vi "main 1.18.vi"() -> ()   [LabVIEW 2020]
uses:
  subvi/Newport ESP301/Newport ESP301.lvlib
  subvi/sp_manip.llb/sp_manip_lib.lvlib
  subvi/sp_manip.llb/tcp_gateway.lvlib
  <vilib>/Utility/file.llb/Write Delimited Spreadsheet (DBL).vi
  <vilib>/Analysis/NI_AALBase.lvlib
  <vilib>/Analysis/1siggen.llb/Ramp Pattern by Samples.vi
  <vilib>/Analysis/NI_AALPro.lvlib
  <vilib>/Analysis/_algsub.llb/Real Vector Norm.vi
  subvi/ZaberTSeries/ZaberTSeries.lvlib
  <vilib>/Utility/file.llb/Write Delimited Spreadsheet (string).vi
  <userlib>/caLab/Private/Get_PV.vi
  <userlib>/caLab/Private/Put_DBL_PV.vi
  <vilib>/Utility/file.llb/Read Delimited Spreadsheet (string).vi
  subvi/ProdigyRemoteControlLib/ProdigyRemoteControl.lvlib
  <vilib>/DAQmx/create/channels.llb/DAQmx Create Channel (DI-Digital Input).vi
panel:
  out "Pics L":i32=200
  out "Waveform Chart":dbl(graph)
  out "G2 X":cluster{dbl[], "Ramp Pattern":dbl[]}(graph)={array[344 elements], "Ramp Pattern"=[0.0, 0.0, 0.0, 0.0, 0.0, 0.0, 0.0, 0.0, 0.0, 0.0, 0.0, 0.0, 0.0, 0.0, 0.0, 0.0, 0.0, 0.0, 0.0, 0.0, 0.0, 12.377241379310345, 41.64689655172414, 18.335172413793103, 0.0, 0.0, 0.0, 0.0, 0.0, 0.0, 0.0, 0.0, 0.0, 0.0, 0.0, 0.0, 0.0, 0.0, 0.0, 0.0, 0.0, 0.0, 0.0, 0.0, 0.0, 0.0, 0.0, 0.0, 0.0, 0.0, 0.0, 0.0, 0.0, 0.0, 0.0, 0.0, 0.0, 0.0, 0.0, 0.0, 0.0, 0.0, 0.0, 0.0, 0.0, 0.0, 0.0, 0.0, 0.0, 0.0, 0.0, 0.0, 0.0, 0.0, 0.0, 0.0, 0.0, 0.0, 0.0, 0.0, 0.0, 0.0, 0.0, 0.0, 0.0, 0.0, 0.0, 0.0, 0.0, 0.0, 0.0, 0.0, 0.0, 0.0, 0.0, 0.0, 0.0, 0.0, 0.0, 0.0, 0.0, 0.0, 0.0, 0.0, 0.0, 0.0, 0.0, 0.0, 0.0, 0.0, 0.0, 0.0, 0.0, 0.0, 0.0, 17.495517241379314, 48.13413793103449, 27.429999999999996, 0.0, 0.0, 0.0, 0.0, 0.0, 0.0, 0.0, 0.0, 0.0, 0.0, 0.0, 0.0, 0.0, 0.0, 0.0, 0.0, 0.0, 0.0, 0.0, 0.0, 0.0, 0.0, 0.0, 0.0, 0.0, 0.0, 0.0, 0.0, 0.0, 0.0, 0.0, 0.0, 0.0, 0.0, 0.0, 0.0, 0.0, 0.0, 0.0, 0.0, 0.0, 0.0, 0.0, 0.0, 0.0, 0.0, 0.0, 0.0, 0.0, 0.0, 0.0, 0.0, 0.0, 0.0, 0.0, 0.0, 0.0, 0.0, 0.0, 0.0, 0.0, 0.0, 0.0, 0.0, 17.760344827586206, 28.923448275862068, 17.532068965517244, 0.0, 0.0, 0.0, 0.0, 0.0, 0.0, 0.0, 0.0, 0.0, 0.0, 0.0, 0.0, 0.0, 0.0, 0.0, 0.0, 0.0, 0.0, 0.0, 0.0, 0.0, 0.0, 0.0, 0.0, 0.0, 0.0, 0.0, 0.0, 0.0, 0.0, 0.0, 0.0, 0.0, 0.0, 0.0, 0.0, 0.0, 0.0, 0.0, 0.0, 0.0, 0.0, 0.0, 0.0, 0.0, 2.201724137931034, 1.9948275862068956, 0.0, 0.0, 0.0, 0.0, 0.0, 0.0, 0.0, 0.0, 0.0, 0.0, 0.0, 0.0, 0.0, 0.0, 0.0, 0.0, 0.0, 0.0, 0.0, 0.0, 0.0, 0.0, 0.0, 0.0, 0.0, 0.0, 0.0, 0.0, 0.0, 0.0, 0.0, 0.0, 0.0, 0.0, 0.0, 0.0, 0.0, 0.0, 0.0, 0.0, 0.0, 0.0, 0.0, 0.0, 0.0, 0.0, 0.0, 0.0, 0.0, 0.0, 0.0, 0.0, 0.0, 0.0, 0.0, 0.0, 0.0, 0.0, 0.0, 0.0, 0.0, 0.0, 0.0, 0.0, 0.0, 0.0, 0.0, 0.0, 0.0, 0.0, 0.0, 0.0, 0.0, 0.0, 0.0, 0.0, 0.0, 0.0, 0.0, 0.0, 0.0, 0.0, 0.0, 0.0, 0.0, 0.0, 0.0, 0.0, 0.0, 0.0, 0.0, 0.0, 0.0, 0.0, 0.0, 0.0, 0.0, 0.0, 0.0, 0.0, 0.0, 0.0, 0.0, 0.0, 0.0, 0.0, 0.0, 0.0, 0.0, 0.0, 0.0, 0.0]}
  in  "reset every n pics":bool=TRUE
  in  "pics2avg":i32=50
  in  "abort acq.":bool
  out "G2 Y":cluster{dbl[], "Ramp Pattern":dbl[]}(graph)={[0.0, 0.0, 0.0, 0.0, 0.0, 0.0, 0.0, 0.0, 0.0, 0.0, 0.0, 0.0, 0.0, 0.0, 0.0, 0.0, 0.0, 0.0, 0.0, 0.0, 0.0, 0.0, 0.0, 0.0, 0.0, 0.0, 0.0, 0.0, 0.0, 0.0, 0.0, 0.0, 0.0, 0.0, 0.0, 0.0, 0.0, 0.0, 0.0, 0.0, 0.0, 0.0, 0.0, 0.0, 0.0, 0.0, 0.0, 0.0, 0.0, 0.0, 0.0, 0.0, 0.0, 0.0, 0.0, 0.0, 0.0, 0.0, 0.0, 0.0, 0.0, 0.0, 0.0, 0.0, 0.0, 0.0, 0.0, 0.0, 0.0, 0.0, 0.0, 0.0, 0.0, 0.0, 0.0, 0.0, 0.0, 0.0, 0.0, 0.0, 0.0, 0.0, 0.0, 0.0, 0.0, 0.0, 0.0, 0.0, 0.0, 0.0, 0.0, 0.0, 0.0, 0.0, 0.0, 0.0, 0.0, 0.0, 0.0, 0.0, 0.0, 0.0, 0.0, 0.0, 0.0, 0.0, 0.0, 0.0, 0.0, 0.0, 0.0, 0.0, 0.0, 0.0, 0.0, 0.0, 0.0, 0.0, 0.0, 0.0, 0.0, 0.0, 0.0, 0.0, 0.0, 0.0, 0.0, 0.0, 0.0, 0.0, 0.0, 0.0, 0.0, 0.0, 0.0, 0.0, 0.0, 0.0, 0.0, 0.0, 0.0, 0.0, 0.0, 0.0, 0.0, 0.0, 0.0, 0.0, 0.0, 0.0, 0.0, 0.0, 0.0, 0.0, 0.0, 0.0, 0.0, 0.0, 0.0, 0.0, 0.0, 0.0, 0.0, 0.0, 0.0, 0.0, 0.0, 0.0, 0.0, 0.0, 0.0, 0.0, 0.0, 0.0, 0.0, 0.0, 0.0, 0.0, 0.0, 0.0, 0.0, 0.0, 0.0, 0.0, 0.0, 0.0, 0.0, 0.0, 0.0, 0.0, 0.0, 0.0, 0.0, 0.0, 0.0, 0.0, 0.0, 0.0, 0.0, 0.0, 0.0, 0.0, 0.0, 0.0, 0.0, 0.0, 0.0, 0.0, 0.0, 0.0, 0.0, 0.0, 0.0, 0.0, 0.0, 0.0, 0.0, 0.0, 0.0, 0.0, 0.0, 0.0, 0.0, 0.0, 0.0, 0.0, 0.0, 0.0, 0.0, 0.0, 0.0, 0.0, 0.0, 0.0, 0.0, 0.0, 0.0, 0.0, 0.0, 0.0, 0.0, 0.0, 0.0, 0.0, 0.0, 0.0, 0.0, 0.0, 0.0, 0.0, 0.0, 0.0, 0.0, 0.0, 0.0, 0.0], "Ramp Pattern"=[0.0, 1.003921568627451, 2.007843137254902, 3.011764705882353, 4.015686274509804, 5.019607843137255, 6.023529411764706, 7.027450980392157, 8.031372549019608, 9.035294117647059, 10.03921568627451, 11.04313725490196, 12.047058823529412, 13.050980392156863, 14.054901960784314, 15.058823529411764, 16.062745098039215, 17.066666666666666, 18.070588235294117, 19.07450980392157, 20.07843137254902, 21.08235294117647, 22.08627450980392, 23.090196078431372, 24.094117647058823, 25.098039215686274, 26.101960784313725, 27.105882352941176, 28.109803921568627, 29.113725490196078, 30.11764705882353, 31.12156862745098, 32.12549019607843, 33.129411764705885, 34.13333333333333, 35.13725490196079, 36.141176470588235, 37.14509803921569, 38.14901960784314, 39.15294117647059, 40.15686274509804, 41.16078431372549, 42.16470588235294, 43.168627450980395, 44.17254901960784, 45.1764705882353, 46.180392156862744, 47.1843137254902, 48.188235294117646, 49.1921568627451, 50.19607843137255, 51.2, 52.20392156862745, 53.207843137254905, 54.21176470588235, 55.21568627450981, 56.219607843137254, 57.22352941176471, 58.227450980392156, 59.23137254901961, 60.23529411764706, 61.23921568627451, 62.24313725490196, 63.247058823529414, 64.25098039215686, 65.25490196078431, 66.25882352941177, 67.26274509803922, 68.26666666666667, 69.27058823529411, 70.27450980392157, 71.27843137254902, 72.28235294117647, 73.28627450980392, 74.29019607843138, 75.29411764705883, 76.29803921568627, 77.30196078431372, 78.30588235294118, 79.30980392156863, 80.31372549019608, 81.31764705882352, 82.32156862745099, 83.32549019607843, 84.32941176470588, 85.33333333333333, 86.33725490196079, 87.34117647058824, 88.34509803921569, 89.34901960784313, 90.3529411764706, 91.35686274509804, 92.36078431372549, 93.36470588235294, 94.3686274509804, 95.37254901960785, 96.37647058823529, 97.38039215686274, 98.3843137254902, 99.38823529411765, 100.3921568627451, 101.39607843137254, 102.4, 103.40392156862745, 104.4078431372549, 105.41176470588235, 106.41568627450981, 107.41960784313726, 108.4235294117647, 109.42745098039215, 110.43137254901961, 111.43529411764706, 112.43921568627451, 113.44313725490196, 114.44705882352942, 115.45098039215686, 116.45490196078431, 117.45882352941176, 118.46274509803922, 119.46666666666667, 120.47058823529412, 121.47450980392156, 122.47843137254903, 123.48235294117647, 124.48627450980392, 125.49019607843137, 126.49411764705883, 127.49803921568628, 128.50196078431372, 129.50588235294117, 130.50980392156862, 131.51372549019607, 132.51764705882354, 133.521568627451, 134.52549019607844, 135.52941176470588, 136.53333333333333, 137.53725490196078, 138.54117647058823, 139.54509803921567, 140.54901960784315, 141.5529411764706, 142.55686274509804, 143.5607843137255, 144.56470588235294, 145.5686274509804, 146.57254901960783, 147.57647058823528, 148.58039215686276, 149.5843137254902, 150.58823529411765, 151.5921568627451, 152.59607843137255, 153.6, 154.60392156862744, 155.6078431372549, 156.61176470588236, 157.6156862745098, 158.61960784313726, 159.6235294117647, 160.62745098039215, 161.6313725490196, 162.63529411764705, 163.6392156862745, 164.64313725490197, 165.64705882352942, 166.65098039215687, 167.65490196078431, 168.65882352941176, 169.6627450980392, 170.66666666666666, 171.6705882352941, 172.67450980392158, 173.67843137254903, 174.68235294117648, 175.68627450980392, 176.69019607843137, 177.69411764705882, 178.69803921568626, 179.7019607843137, 180.7058823529412, 181.70980392156864, 182.71372549019608, 183.71764705882353, 184.72156862745098, 185.72549019607843, 186.72941176470587, 187.73333333333332, 188.7372549019608, 189.74117647058824, 190.7450980392157, 191.74901960784314, 192.75294117647059, 193.75686274509803, 194.76078431372548, 195.76470588235293, 196.7686274509804, 197.77254901960785, 198.7764705882353, 199.78039215686275, 200.7843137254902, 201.78823529411764, 202.7921568627451, 203.79607843137254, 204.8, 205.80392156862746, 206.8078431372549, 207.81176470588235, 208.8156862745098, 209.81960784313725, 210.8235294117647, 211.82745098039214, 212.83137254901962, 213.83529411764707, 214.8392156862745, 215.84313725490196, 216.8470588235294, 217.85098039215686, 218.8549019607843, 219.85882352941175, 220.86274509803923, 221.86666666666667, 222.87058823529412, 223.87450980392157, 224.87843137254902, 225.88235294117646, 226.8862745098039, 227.89019607843136, 228.89411764705883, 229.89803921568628, 230.90196078431373, 231.90588235294118, 232.90980392156862, 233.91372549019607, 234.91764705882352, 235.92156862745097, 236.92549019607844, 237.9294117647059, 238.93333333333334, 239.93725490196078, 240.94117647058823, 241.94509803921568, 242.94901960784313, 243.95294117647057, 244.95686274509805, 245.9607843137255, 246.96470588235294, 247.9686274509804, 248.97254901960784, 249.9764705882353, 250.98039215686273, 251.98431372549018, 252.98823529411766, 253.9921568627451, 254.99607843137255, 256.0]}
  out "ETA":timestamp=timestamp(3655133644.4615793 s since 1904-01-01) format="%<%H:%M:%S>T"
  out "acq. imgs":i32=200
  out "snap_prog":dbl(slide)=1.0 scale=0.0..1.0
  in  "BasePath":path=path "T:/trARPES/PESData"
  in  "cam_liveavg":bool=TRUE caption="live average"
  out "cam_fps":dbl=19.690658487387566 caption="FPS" format="%.1g"
  out "sideimg":dbl[][](graph)
  out "RunNumber":u16=3091
  out "sum":dbl format="%#.2g"
  out "max":dbl=22.774482758620692
  out "mainimg":dbl[][](graph)
  out "ESP_con?":bool=TRUE caption="ESP301"
  out "phoib_con?":bool caption="PHOIBOS"
  out "manip_con?":bool=TRUE caption="manipulator"
  out "cam_con?":bool caption="camera"
  in  "main_close":bool=TRUE
  in  "Tab Control":enum32{"live", "scan", "devices"}(tab)=enum."devices"
  in  "wattpilot_set":bool
  out "Readback_wattpilot":dbl=304.89
  in  "Set Powet (%)":dbl
  out "Readback":dbl=340.0
  out "In Range":bool
  in  "setpoint_set":bool
  in  "Setpoint":dbl=302.0
  out "TB":dbl=304.91
  out "TA":dbl=304.49
  in  "phoib_I_10s":dbl
  out "phoib_I_10":dbl caption="Mesh Back"
  in  "mirr_go":bool
  in  "ESP_opent0file":bool
  in  "mirr_rel":i32=1 caption="relative [steps]"
  in  "mirr_Y-":bool
  in  "mirr_Y+":bool
  in  "mirr_X+":bool
  in  "mirr_X-":bool
  in  "manip_deltas":dbl[](array[numeric])=[0.0, 0.0, 5.0, 0.0, 0.0, 0.0] caption="delta" format="%#.5g"
  in  "aq.mode":enum32{"Radio Selection 1", "Radio Selection 2"}(radio)=enum."Radio Selection 2"
  in  "dark avg":i32=100
  in  "cam_avgs":i32=20 caption="N"
  in  "ESP_delta":dbl caption="relative [mm]"
  in  "ESP_-":bool
  in  "ESP_+":bool
  in  "ESP_go":bool
  in  "ESP_dest_t":dbl=728236.1319443199 caption="[fs]"
  in  "ESP_dest":dbl=-35.84015 caption="[mm]"
  in  "ESP_set_t0":bool
  in  "phoib_I_6s":dbl=3200.0
  in  "phoib_I_5s":dbl=1700.0
  in  "phoib_I_4s":dbl=4.558
  in  "phoib_I_3s":dbl=-10.0
  in  "phoib_I_2s":dbl=35.0
  in  "phoib_I_1s":dbl=21.0
  in  "phoib_standby":bool
  in  "phoib_set":bool
  out "phoib_I_6":dbl=3200.0 caption="Screen Voltage"
  out "phoib_I_5":dbl=1500.0 caption="Detctor Voltage"
  out "phoib_I_4":dbl=4.558 caption="Work Function"
  out "phoib_I_3":dbl=-10.0 caption="Coil Current"
  out "phoib_I_2":dbl=35.0 caption="Pass Energy"
  out "phoib_I_1":dbl=21.0 caption="Kinetic Energy"
  out "Saved Positions":string[][](table)=[["ertwertwert", "-2.299945", "-2.030214", "38.900024", "50.000762", "0.000887", "-97.998082"], ["uztgugt", "-14.999451", "-13.638894", "442.380066", "13.998380", "-1.893758", "-76.305838"], ["asdf", "-14.999451", "-13.638894", "442.380066", "13.998380", "-1.893758", "-76.305838"], ["test3", "-14.999451", "-13.638894", "441.380066", "13.998380", "-1.893758", "-76.305838"]]
  in  "Save Pos":bool
  in  "Load":bool
  in  "Delete":bool
  in  "ManipRel +":bool
  in  "ManipRel -":bool
  in  "Move Abs":bool
  in  "stop manip":bool
  in  "dest":dbl[](array[numeric])=[1.794011231344732, -4.007411134769244, 35.099853515625, 337.9843004481455, 2.0, 140.61656469713384] caption="destination" format="%#.5g"
  out "axis":string[](array[string])=["x", "y", "z", "polar", "tilt", "azimut"]
  out "pos":dbl[](array[numeric])=[1.794011231344732, -4.007411134769244, 35.099853515625, 337.9843004481455, 1.998632949125299, 140.61656469713384] caption="position" format="%.5f"
  out "ESP_pos":dbl=-35.84015 caption="Position"
  out "ESP_delay":dbl=-0.3335640952092252 caption="Delay"
  out "ESP_t0":dbl=-35.8401 caption="Time Zero @"
  out "phoib_I_7":dbl=-30.0 caption="Conversion Voltage"
  in  "phoib_I_7s":dbl=-30.0
  in  "phoib_I_8s":dbl=0.0039
  in  "phoib_I_9s":dbl
  out "phoib_I_8":dbl=0.0039 caption="FD1"
  out "phoib_I_9":dbl caption="Mesh Front"
  in  "gain":bool
  in  "cam_exp":u32=50 caption="exposure [ms]"
  in  "binning":u16(ring)=2 items=["X 1", "X 2", "X 4", "X 8"]
  in  "cam_dark?":bool=TRUE caption="subtract dark?"
  in  "cam_dark":bool
  in  "cam_saveimg":bool
  in  "e-size":u8
  in  "lower threshold":i32=20
  in  "count?":bool
  in  "ROI Left":i32=1
  in  "ROI Right":i32=43
  in  "ROI Top":i32=1
  in  "ROI Bottom":i32=33
  out "moving?":bool[](array[boolean])
  out "mirr_posX":i32=1955 caption="X"
  out "mirr_posY":i32=2950 caption="Y"
  in  "mirr_dest":i32[](array[numeric])=[60782, 121383]
  out "waveplate position":dbl format="%.6g"
  out "stage2 position":dbl format="%.6g"
  in  "lens_mode":string(combo)
  in  "scan_range":string(combo)
  out "current scan 2":i32=3
  out "scan 1":dbl(slide)=1.0 scale=0.0..1.0
  in  "Tab Control 2":enum32{"setup", "data"}(tab)=enum."data"
  in  "scan_selector 2":T1(tab)
  in  "scan_manip_start 2":dbl[](array[numeric])=[1.794011231344732, -4.007411134769244, 35.099853515625, 337.9843004481455, 2.000390761745462, 140.61656469713384] caption="start position" format="%#.5g"
  in  "scan_manip_deltas 2":dbl[](array[numeric])=[0.0, 0.0, 0.0, 0.0, 1.0, 0.0] caption="direction vector\n(gets normalized)" format="%#.5g"
  in  "scan_manip_setstart 2":bool
  in  "scan_mirr_start 2":i32[](array[numeric])=[60782, 121383] caption="scan_mirr_start"
  in  "scan_mirr_deltas 2":i32[](array[numeric])=[1, 0] caption="direction vector\n(gets normalized)"
  in  "scan_mirr_setstart 2":bool
  in  "wait addional  2":dbl caption="s"
  in  "Wait for T 2":bool=TRUE
  in  "scan_volt_parameter 2":string(combo)="Kinetic Energy"
  in  "waypointsD2":string[][](table)
  in  "waypointsD1":string[][](table)=[["302", "1"], ["304", ""], ["", ""]]
  in  "load waypoints 1":bool
  in  "meas_iter":i32=1 caption="Iterations"
  in  "scan_selector":T1(tab)=enum."delay"
  in  "scan_manip_setstart":bool
  in  "scan_manip_start":dbl[](array[numeric])=[1.794011231344732, -4.007411134769244, 35.099853515625, 337.9843004481455, 2.000390761745462, 140.61656469713384] caption="start position" format="%#.5g"
  in  "scan_manip_deltas":dbl[](array[numeric])=[0.0, 0.0, 0.0, 0.0, 1.0, 0.0] caption="direction vector\n(gets normalized)" format="%#.5g"
  in  "scan_mirr_start":i32[](array[numeric])=[60782, 121383]
  in  "scan_mirr_deltas":i32[](array[numeric])=[1, 0] caption="direction vector\n(gets normalized)"
  in  "scan_mirr_setstart":bool
  in  "wait addional":dbl caption="s"
  in  "Wait for T":bool=TRUE
  in  "scan_volt_parameter":string(combo)="Kinetic Energy"
  in  "clear waypoints 1":bool
  in  "load waypoints 2":bool
  in  "clear waypoints 2":bool
  out "intensitygraph":cluster{"Array":dbl[], "Intensity Chart":dbl[]}(graph)={"Array"=[302.0, 303.0, 304.0], "Intensity Chart"=[1937.88, 12704.590000000002, 4640.840000000001]}
  out "energygraph":dbl[][](graph)=[[0.0, 0.0, 0.0, 64.28999999999999, 120.06, 0.0, 0.0, 0.0, 0.0, 0.0, 0.0, 0.0, 0.0, 0.0, 0.0, 0.0, 0.0, 0.0, 0.0, 0.0, 0.0, 0.0, 0.0, 0.0, 0.0, 0.0, 0.0, 0.0, 0.0, 0.0, 0.0, 0.0, 0.0, 0.0, 0.0, 0.0, 0.0, 0.0, 0.0, 0.0, 0.0, 0.0, 0.0, 0.0, 0.0, 0.0, 0.0, 0.0, 0.0, 384.53999999999996, 1103.3799999999999, 448.21000000000004, 0.0, 0.0, 0.0, 0.0, 0.0, 0.0, 0.0, 0.0, 0.0, 0.0, 0.0, 0.0, 0.0, 0.0, 0.0, 0.0, 0.0, 120.82, 0.0, 261.04, 195.1, 253.87, 199.70999999999998, 127.75, 87.50999999999999, 0.0, 52.54, 0.0, 0.0, 51.78, 55.73, 0.0, 0.0, 0.0, 0.0, 0.0, 0.0, 0.0, 0.0, 0.0, 0.0, 0.0, 0.0, 0.0, 0.0, 0.0, 0.0, 0.0, 0.0, 0.0, 0.0, 0.0, 0.0, 0.0, 0.0, 0.0, 0.0, 0.0, 0.0, 0.0, 0.0, 332.90999999999997, 1106.25, 934.74, 0.0, 156.76, 62.65, 0.0, 0.0, 0.0, 0.0, 0.0, 0.0, 54.62, 0.0, 0.0, 0.0, 0.0, 0.0, 0.0, 0.0, 0.0, 0.0, 0.0, 0.0, 0.0, 0.0, 0.0, 0.0, 0.0, 0.0, 0.0, 65.85, 165.75, 0.0, 0.0, 0.0, 0.0, 0.0, 0.0, 0.0, 0.0, 0.0, 0.0, 0.0, 0.0, 0.0, 0.0, 0.0, 0.0, 0.0, 266.63, 591.5, 261.64, 0.0, 391.9, 527.29, 82.87, 123.75, 286.74, 151.72, 0.0, 0.0, 0.0, 0.0, 0.0, 0.0, 0.0, 0.0, 0.0, 0.0, 0.0, 0.0, 0.0, 0.0, 0.0, 0.0, 0.0, 0.0, 0.0, 396.37, 721.0900000000001, 353.5, 83.97999999999999, 104.77000000000001, 0.0, 57.83, 60.98, 182.28, 128.78, 0.0, 0.0, 0.0, 465.25, 624.3399999999999, 348.62, 0.0, 0.0, 0.0, 0.0, 0.0, 0.0, 0.0, 0.0, 0.0, 0.0, 0.0, 0.0, 119.7, 217.91, 120.56, 0.0, 0.0, 0.0, 0.0, 0.0, 0.0, 0.0, 58.89, 0.0, 0.0, 0.0, 202.23999999999998, 149.79000000000002, 0.0, 117.82, 212.51999999999998, 534.74, 421.98, 50.97, 0.0, 0.0, 0.0, 0.0, 362.15999999999997, 656.04, 265.02, 0.0, 0.0, 0.0, 0.0, 0.0, 0.0, 0.0, 0.0, 0.0, 0.0, 0.0, 0.0, 0.0, 0.0, 0.0, 0.0, 0.0, 0.0, 0.0, 0.0, 0.0, 0.0, 0.0, 0.0, 0.0, 0.0, 0.0, 0.0, 0.0, 0.0, 0.0, 0.0, 0.0, 0.0, 0.0, 0.0, 0.0, 0.0, 0.0, 0.0, 0.0, 0.0, 0.0, 0.0, 0.0, 0.0, 0.0, 0.0, 0.0, 0.0, 0.0, 0.0, 0.0, 0.0, 0.0, 0.0, 0.0, 0.0, 0.0, 0.0, 0.0, 0.0, 0.0, 0.0, 237.67999999999998, 286.08, 130.9, 0.0, 0.0, 0.0, 0.0, 0.0, 0.0, 0.0, 0.0, 0.0, 0.0, 0.0, 0.0, 0.0, 0.0, 0.0, 0.0, 0.0, 0.0, 0.0, 0.0, 0.0, 0.0, 0.0, 0.0, 0.0, 0.0, 0.0, 0.0], [0.0, 0.0, 0.0, 0.0, 0.0, 0.0, 0.0, 0.0, 0.0, 0.0, 0.0, 0.0, 0.0, 0.0, 0.0, 0.0, 0.0, 485.13, 1279.2, 234.71, 0.0, 0.0, 0.0, 0.0, 0.0, 0.0, 0.0, 0.0, 0.0, 0.0, 0.0, 0.0, 50.5, 654.4200000000001, 511.98, 0.0, 0.0, 0.0, 0.0, 0.0, 0.0, 0.0, 0.0, 0.0, 0.0, 0.0, 0.0, 0.0, 0.0, 0.0, 0.0, 0.0, 0.0, 0.0, 0.0, 0.0, 0.0, 0.0, 63.72, 693.84, 574.54, 0.0, 0.0, 0.0, 68.68, 1054.28, 1010.9499999999999, 0.0, 0.0, 0.0, 0.0, 0.0, 0.0, 0.0, 0.0, 0.0, 0.0, 0.0, 56.57, 971.76, 1333.73, 330.0, 0.0, 0.0, 0.0, 0.0, 0.0, 349.33000000000004, 292.7, 0.0, 0.0, 0.0, 0.0, 0.0, 0.0, 82.77000000000001, 1059.23, 1069.87, 156.47, 0.0, 0.0, 0.0, 0.0, 293.91, 333.47, 551.4, 493.64, 73.72999999999999, 0.0, 0.0, 0.0, 0.0, 0.0, 0.0, 0.0, 0.0, 0.0, 0.0, 0.0, 0.0, 0.0, 0.0, 286.01, 543.0699999999999, 251.94, 0.0, 0.0, 0.0, 0.0, 0.0, 233.63, 968.4799999999999, 771.53, 109.94, 0.0, 123.07, 499.72999999999996, 431.4, 0.0, 0.0, 60.85, 69.5, 0.0, 0.0, 0.0, 0.0, 0.0, 0.0, 0.0, 0.0, 0.0, 0.0, 0.0, 0.0, 0.0, 0.0, 52.01, 0.0, 0.0, 0.0, 0.0, 0.0, 0.0, 0.0, 0.0, 0.0, 0.0, 0.0, 0.0, 0.0, 0.0, 0.0, 0.0, 0.0, 0.0, 0.0, 0.0, 0.0, 0.0, 0.0, 0.0, 0.0, 0.0, 0.0, 0.0, 0.0, 0.0, 0.0, 0.0, 0.0, 52.95, 478.8, 870.47, 572.83, 61.67, 268.19, 1143.4, 1804.2599999999998, 1145.6100000000001, 739.22, 904.59, 1109.3000000000002, 1233.6599999999999, 212.92, 0.0, 0.0, 105.95, 448.76000000000005, 1306.3500000000001, 1005.5900000000001, 68.8, 0.0, 57.94, 0.0, 0.0, 0.0, 0.0, 0.0, 0.0, 0.0, 0.0, 0.0, 0.0, 0.0, 0.0, 0.0, 0.0, 0.0, 0.0, 0.0, 0.0, 0.0, 0.0, 0.0, 0.0, 0.0, 0.0, 159.01, 520.94, 925.5600000000001, 1641.53, 2261.26, 1259.83, 0.0, 0.0, 0.0, 0.0, 0.0, 0.0, 136.69, 398.81, 382.02, 0.0, 0.0, 0.0, 0.0, 0.0, 0.0, 421.01, 1376.5800000000002, 1425.75, 268.07, 0.0, 345.84000000000003, 396.77, 0.0, 0.0, 0.0, 0.0, 0.0, 216.93, 727.65, 830.9, 774.2299999999999, 839.3900000000001, 309.97, 0.0, 0.0, 0.0, 0.0, 0.0, 0.0, 0.0, 100.57, 459.66, 305.86, 0.0, 0.0, 0.0, 0.0, 0.0, 0.0, 0.0, 0.0, 0.0, 0.0, 0.0, 0.0, 0.0, 0.0, 0.0, 0.0, 0.0, 0.0, 0.0, 0.0, 0.0, 0.0, 0.0, 0.0, 0.0, 64.97999999999999, 379.62, 337.15999999999997, 83.6, 463.66, 399.03999999999996, 0.0, 0.0, 0.0, 0.0, 0.0, 0.0, 0.0, 0.0, 0.0, 0.0, 0.0, 0.0, 0.0, 0.0, 0.0, 0.0, 0.0, 0.0, 0.0, 0.0, 0.0, 0.0, 0.0, 0.0, 0.0, 0.0, 0.0], [0.0, 0.0, 0.0, 0.0, 0.0, 0.0, 0.0, 0.0, 0.0, 0.0, 0.0, 0.0, 0.0, 0.0, 0.0, 165.83, 124.99, 78.27000000000001, 0.0, 0.0, 0.0, 765.77, 1457.88, 293.67, 0.0, 0.0, 0.0, 0.0, 0.0, 0.0, 0.0, 0.0, 0.0, 0.0, 0.0, 0.0, 0.0, 0.0, 0.0, 0.0, 0.0, 0.0, 0.0, 0.0, 0.0, 0.0, 0.0, 0.0, 0.0, 85.5, 116.32, 0.0, 0.0, 0.0, 0.0, 0.0, 0.0, 0.0, 0.0, 0.0, 0.0, 0.0, 0.0, 0.0, 0.0, 0.0, 0.0, 0.0, 179.01, 123.78999999999999, 64.69, 0.0, 433.57000000000005, 1457.15, 661.49, 0.0, 0.0, 0.0, 0.0, 0.0, 0.0, 171.38, 497.28999999999996, 835.47, 1797.0300000000002, 1202.25, 169.95, 0.0, 0.0, 0.0, 0.0, 383.74, 496.08, 196.89999999999998, 0.0, 0.0, 0.0, 0.0, 719.08, 1717.5100000000002, 1360.8, 163.65, 118.56, 798.75, 610.32, 0.0, 0.0, 0.0, 0.0, 73.12, 51.75, 0.0, 0.0, 0.0, 0.0, 0.0, 0.0, 0.0, 0.0, 0.0, 0.0, 0.0, 233.35000000000002, 1128.3, 1138.8400000000001, 207.43, 0.0, 0.0, 50.52, 0.0, 0.0, 0.0, 0.0, 0.0, 0.0, 0.0, 0.0, 0.0, 0.0, 0.0, 0.0, 0.0, 0.0, 0.0, 0.0, 0.0, 0.0, 0.0, 0.0, 0.0, 0.0, 122.82, 66.93, 184.87, 606.35, 1065.2, 616.33, 82.97, 0.0, 0.0, 0.0, 0.0, 0.0, 0.0, 0.0, 0.0, 0.0, 0.0, 0.0, 210.77, 369.49, 0.0, 0.0, 0.0, 0.0, 0.0, 0.0, 0.0, 0.0, 0.0, 0.0, 0.0, 0.0, 0.0, 0.0, 0.0, 0.0, 0.0, 0.0, 61.71, 492.70000000000005, 501.67999999999995, 50.9, 0.0, 0.0, 0.0, 0.0, 0.0, 0.0, 0.0, 0.0, 0.0, 0.0, 0.0, 0.0, 0.0, 0.0, 0.0, 0.0, 0.0, 0.0, 0.0, 0.0, 0.0, 0.0, 0.0, 0.0, 0.0, 0.0, 0.0, 0.0, 0.0, 0.0, 0.0, 0.0, 0.0, 0.0, 0.0, 0.0, 0.0, 0.0, 0.0, 0.0, 0.0, 0.0, 0.0, 0.0, 0.0, 0.0, 0.0, 0.0, 0.0, 0.0, 0.0, 0.0, 0.0, 0.0, 0.0, 0.0, 0.0, 0.0, 0.0, 0.0, 0.0, 0.0, 0.0, 0.0, 0.0, 0.0, 0.0, 0.0, 0.0, 0.0, 0.0, 0.0, 0.0, 0.0, 0.0, 0.0, 0.0, 191.69, 347.02, 262.31, 325.89, 168.79, 0.0, 0.0, 52.9, 53.13, 0.0, 0.0, 0.0, 0.0, 0.0, 0.0, 0.0, 0.0, 0.0, 0.0, 0.0, 0.0, 0.0, 0.0, 0.0, 0.0, 0.0, 0.0, 0.0, 0.0, 0.0, 0.0, 0.0, 0.0, 0.0, 0.0, 327.12, 491.83000000000004, 242.02999999999997, 0.0, 0.0, 0.0, 0.0, 0.0, 0.0, 0.0, 676.6, 975.77, 229.86, 0.0, 144.15, 151.75, 0.0, 0.0, 0.0, 0.0, 0.0, 0.0, 0.0, 0.0, 0.0, 0.0, 0.0, 0.0, 0.0, 0.0, 0.0, 0.0, 0.0, 0.0, 0.0, 0.0, 0.0, 0.0, 0.0]]
  out "anglegraph":dbl[][](graph)=[[0.0, 0.0, 0.0, 0.0, 0.0, 0.0, 0.0, 0.0, 0.0, 0.0, 0.0, 0.0, 0.0, 0.0, 0.0, 0.0, 0.0, 0.0, 0.0, 0.0, 0.0, 0.0, 0.0, 0.0, 0.0, 0.0, 0.0, 307.98, 204.45, 0.0, 0.0, 0.0, 0.0, 0.0, 0.0, 0.0, 0.0, 0.0, 0.0, 0.0, 0.0, 0.0, 0.0, 0.0, 0.0, 0.0, 0.0, 0.0, 0.0, 0.0, 0.0, 0.0, 0.0, 0.0, 0.0, 0.0, 0.0, 0.0, 0.0, 0.0, 0.0, 0.0, 0.0, 0.0, 0.0, 0.0, 0.0, 0.0, 0.0, 0.0, 0.0, 0.0, 0.0, 0.0, 0.0, 0.0, 0.0, 0.0, 0.0, 0.0, 0.0, 0.0, 0.0, 0.0, 0.0, 0.0, 0.0, 0.0, 0.0, 0.0, 0.0, 0.0, 0.0, 0.0, 0.0, 0.0, 0.0, 0.0, 0.0, 0.0, 0.0, 0.0, 0.0, 0.0, 0.0, 0.0, 0.0, 0.0, 0.0, 0.0, 0.0, 0.0, 0.0, 0.0, 0.0, 0.0, 0.0, 0.0, 0.0, 0.0, 0.0, 0.0, 0.0, 0.0, 0.0, 0.0, 0.0, 0.0, 0.0, 0.0, 0.0, 0.0, 0.0, 0.0, 0.0, 0.0, 0.0, 0.0, 0.0, 0.0, 0.0, 0.0, 0.0, 0.0, 0.0, 0.0, 0.0, 0.0, 0.0, 0.0, 0.0, 0.0, 0.0, 0.0, 0.0, 0.0, 640.8800000000001, 550.45, 91.89, 0.0, 0.0, 0.0, 0.0, 0.0, 0.0, 0.0, 0.0, 0.0, 0.0, 0.0, 0.0, 0.0, 0.0, 0.0, 0.0, 69.94, 60.96, 0.0, 0.0, 0.0, 0.0, 0.0, 0.0, 0.0, 0.0, 0.0, 0.0, 0.0, 0.0, 0.0, 0.0, 0.0, 0.0, 0.0, 0.0, 0.0, 115.87, 235.84, 172.04999999999998, 0.0, 0.0, 0.0, 0.0, 0.0, 0.0, 0.0, 0.0, 0.0, 0.0, 0.0, 0.0, 0.0, 0.0, 0.0, 0.0, 0.0, 0.0, 0.0, 0.0, 0.0, 0.0, 0.0, 0.0, 0.0, 0.0, 0.0, 0.0, 0.0, 0.0, 0.0, 0.0, 0.0, 0.0, 0.0, 0.0, 0.0, 0.0, 0.0, 0.0, 0.0, 0.0, 0.0, 0.0, 0.0, 0.0, 0.0, 0.0, 0.0, 0.0, 0.0, 0.0, 0.0, 0.0, 0.0, 0.0, 0.0], [0.0, 0.0, 0.0, 0.0, 0.0, 0.0, 0.0, 0.0, 0.0, 0.0, 0.0, 0.0, 0.0, 0.0, 0.0, 0.0, 54.97, 1426.6399999999999, 1312.94, 180.81, 0.0, 0.0, 0.0, 0.0, 0.0, 0.0, 0.0, 465.48, 989.61, 293.56, 0.0, 0.0, 0.0, 0.0, 0.0, 0.0, 0.0, 0.0, 0.0, 0.0, 0.0, 0.0, 0.0, 0.0, 0.0, 0.0, 0.0, 0.0, 0.0, 0.0, 0.0, 0.0, 0.0, 0.0, 0.0, 0.0, 0.0, 0.0, 0.0, 331.78, 944.91, 463.28, 0.0, 0.0, 0.0, 0.0, 143.70999999999998, 402.81, 196.09, 0.0, 0.0, 0.0, 483.82, 433.7, 0.0, 0.0, 0.0, 0.0, 0.0, 0.0, 89.85, 513.2, 263.03999999999996, 0.0, 0.0, 0.0, 0.0, 0.0, 0.0, 0.0, 0.0, 104.84, 0.0, 226.86, 214.93, 235.13, 0.0, 0.0, 0.0, 0.0, 0.0, 0.0, 0.0, 0.0, 0.0, 0.0, 0.0, 0.0, 0.0, 0.0, 0.0, 0.0, 0.0, 0.0, 0.0, 0.0, 0.0, 0.0, 0.0, 0.0, 0.0, 0.0, 0.0, 0.0, 0.0, 0.0, 0.0, 0.0, 0.0, 0.0, 0.0, 0.0, 0.0, 0.0, 0.0, 0.0, 0.0, 0.0, 0.0, 380.83, 649.96, 229.04, 0.0, 0.0, 0.0, 276.21000000000004, 441.79999999999995, 228.29, 0.0, 0.0, 0.0, 0.0, 0.0, 0.0, 0.0, 0.0, 0.0, 0.0, 0.0, 0.0, 0.0, 0.0, 0.0, 0.0, 0.0, 0.0, 0.0, 0.0, 123.92000000000002, 1311.81, 1454.81, 600.87, 0.0, 0.0, 0.0, 0.0, 0.0, 0.0, 0.0, 0.0, 0.0, 0.0, 0.0, 0.0, 0.0, 0.0, 0.0, 0.0, 0.0, 0.0, 0.0, 0.0, 0.0, 0.0, 0.0, 0.0, 0.0, 0.0, 0.0, 0.0, 0.0, 0.0, 654.53, 894.22, 410.35, 0.0, 0.0, 0.0, 0.0, 0.0, 0.0, 0.0, 0.0, 0.0, 0.0, 0.0, 0.0, 0.0, 0.0, 0.0, 0.0, 0.0, 0.0, 0.0, 0.0, 0.0, 0.0, 0.0, 0.0, 0.0, 0.0, 0.0, 0.0, 0.0, 0.0, 0.0, 0.0, 0.0, 0.0, 0.0, 0.0, 0.0, 0.0, 0.0, 0.0, 0.0, 0.0, 0.0, 0.0, 0.0, 0.0, 0.0, 0.0, 0.0, 0.0, 0.0], [0.0, 0.0, 0.0, 0.0, 0.0, 0.0, 0.0, 0.0, 0.0, 0.0, 0.0, 0.0, 0.0, 0.0, 0.0, 0.0, 0.0, 0.0, 0.0, 0.0, 0.0, 0.0, 0.0, 0.0, 0.0, 0.0, 0.0, 0.0, 0.0, 125.9, 1017.51, 504.48, 0.0, 0.0, 0.0, 0.0, 0.0, 0.0, 0.0, 0.0, 0.0, 0.0, 0.0, 0.0, 0.0, 0.0, 0.0, 0.0, 0.0, 0.0, 0.0, 0.0, 0.0, 0.0, 0.0, 0.0, 0.0, 0.0, 0.0, 0.0, 0.0, 0.0, 0.0, 0.0, 0.0, 0.0, 0.0, 0.0, 0.0, 0.0, 0.0, 0.0, 109.81, 66.88, 0.0, 0.0, 733.48, 806.32, 342.43, 0.0, 0.0, 0.0, 0.0, 0.0, 0.0, 0.0, 0.0, 0.0, 0.0, 0.0, 0.0, 0.0, 0.0, 0.0, 0.0, 0.0, 0.0, 0.0, 0.0, 0.0, 0.0, 0.0, 0.0, 0.0, 0.0, 174.07999999999998, 275.74, 429.21, 301.15999999999997, 0.0, 0.0, 0.0, 0.0, 0.0, 0.0, 0.0, 0.0, 0.0, 0.0, 0.0, 0.0, 0.0, 0.0, 0.0, 0.0, 0.0, 0.0, 0.0, 0.0, 0.0, 0.0, 0.0, 0.0, 0.0, 0.0, 0.0, 0.0, 0.0, 0.0, 0.0, 0.0, 0.0, 0.0, 0.0, 0.0, 0.0, 0.0, 0.0, 0.0, 0.0, 0.0, 0.0, 0.0, 0.0, 0.0, 0.0, 0.0, 0.0, 0.0, 0.0, 0.0, 0.0, 0.0, 0.0, 0.0, 0.0, 0.0, 0.0, 0.0, 0.0, 0.0, 0.0, 0.0, 0.0, 0.0, 252.98000000000002, 303.56, 60.91, 52.9, 53.13, 0.0, 0.0, 0.0, 0.0, 0.0, 0.0, 0.0, 0.0, 0.0, 0.0, 0.0, 0.0, 0.0, 0.0, 0.0, 0.0, 0.0, 0.0, 0.0, 0.0, 0.0, 0.0, 0.0, 0.0, 0.0, 0.0, 0.0, 0.0, 0.0, 0.0, 0.0, 0.0, 0.0, 61.05, 350.49, 266.71000000000004, 0.0, 0.0, 0.0, 0.0, 0.0, 0.0, 0.0, 0.0, 0.0, 0.0, 0.0, 0.0, 0.0, 0.0, 0.0, 0.0, 0.0, 0.0, 0.0, 0.0, 0.0, 0.0, 0.0, 0.0, 0.0, 0.0, 0.0, 0.0, 0.0, 0.0, 0.0, 0.0, 0.0, 0.0, 0.0, 0.0, 0.0, 0.0, 0.0, 0.0]]
  in  "stop after iteration":bool
  in  "time/step [s]":dbl=10.787117004394531
  out "current iteration":i32=1
  out "current scan":i32=3
  out "iteration":dbl(slide)=1.0 scale=0.0..1.0
  out "scan 2":dbl(slide)=1.0 scale=0.0..1.0
  in  "stop after step":bool
  in  "scan_go":bool
  out "measpoints":i32=3
  out "total steps":i32=3
  out "RAM [MB]":dbl=1.6590000000000003
  out "disk [MB]":dbl=1.6590000000000003
  out "duration [HH:MM:SS]":dbl=32.361351013183594 format="%<%H:%M:%S>t"
  out "ETA 2":timestamp
  in  "WattPilot EPICS chanel readback":string="trARPES:Wattpilot:PumpPercent_RBV"
  in  "WattPilot EPICS chanel set":string="trARPES:Wattpilot:PumpPercent"
  in  "ESP patch":i32[](array[numeric])=[3, 2, 1]
  in  "LS310  EPICS Heater":string="trARPES:Carving:HT-RNG"
  in  "LS310  EPICS SP":string="trARPES:Carving:TEMP"
  in  "LS310  EPICS chanel B":string="trARPES:Carving:TEMP-B"
  in  "mm/s":dbl
  in  "Set Speed to":bool
  in  "ESP Axis waveplate":i32=2 min=1 max=3
  in  "mirr_init":bool
  in  "mirr_release":bool
  in  "mirr_Y#":u8=2
  in  "manip_init":bool
  in  "manip_release":bool
  in  "phoib_init":bool
  in  "phoib_release":bool
  in  "ESP_init":bool
  in  "ESP_release":bool
  in  "ESP301 VISA":refnum<visa-resource-name>="COM8"
  in  "board number":i32
  in  "cam_init":bool
  in  "cam_release":bool
  out "cam_error":errorcluster
  out "phoib_error":errorcluster
  in  "ESP Axis delay":i32=3 min=1 max=3
  out "error out":errorcluster={"status"=FALSE, "code"=1073676418, "source"="VISA Close in Newport ESP301.lvlib:Close.vi->main 1.17a beta.vi"}
  out "error out 2":errorcluster={"status"=TRUE, "code"=1, "source"="TCP Write in sp_manip_lib.lvlib:sp_manip_disconnect.vi->main 1.17a beta.vi"}
  out "mirr_Error":errorcluster={"status"=FALSE, "code"=1073676418, "source"="VISA Close in ZaberTSeries.lvlib:Close.vi->main 1.17a beta.vi"}
  in  "mirr_VISA":refnum<visa-resource-name>="COM3"
  in  "mirr_X#":u8=1
  in  "Operating mode\nHP & QE / HS & DiCam Pro":u32=1
  in  "Frame trigger \n(High Performance and QE only)":u16
  in  "LS310  EPICS chanel A":string="trARPES:Carving:TEMP_RBV"
  in  "Status EPICS chanel":string="trARPES:Carving:TEMP-STAT"
  # "camera"
  # "analyzer"
  # "manipulator"
  # "temperature"
  # "aquisition"
  # "delay stage"
  # "Position"
  # "Destination"
  # "WattPilot"
  # "- no settings -"
  # "waypoints are absolute values"
  # "- no settings -"
  # "waypoints are absolute values"
  # "- no settings -"
  # "waypoints are absolute values"
  # "- no settings -"
  # "waypoints are absolute values"
  # "X\nY\nZ\npolar\ntilt\nazimut"
  # "waypoint \"0\" is start position"
  # "X\nY"
  # "waypoint \"0\" is start position"
  # "waypoints are absolute values"
  # "- no settings -"
  # "waypoints are absolute values"
  # "- no settings -"
  # "waypoints are absolute values"
  # "- no settings -"
  # "waypoints are absolute values"
  # "- no settings -"
  # "waypoints are absolute values"
  # "X\nY\nZ\npolar\ntilt\nazimut"
  # "waypoint \"0\" is start position"
  # "X\nY"
  # "waypoint \"0\" is start position"
  # "waypoints are absolute values"
  # "camera"
  # "phoibos"
  # "ESP301"
  # "manipulator"
  # "mirror"
  # "delay"
  # "waveplate"
  # "stage2"
  # "0 = sequential\n1 = simultaneous"
  # "0 = internal\n1 = external rising\n2 = external falling"
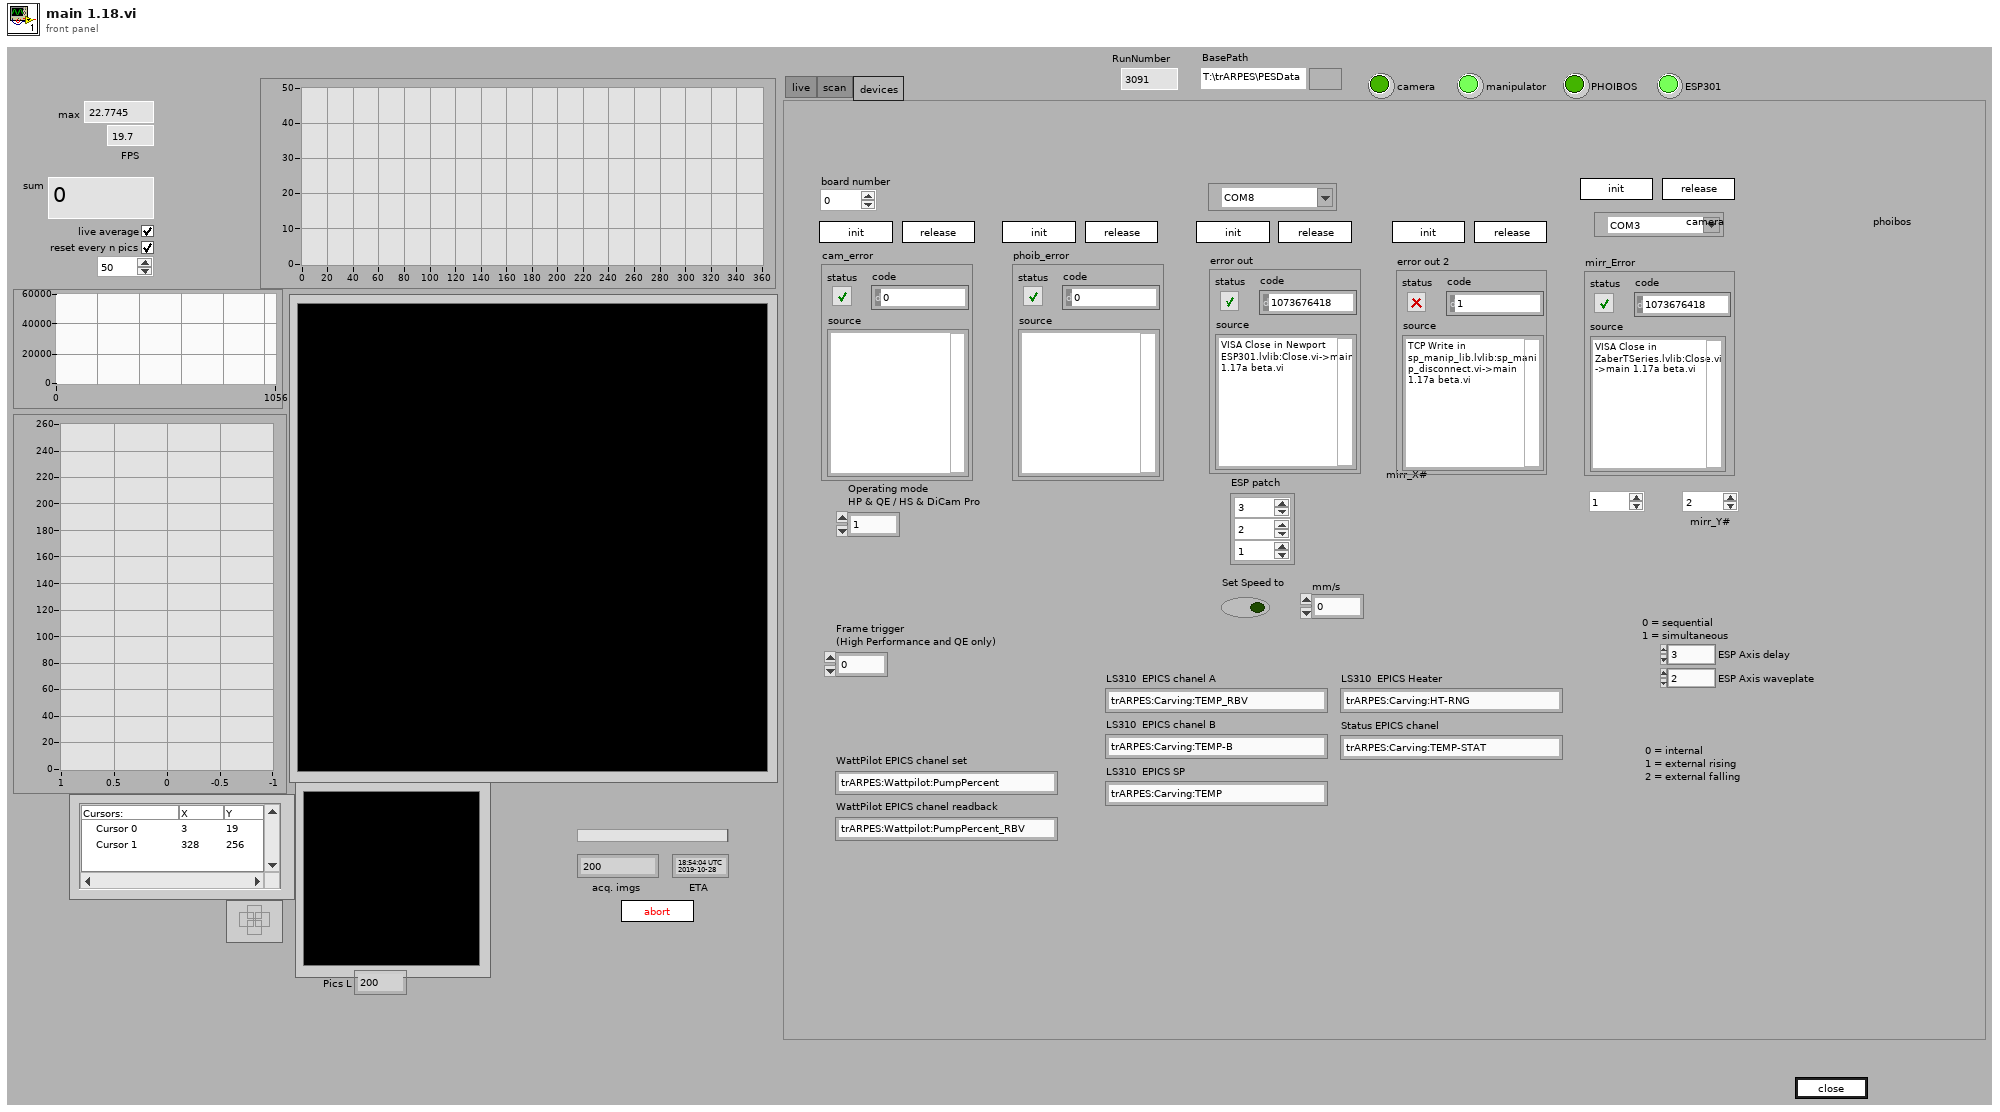
[diagram p1: front panel]
types:
  T1 = enum32{"none", "delay", "wattpilot", "waveplate", "stage2", "manipulator", "mirror", "temperature", "voltage"}
  T2 = cluster{"queue out":refnum<queue>, "queue out":refnum<queue>, "queue out":refnum<queue>, "queue out":refnum<queue>, "queue out":refnum<queue>, "queue out":refnum<queue>, "queue out":refnum<queue>}
  T3 = typedef "LVCursorListTypeDef.ctl" = cluster{"Name":string, "Color":u32, "Style":u8, "Point Style":u8, "Name Visible":bool, "Allow Drag":bool, "Cursor Mode":u32, "Plot":i32, "Index":i32, "Position":cluster{"X":dbl, "Y":dbl}, "X Scale":u32, "Y Scale":u32, "Watch Plots":i32[], "Watch All Plots":bool, "Plot Area":i32, "Label Offset":cluster{"X":dbl, "Y":dbl}}[]
  T4 = cluster{"mirr_X#":u8, "Command":u8, dbl, "Response Count":i32}
  T5 = cluster{"mirr_Y#":u8, "Command":u8, dbl, "Response Count":i32}
  T6 = cluster{i32, "Command":u8, i32, "Response Count":i32}
  T7 = cluster{"Axis_Name":string, "Axis_Type":string, "Axis_Position":dbl, "continous":bool, "moving":bool}[]
  T8 = typedef "ProdigyRemoteControl.lvlib/DEF_AnalyzerParaInfo.ctl" = cluster{"Name":string, "Type":string, "Value Type":string, "Unit":string, "Min":string, "Max":string, "Values":string}
  T9 = typedef "ProdigyRemoteControl.lvlib/DEF_SpectrumParaInfo.ctl" = cluster{"Name":string, "Value Type":string, "Unit":string, "Min":string, "Max":string, "Values":string[]}
  T10 = cluster{"Camera type":u32, "Operating mode\nHP & QE / HS & DiCam Pro ":u32, "Frame trigger \n(High Performance and QE only)":u16, "Sequence trigger":u16, "Low Light\n(QE only)":bool, "Gain":bool, "Horzontal\nbinning":u16, "Vertical\nbinning ":u16, "ROI Left":i32, "ROI Right":i32, "ROI Top":i32, "ROI Bottom":i32}
  T11 = cluster{"Name":string, "Color":u32, "Style":u8, "Point Style":u8, "Name Visible":bool, "Allow Drag":bool, "Cursor Mode":u32, "Plot":i32, "Index":i32, "Position":cluster{"X":dbl, "Y":dbl}, "X Scale":u32, "Y Scale":u32, "Watch Plots":i32[], "Watch All Plots":bool, "Plot Area":i32, "Label Offset":cluster{"X":dbl, "Y":dbl}}
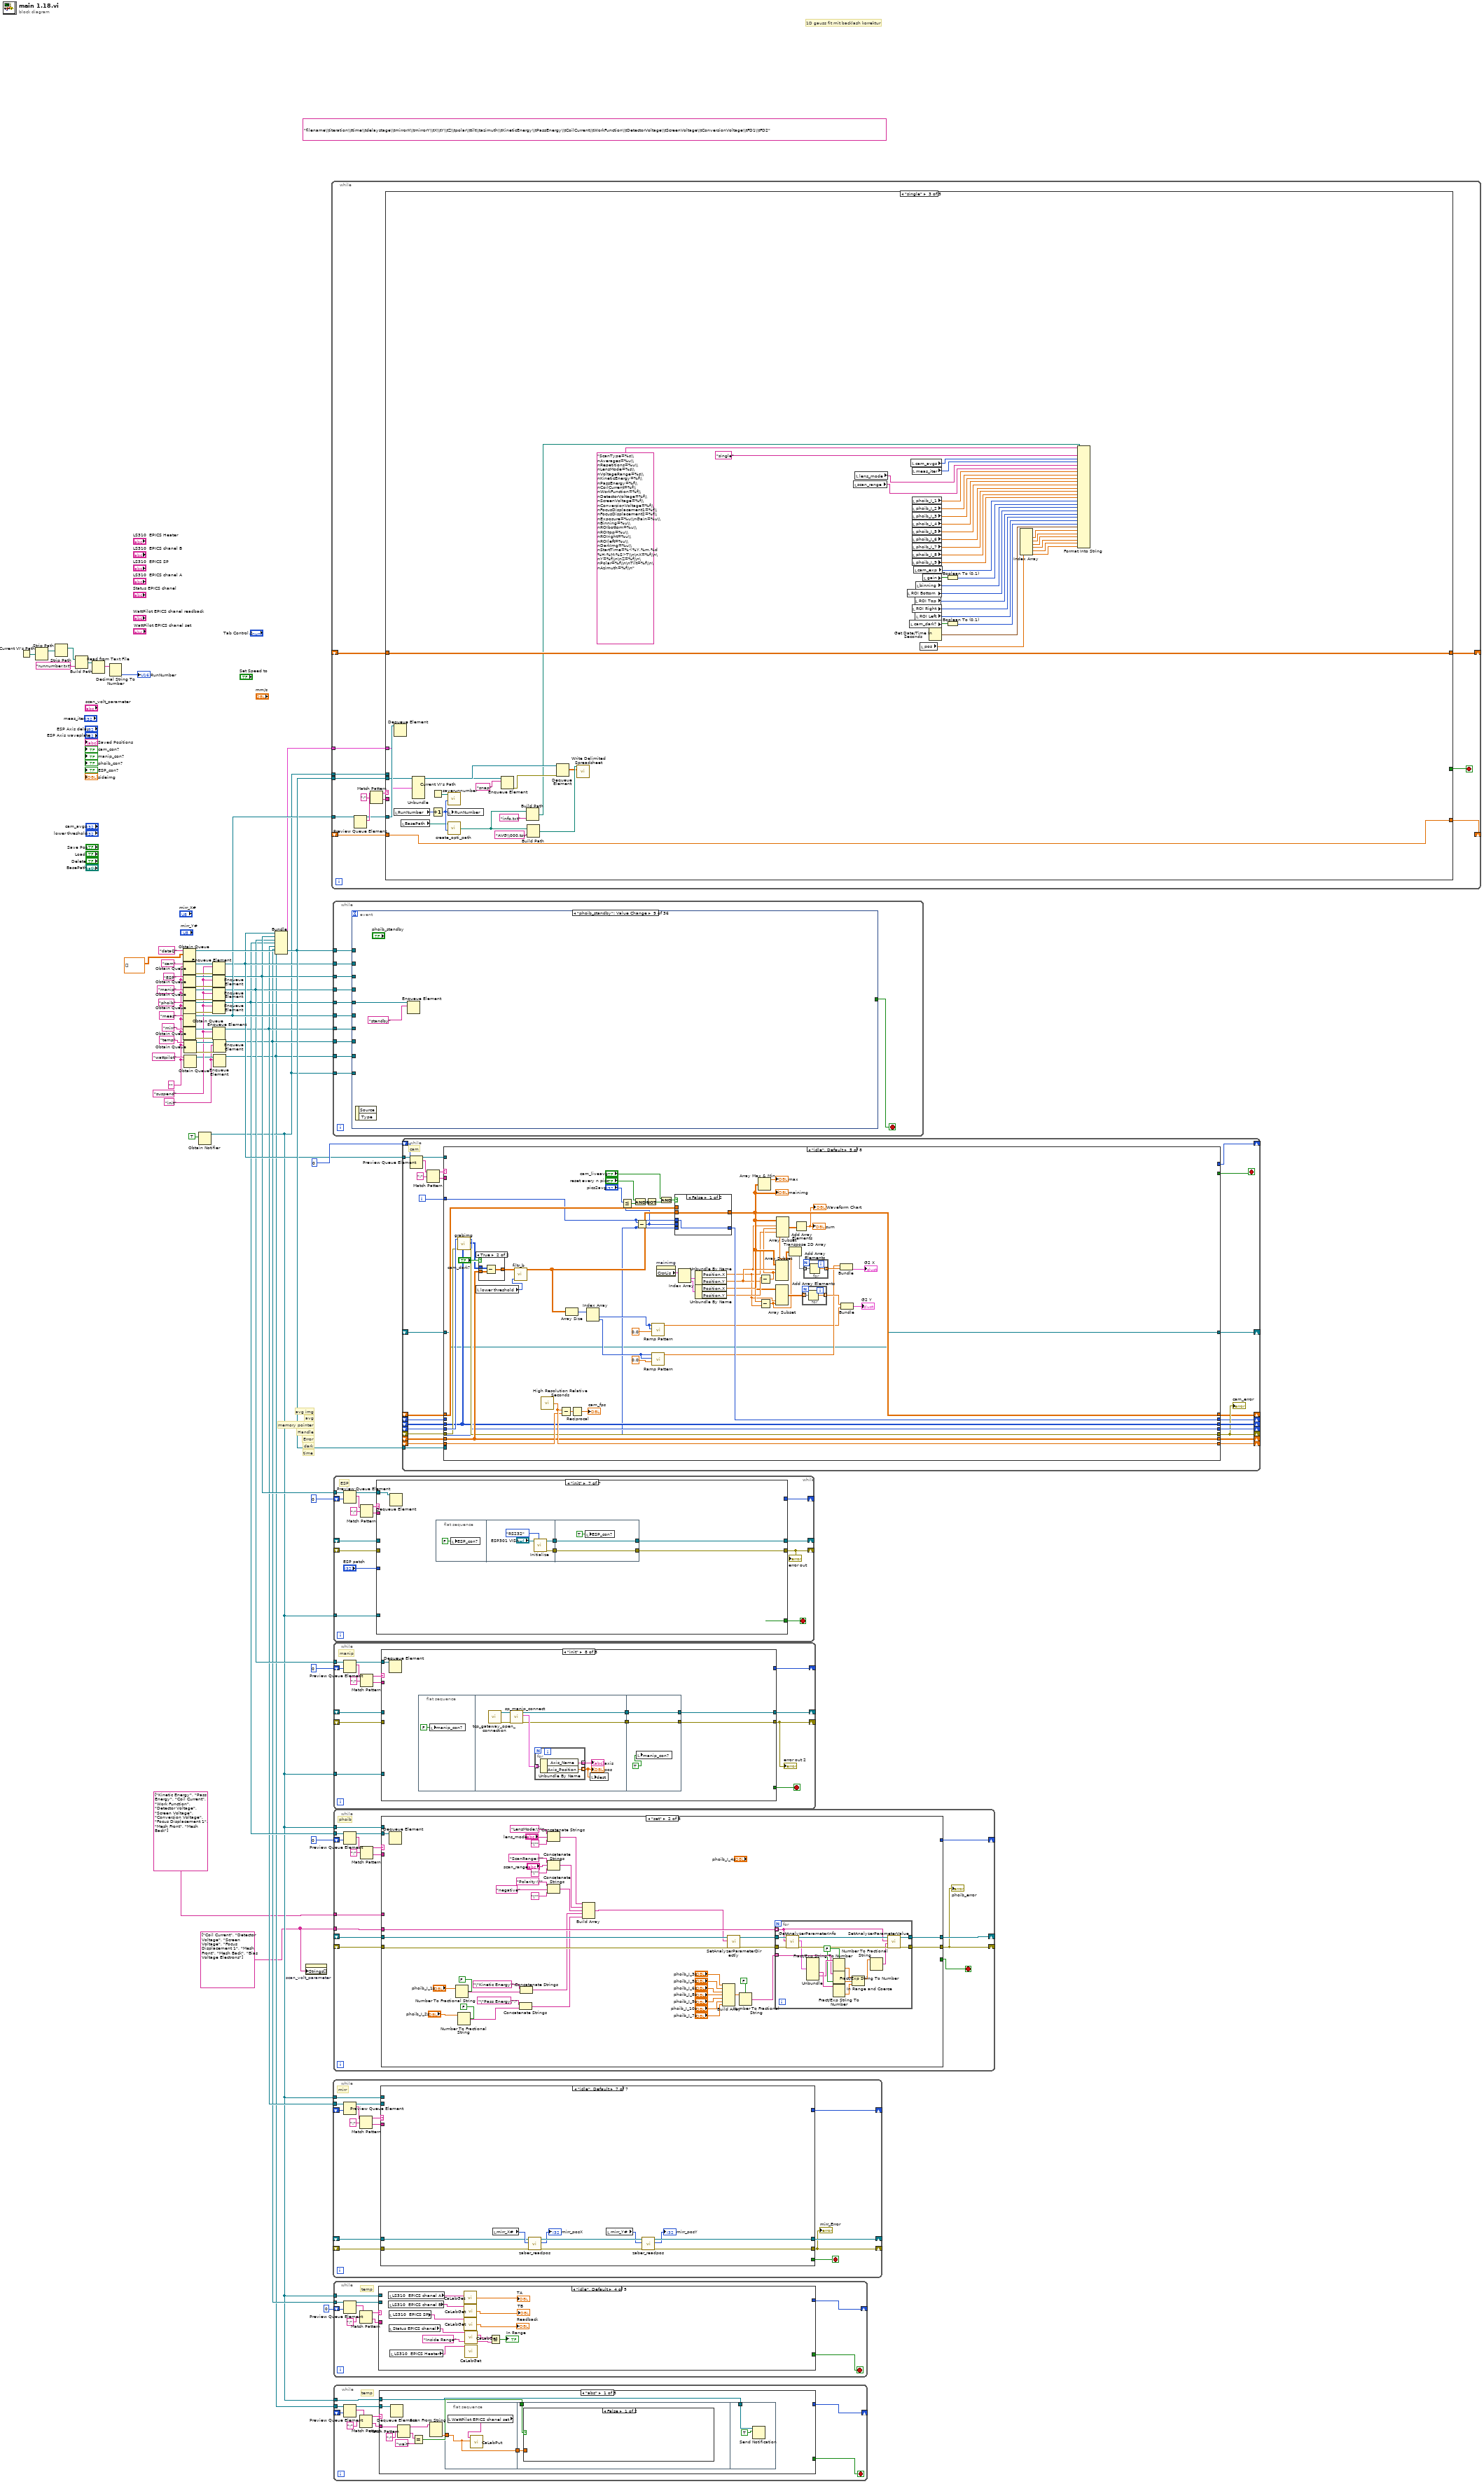
[diagram p0: block diagram]
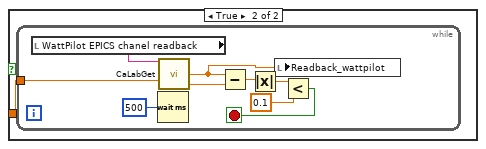
[diagram p2: hidden frame]
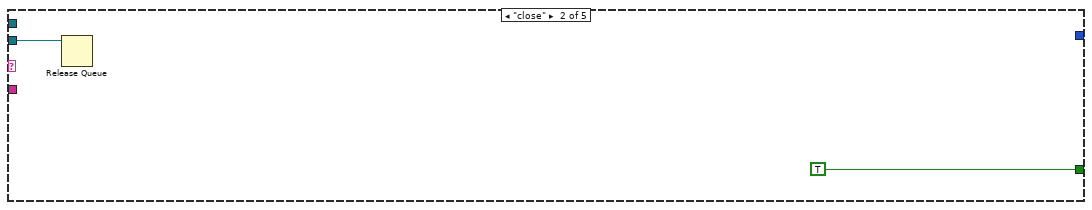
[diagram p3: hidden frame]
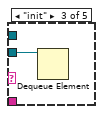
[diagram p4: hidden frame]
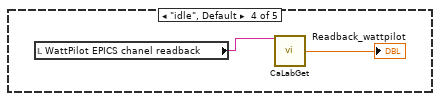
[diagram p5: hidden frame]
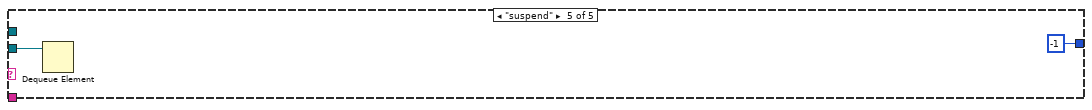
[diagram p6: hidden frame]
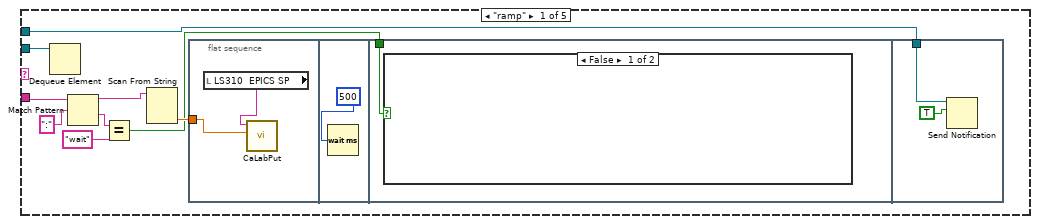
[diagram p7: hidden frame]
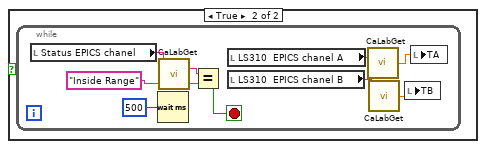
[diagram p8: hidden frame]
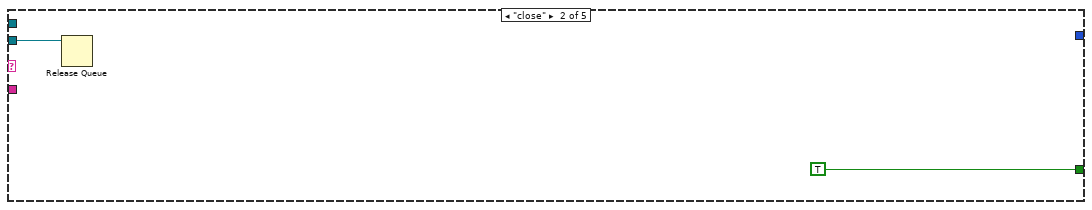
[diagram p9: hidden frame]
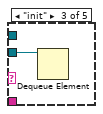
[diagram p10: hidden frame]
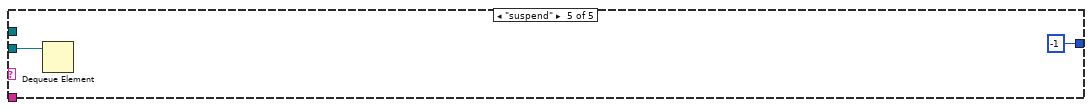
[diagram p11: hidden frame]
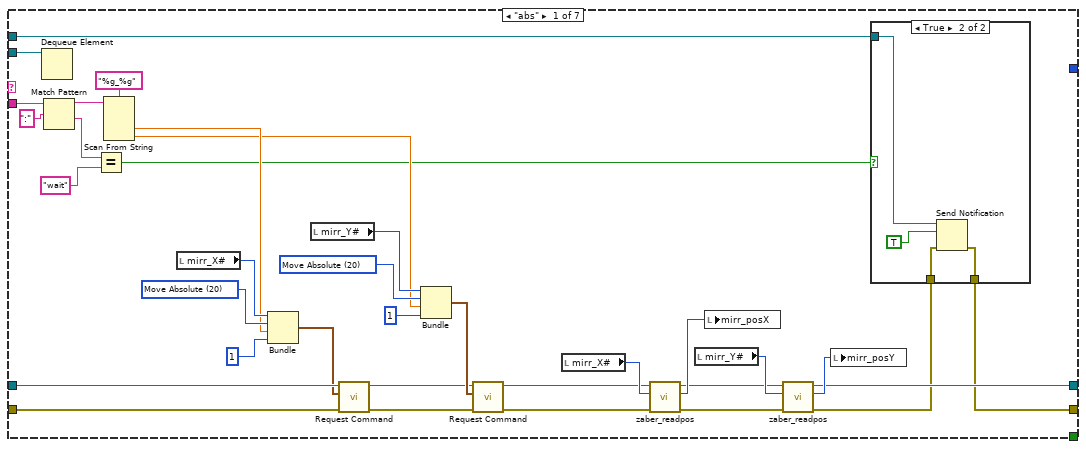
[diagram p12: hidden frame]
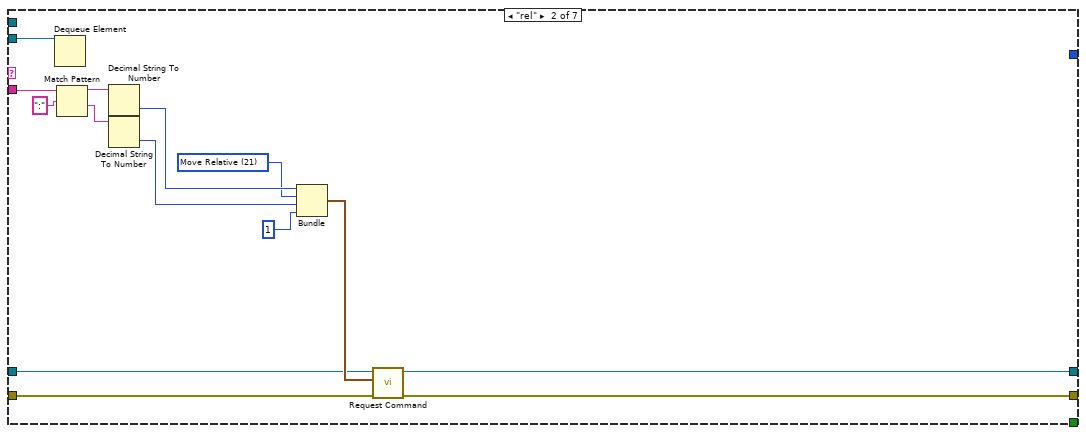
[diagram p14: hidden frame]
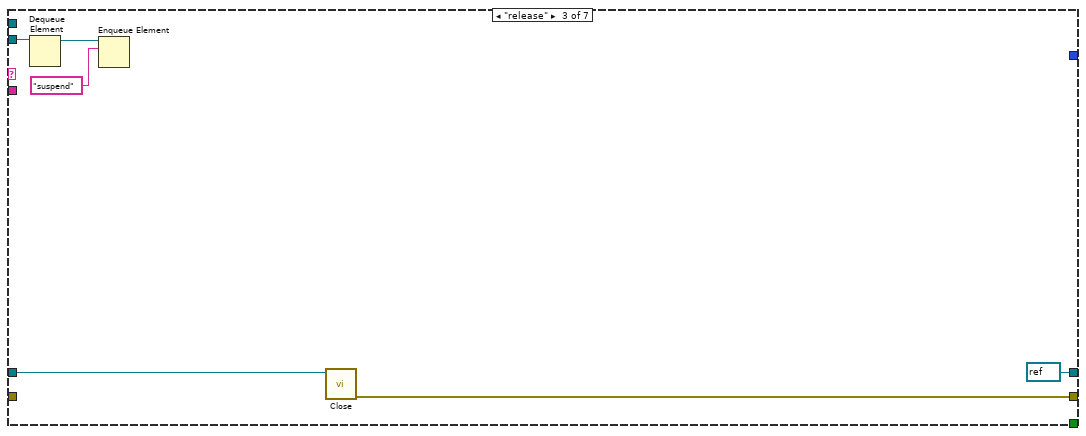
[diagram p15: hidden frame]
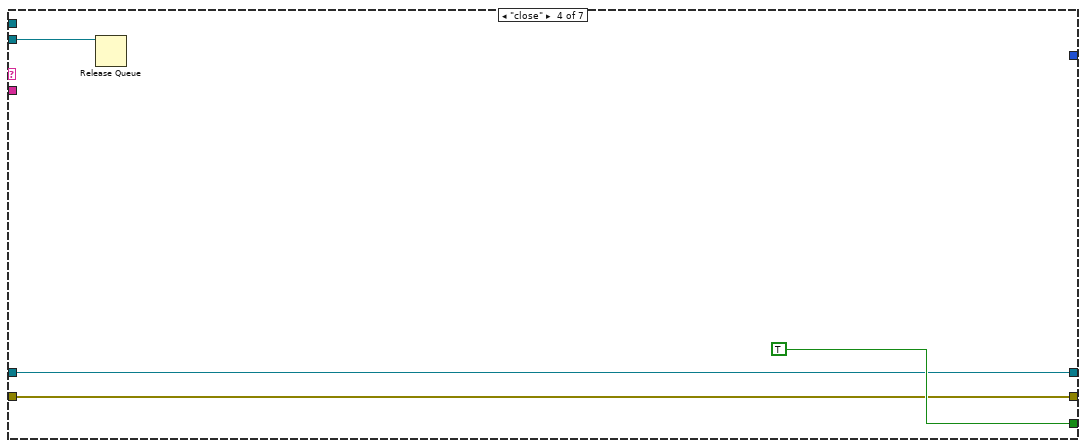
[diagram p16: hidden frame]
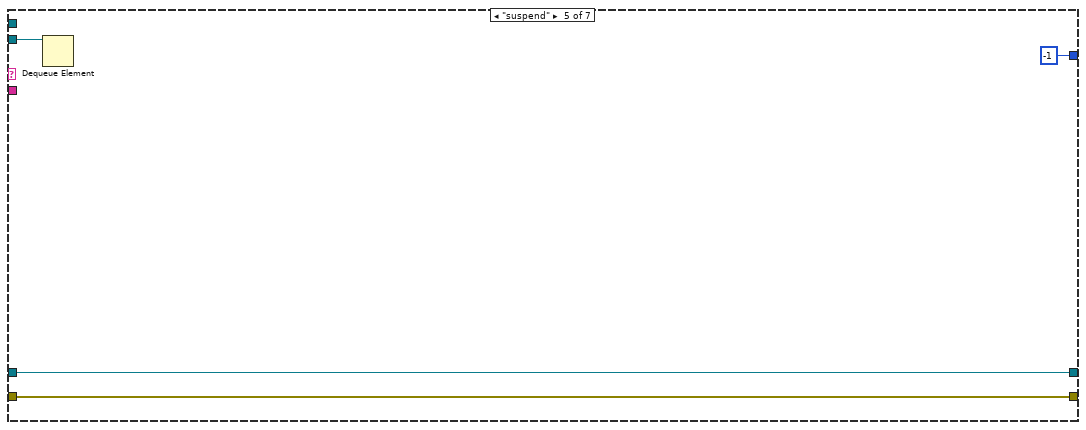
[diagram p17: hidden frame]
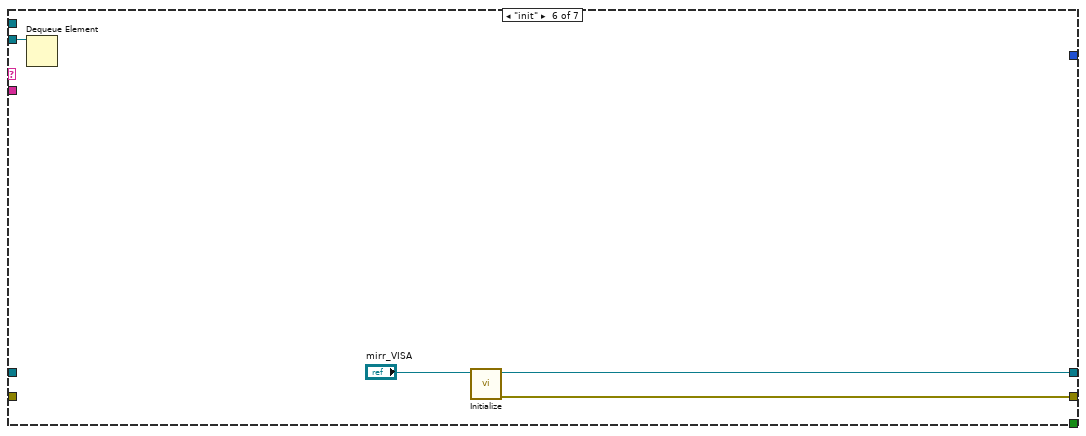
[diagram p18: hidden frame]
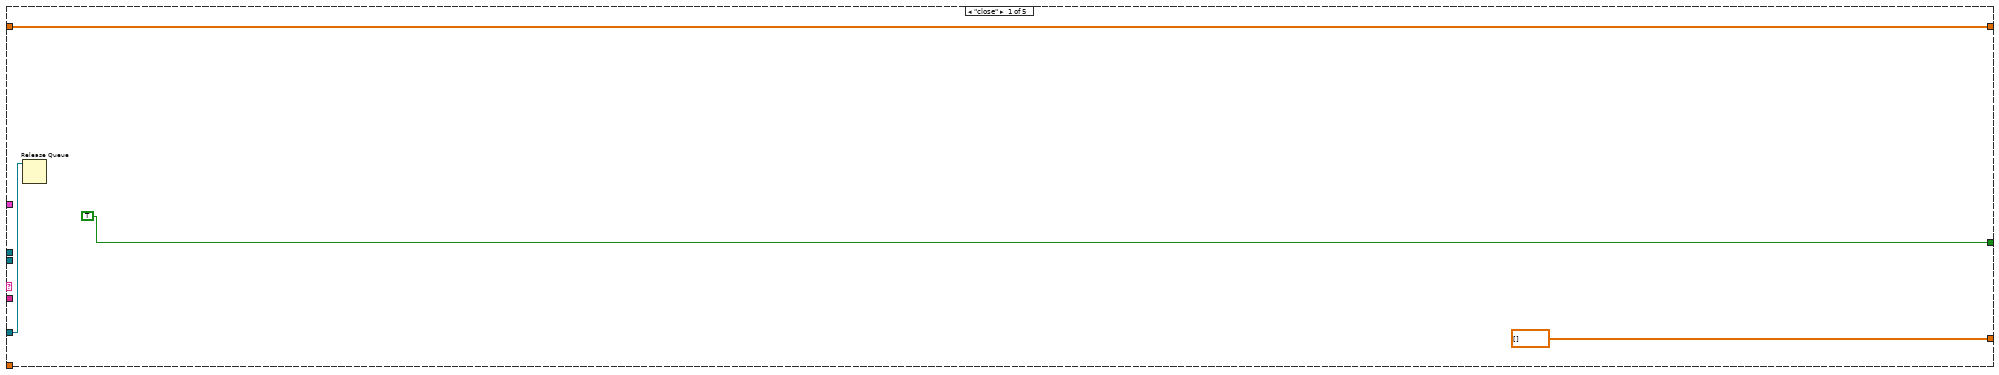
[diagram p19: hidden frame]
diagram:
  w1 = string[] ["Coil Current", "Detector Voltage", "Screen Voltage", "Focus Displacement 1", "Mesh Front", "Mesh Back", "Bias Voltage Electrons"]
  (unwired) "filename\\titeration\\ttime\\tdelaystage\\tmirrorX\\tmirrorY\\tX\\tY\\tZ\\tpolar\\ttilt\\tazimuth\\tKineticEnergy\\tPassEnergy\\tCoilCurrent\\tWorkFunction\\tDetectorVoltage\\tScreenVoltage\\tConversionVoltage\\tFD1\\tFD2"
  w4 = "init" ("name (unnamed)")
  w10 = "suspend" ("name (unnamed)")
  w5 = "" ("name (unnamed)")
  # "1D gauss fit mit backlash korrektur"
  # "avg img"
  # "avg"
  # "time"
  # "dark"
  # "Error"
  # "Handle"
  # "memory pointer"
  n1 = Current VI's Path() -> (path=w27:path)
  n2 = Strip Path(path=w27) -> (stripped path=w31:path)  [unwired: 1 out]
  n3 = Strip Path(path=w31) -> (stripped path=w32:path)  [unwired: 1 out]
  n4 = Build Path(base path=w32, name or relative path="runnumber.txt") -> (appended path=w29:path)
  n5 = Read from Text File(file (use dialog)=w29) -> (text=w30:string)  [unwired: 3 in, 3 out]
  n6 = Decimal String To Number(string=w30) -> (number=→"RunNumber":i32)  [unwired: 2 in, 1 out]
  n7 = Obtain Queue(name (unnamed)="dataQ", element data type=dbl[][] []) -> (queue out=w33:refnum<queue>)  [unwired: 3 in, 2 out]
  n8 = Obtain Queue(name (unnamed)="cam", element data type=w5) -> (queue out=w51:refnum<queue>, error out=w50:errorcluster)  [unwired: 3 in, 1 out]
  n9 = Obtain Queue(name (unnamed)="ESP", element data type=w5) -> (queue out=w48:refnum<queue>, error out=w49:errorcluster)  [unwired: 3 in, 1 out]
  n10 = Obtain Queue(name (unnamed)="manip", element data type=w5) -> (queue out=w45:refnum<queue>, error out=w44:errorcluster)  [unwired: 3 in, 1 out]
  n11 = Obtain Queue(name (unnamed)="phoib", element data type=w5) -> (queue out=w42:refnum<queue>, error out=w43:errorcluster)  [unwired: 3 in, 1 out]
  n12 = Obtain Queue(name (unnamed)="meas", element data type=w5) -> (queue out=w26:refnum<queue>)  [unwired: 3 in, 2 out]
  n13 = Obtain Queue(name (unnamed)="mirr", element data type=w5) -> (queue out=w18:refnum<queue>, error out=w17:errorcluster)  [unwired: 3 in, 1 out]
  n14 = Obtain Queue(name (unnamed)="temp", element data type=w5) -> (queue out=w13:refnum<queue>, error out=w12:errorcluster)  [unwired: 3 in, 1 out]
  n15 = Obtain Queue(name (unnamed)="wattpilot", element data type=w5) -> (queue out=w7:refnum<queue>)  [unwired: 3 in, 2 out]
  n16 = Obtain Notifier(notification data type=TRUE) -> (notifier out=w8:refnum<notifier>)  [unwired: 3 in, 2 out]
  n17 = Enqueue Element(queue=w51, element=w10, error in (no error)=w50) -> (queue out=w24:refnum<queue>)  [unwired: 1 in, 2 out]
  n18 = Enqueue Element(queue=w48, element=w10, error in (no error)=w49) -> (queue out=w23:refnum<queue>)  [unwired: 1 in, 2 out]
  n19 = Enqueue Element(queue=w45, element=w10, error in (no error)=w44) -> (queue out=w22:refnum<queue>)  [unwired: 1 in, 2 out]
  n20 = Enqueue Element(queue=w42, element=w10, error in (no error)=w43) -> (queue out=w21:refnum<queue>)  [unwired: 1 in, 2 out]
  n21 = Enqueue Element(queue=w18, element=w10, error in (no error)=w17) -> (queue out=w15:refnum<queue>)  [unwired: 1 in, 2 out]
  n22 = Enqueue Element(queue=w13, element=w4, error in (no error)=w12) -> (queue out=w9:refnum<queue>)  [unwired: 1 in, 2 out]
  n23 = Enqueue Element(queue=w7, element=w4) -> (queue out=w3:refnum<queue>)  [unwired: 2 in, 2 out]
  n24 = Bundle("queue out"=w24, "queue out"=w23, "queue out"=w22, "queue out"=w21, "queue out"=w15, "queue out"=w9, "queue out"=w3) -> (w25:T2)  [unwired: 1 in]
  n25 = property on="scan_volt_parameter" class="CmbBox"("Strings[]"=w1) -> ()  [unwired: 2 in, 2 out]
  n26 = while {
    tunnel: w33 -> [w66]
    tunnel: w26 -> [w63]
    tunnel: w25 -> [w59]
    shift-right: [w57] -> _
    shift-left: _ -> [w56]
    tunnel: w8 -> [w55]
    shift-right: [w54] -> _
    shift-left: _ -> [w53]
    stop <- w58 stop-if-true
    n27 = Preview Queue Element(queue=w63) -> (queue out=w60:refnum<queue>, element=w65:string)  [unwired: 2 in, 2 out]
    n28 = Match Pattern(string=w65, regular expression=":") -> (before substring=w62:string, after substring=w61:string)  [unwired: 1 in, 2 out]
    n29 = case shown="\"single\"" w62 {
      tunnel: w66 -> [_ _ w122 w146 _]
      tunnel: w61 -> [_ _ _ _ _]
      tunnel: w60 -> [w70 _ w123 w142 w626]
      tunnel: [TRUE _ _ _ _] -> w58
      tunnel: w59 -> [_ _ w110 w139 _]
      tunnel: [w68 w72 w108 w144 w632] -> w57
      tunnel: w56 -> [w68 w72 w108 _ w632]
      tunnel: w55 -> [_ _ _ w143 _]
      tunnel: [dbl[] [] ("Array") w71 w82 w140 w628] -> w54
      tunnel: w53 -> [_ w71 w82 _ w628]
      frame "close" {
        n30 = Release Queue(queue=w70) -> ()  [unwired: 2 in, 3 out]
      }
      frame "idle", Default {
      }
      frame "single" {
        n31 = Dequeue Element(queue=w123) -> ()  [unwired: 2 in, 4 out]
        n32 = local read "RunNumber"() -> (w117:u16)
        n33 = local read "BasePath"() -> (w118:path)
        n34 = Unbundle(w110) -> ("queue out"=w109:refnum<queue>)  [unwired: 6 out]
        n35 = Increment(x=w117) -> (x+1=w119:u16)
        n36 = Current VI's Path() -> (path=w116:path)
        n37 = call "saverunnumber.vi"("RunNumber"=w119, "VI path"=w116) -> ()  [unwired: 10 in]
        n38 = local write "RunNumber"(w119) -> ()
        n39 = call "create_opti_path.vi"("RunNumber"=w119, "base path"=w118) -> ("Path"=w112:path)  [unwired: 2 in]
        n40 = Enqueue Element(queue=w109, element="snap" ("string")) -> (error out=w120:errorcluster)  [unwired: 2 in, 2 out]
        n41 = Build Path(base path=w112, name or relative path="info.txt") -> (appended path=w83:path)
        n42 = Build Path(base path=w112, name or relative path="AVG\\000.tsv") -> (appended path=w114:path)
        n43 = Dequeue Element(queue=w122, error in (no error)=w120) -> (element=w111:dbl[][])  [unwired: 1 in, 3 out]
        n44 = call-poly <vilib>:"Write Delimited Spreadsheet.vi"("file path (dialog if empty)"=w114, "2D data"=w111) -> ()  [unwired: 12 in, 2 out]
        n45 = local read "scan_range"() -> (w73:string)
        n46 = local read "lens_mode"() -> (w74:string)
        n47 = local read "ROI Bottom"() -> (w90:i32)
        n48 = local read "cam_dark?"() -> (w86:bool)
        n49 = local read "cam_avgs"() -> (w105:i32)
        n50 = local read "meas_iter"() -> (w104:i32)
        n51 = local read "phoib_I_1"() -> (w103:dbl)
        n52 = local read "phoib_I_2"() -> (w102:dbl)
        n53 = local read "phoib_I_3"() -> (w101:dbl)
        n54 = local read "phoib_I_4"() -> (w100:dbl)
        n55 = local read "phoib_I_5"() -> (w99:dbl)
        n56 = local read "phoib_I_6"() -> (w98:dbl)
        n57 = local read "phoib_I_7"() -> (w97:dbl)
        n58 = local read "phoib_I_8"() -> (w96:dbl)
        n59 = local read "phoib_I_9"() -> (w95:dbl)
        n60 = local read "ROI Right"() -> (w88:i32)
        n61 = local read "cam_exp"() -> (w94:u32)
        n62 = local read "ROI Top"() -> (w89:i32)
        n63 = local read "ROI Left"() -> (w87:i32)
        n64 = local read "binning"() -> (w91:u16)
        n65 = local read "pos"() -> (w81:dbl[])
        n66 = local read "gain"() -> (w93:bool)
        n67 = Get Date/Time In Seconds() -> (seconds since 1Jan1904=w84:timestamp)
        n68 = Boolean To (0,1)(Boolean=w93) -> (0, 1=w92:i16)
        n69 = Boolean To (0,1)(Boolean=w86) -> (0, 1=w85:i16)
        n70 = Index Array(array=w81) -> (element #1=w80:dbl, element #2=w79:dbl, element #3=w78:dbl, element #4=w77:dbl, element #5=w76:dbl, element #6=w75:dbl)  [unwired: 6 in]
        n71 = Format Into String(format string="ScanType=%s\\nAverages=%u\\nRepetitions=%u\\nLensMode=%s\\nVoltageRange=%s\\nKineticEnergy=%f\\nPassEnergy=%f\\nCoilCurrent=%f\\nWorkFunction=%f\\nDetectorVoltage=%f\\nScreenVoltage=%f\\nConversionVoltage=%f\\nFocusDisplacement1=%f\\nFocusDisplacement2=%f\\nExposure=%u\\nGain=%u\\nBinning=%u\\nROIbottom=%u\\nROItop=%u\\nROIright=%u\\nROIleft=%u\\nDarkImg=%u\\nStartTime=%<%Y.%m.%d %H:%M:%S>T\\n\nX=%f\\n\nY=%f\\n\nZ=%f\\n\nPolar=%f\\n\nTilt=%f\\n\nAzimuth=%f\\n", initial string=w83, "single" ("input 1"), w105, w104, w74, w73, w103, w102, w101, w100, w99, w98, w97, w96, w95, w94, w92, w91, w90, w89, w88, w87, w85, w84, w80, w79, w78, w77, w76, w75) -> ()  [unwired: 1 in, 2 out]
      }
      frame "scan" {
        n72 = Dequeue Element(queue=w142) -> ()  [unwired: 2 in, 4 out]
        n73 = Unbundle(w139) -> ("queue out"=w138:refnum<queue>, "queue out"=w137:refnum<queue>, "queue out"=w136:refnum<queue>, "queue out"=w135:refnum<queue>, "queue out"=w134:refnum<queue>, "queue out"=w124:refnum<queue>)  [unwired: 1 out]
        n74 = call "create scan vectr.vi"("Table Control"="waypointsD2") -> ("Array"=w132:dbl[])
        n75 = for {
          tunnel: "scan_selector 2" -> [w156]
          tunnel: w138 -> [w155]
          tunnel: w137 -> [w154]
          tunnel: w136 -> [w153]
          tunnel: w135 -> [w152]
          tunnel: w134 -> [w151]
          tunnel: [w150] -> w129 mode=indexing
          tunnel: [w149] -> w133
          tunnel: w132 -> [w148] mode=indexing
          tunnel: w124 -> [w147]
          n76 = case shown="\"voltage\"" w156 {
            tunnel: ["" w160 w171 w182 w188 w199 w217 w231 w243] -> w150
            tunnel: w155 -> [w157 w159 w173 _ w187 _ _ _ _]
            tunnel: w154 -> [_ _ _ _ _ w198 _ _ _]
            tunnel: w153 -> [_ _ _ _ _ _ _ _ w242]
            tunnel: w152 -> [_ _ _ _ _ _ w216 _ _]
            tunnel: w151 -> [_ _ _ _ _ _ _ w230 _]
            tunnel: [w157 w159 w173 w181 w187 w198 w216 w230 w242] -> w149
            tunnel: w148 -> [_ w161 w172 w183 w189 w200 w215 w233 w244]
            tunnel: w147 -> [_ _ _ w181 _ _ _ _ _]
            frame "none", Default {
            }
            frame "delay" {
              w164 = ":" ("string")
              n77 = local read "ESP_t0"() -> (w168:dbl)
              n78 = call "time2mm.vi"("fs[1]/ps[0]"=TRUE, "Offset (mm)"=w168, "time"=w161) -> ("position (mm)"=w169:dbl)
              n79 = Number To Decimal String(number=0) -> (decimal integer string=w166:string)  [unwired: 1 in]
              n80 = Number To Fractional String(number=w169) -> (F-format string=w162:string)  [unwired: 3 in]
              n81 = Concatenate Strings("abs:" ("string"), w166, w164, w162, w164, "wait" ("string")) -> (w160:string)
            }
            frame "waveplate" {
              w179 = ":" ("string")
              n82 = Number To Fractional String(number=w172) -> (F-format string=w174:string)  [unwired: 3 in]
              n83 = Number To Decimal String(number=1) -> (decimal integer string=w177:string)  [unwired: 1 in]
              n84 = Concatenate Strings("abs:" ("string"), w177, w179, w174, w179, "wait" ("string")) -> (w171:string)
            }
            frame "wattpilot" {
              n85 = Number To Fractional String(number=w183) -> (F-format string=w184:string)  [unwired: 3 in]
              n86 = Concatenate Strings("abs:" ("string"), w184, ":" ("string"), "wait" ("string")) -> (w182:string)
            }
            frame "stage2" {
              w194 = ":" ("string")
              n87 = Number To Decimal String(number=2) -> (decimal integer string=w191:string)  [unwired: 1 in]
              n88 = Number To Fractional String(number=w189) -> (F-format string=w190:string)  [unwired: 3 in]
              n89 = Concatenate Strings("abs:" ("string"), w191, w194, w190, w194, "wait" ("string")) -> (w188:string)
            }
            frame "manipulator" {
              n90 = call-poly <vilib>:"Vector Norm.vi"("Input Vector"="scan_manip_deltas 2") -> ("norm"=w201:dbl)  [unwired: 9 in, 1 out]
              n91 = Divide(x="scan_manip_deltas 2", y=w201) -> (x/y=w202:dbl[])
              n92 = Multiply(x=w202, y=w200) -> (x*y=w213:dbl[])
              n93 = Add(x="scan_manip_start 2", y=w213) -> (x+y=w214:dbl[])
              n94 = Index Array(array=w214) -> (element #1=w211:dbl, element #2=w210:dbl, element #3=w209:dbl, element #4=w208:dbl, element #5=w207:dbl, element #6=w206:dbl)  [unwired: 6 in]
              n95 = Format Into String(format string="%g_%g_%g_%g_%g_%g", w211, w210, w209, w208, w207, w206) -> (resulting string=w204:string)  [unwired: 2 in, 1 out]
              n96 = Concatenate Strings("abs:" ("string"), w204, ":wait" ("string")) -> (w199:string)
            }
            frame "mirror" {
              n97 = call-poly <vilib>:"Vector Norm.vi"("Input Vector"="scan_mirr_deltas 2") -> ("norm"=w220:dbl)  [unwired: 9 in, 1 out]
              n98 = Divide(x="scan_mirr_deltas 2", y=w220) -> (x/y=w221:dbl[])
              n99 = Multiply(x=w221, y=w215) -> (x*y=w228:dbl[])
              n100 = Add(x="scan_mirr_start 2", y=w228) -> (x+y=w229:dbl[])
              n101 = Index Array(array=w229) -> (element #1=w225:dbl, element #2=w224:dbl)  [unwired: 2 in]
              n102 = Format Into String(format string="%g_%g", w225, w224) -> (resulting string=w222:string)  [unwired: 2 in, 1 out]
              n103 = Concatenate Strings("abs:" ("string"), w222, ":wait" ("string")) -> (w217:string)
            }
            frame "temperature" {
              n104 = Number To Fractional String(number=w233) -> (F-format string=w235:string)  [unwired: 3 in]
              n105 = Concatenate Strings("ramp:" ("string"), w235) -> (w236:string)
              n106 = case shown="True" "Wait for T 2" {
                tunnel: w236 -> [w238 w241]
                tunnel: ":wait" ("string") -> [_ w240]
                tunnel: [w238 w239] -> w231
                frame False {
                }
                frame True {
                  n107 = Concatenate Strings(w241, w240) -> (w239:string)
                }
              }
            }
            frame "voltage" {
              n108 = Number To Fractional String(number=w244) -> (F-format string=w248:string)  [unwired: 3 in]
              n109 = Concatenate Strings("setsgl:" ("string"), "scan_volt_parameter 2", ":" ("string"), w248) -> (w243:string)
            }
          }
        }
        n110 = Array Size(array=w129) -> (size(s)=w126:i32)
        n111 = Equal To 0?(x=w126) -> (x = 0?=w128:bool)
        n112 = Select(t=1, s=w128, f=w126) -> (s? t:f=w125:i32)
        n113 = Get Date/Time In Seconds() -> (seconds since 1Jan1904=w141:timestamp)
        n114 = for {
          N: w125 -> [w250]
          tunnel: w146 -> [w292]
          tunnel: dbl[][][] [] -> [w291]
          tunnel: [w290] -> w144
          tunnel: w143 -> [w287]
          tunnel: w141 -> [w289]
          tunnel: [w288] -> w140
          tunnel: w139 -> [w279]
          tunnel: w129 -> [w254]
          tunnel: w133 -> [w260]
          i -> [w252]
          # "i"
          # "n"
          n115 = local read "RunNumber"() -> (w272:u16)
          n116 = Index Array(array=w254, index=w252) -> (element=w253:string)
          n117 = Increment(x=w252) -> (x+1=w249:i32)
          "current scan 2" <- w249
          n118 = Not Equal?(x="", y=w253) -> (x != y?=w285:bool)
          n119 = local read "BasePath"() -> (w271:path)
          n120 = Divide(x=w249, y=w250) -> (x/y=→"scan 1":dbl)
          n121 = case shown="True" w285 {
            tunnel: w260 -> [_ w475]
            tunnel: w253 -> [_ w474]
            tunnel: w287 -> [_ w473]
            tunnel: [errorcluster {"status"=FALSE, "code"=0, "source"=""} ("error out") w470] -> w259
            frame False {
            }
            frame True {
              n122 = Cancel Notification(0:w473) -> (11:w472:errorcluster)  [unwired: 1 in, 2 out]
              n123 = Enqueue Element(queue=w475, element=w474, error in (no error)=w472) -> (error out=w471:errorcluster)  [unwired: 1 in, 2 out]
              n124 = Wait on Notification(notifier=w473, error in (no error)=w471) -> (error out=w470:errorcluster)  [unwired: 2 in, 3 out]
            }
          }
          n125 = Current VI's Path() -> (path=w273:path)
          n126 = Increment(x=w272) -> (x+1=w270:u16)
          n127 = call "create scan vectr.vi"("Table Control"="waypointsD1") -> ("Array"=w261:dbl[])
          n128 = flat-sequence {
            tunnel: w275 -> [w307]
            tunnel: w262 -> [w301]
            tunnel: w259 -> [w295]
            tunnel: [w295] -> w258
            frame #0 {
              n129 = local read "scan_range"() -> (w293:string)
              n130 = local read "waveplate position"() -> (w298:dbl)
              n131 = local read "lens_mode"() -> (w294:string)
              n132 = local read "stage2 position"() -> (w297:dbl)
              n133 = local read "ESP_pos"() -> (w299:dbl)
              n134 = local read "TA"() -> (w300:dbl)
              n135 = local read "TB"() -> (w296:dbl)
              n136 = local read "ROI Bottom"() -> (w311:i32)
              n137 = local read "cam_dark?"() -> (w306:bool)
              n138 = local read "cam_avgs"() -> (w303:i32)
              n139 = local read "meas_iter"() -> (w304:i32)
              n140 = local read "ROI Right"() -> (w313:i32)
              n141 = local read "phoib_I_1"() -> (w316:dbl)
              n142 = local read "phoib_I_2"() -> (w317:dbl)
              n143 = local read "phoib_I_3"() -> (w318:dbl)
              n144 = local read "phoib_I_4"() -> (w319:dbl)
              n145 = local read "phoib_I_5"() -> (w320:dbl)
              n146 = local read "phoib_I_6"() -> (w321:dbl)
              n147 = local read "phoib_I_7"() -> (w322:dbl)
              n148 = local read "phoib_I_8"() -> (w323:dbl)
              n149 = local read "phoib_I_9"() -> (w324:dbl)
              n150 = local read "cam_exp"() -> (w308:u32)
              n151 = local read "ROI Top"() -> (w312:i32)
              n152 = local read "ROI Left"() -> (w314:i32)
              n153 = local read "binning"() -> (w310:u16)
              n154 = local read "ESP_t0"() -> (w325:dbl)
              n155 = local read "gain"() -> (w305:bool)
              n156 = Boolean To (0,1)(Boolean=w305) -> (0, 1=w309:i16)
              n157 = Boolean To (0,1)(Boolean=w306) -> (0, 1=w315:i16)
              n158 = Format Into String(format string="ScanType:%s\\nAverages:%u\\nRepetitions:%u\\nLensMode:%s\\nVoltageRange:%s\\nExposure:%u\\nGain:%u\\nBinning:%u\\nROIbottom:%u\\nROItop:%u\\nROIright:%u\\nROIleft:%u\\nDarkImg:%u\\nKineticEnergy:%f\\nPassEnergy:%f\\nCoilCurrent:%f\\nWorkFunction:%f\\nDetectorVoltage:%f\\nScreenVoltage:%f\\nConversionVoltage:%f\\nFocusDisplacement1:%f\\nFocusDisplacement2:%f\\nTimeZero:%f\\nDelayStage:%f\\nWaveplate:%f\\n2ndStage:%f\\nTempA:%f\\nTempB:%f\\n", initial string=w301, w307, w303, w304, w294, w293, w308, w309, w310, w311, w312, w313, w314, w315, w316, w317, w318, w319, w320, w321, w322, w323, w324, w325, w299, w298, w297, w300, w296) -> ()  [unwired: 1 in, 2 out]
            }
          }
          n159 = call "create_opti_path.vi"("RunNumber"=w270, "base path"=w271) -> ("Path"=w263:path)  [unwired: 2 in]
          n160 = call "saverunnumber.vi"("RunNumber"=w270, "VI path"=w273) -> ()  [unwired: 10 in]
          n161 = local write "RunNumber"(w270) -> ()
          n162 = Unbundle(w279) -> ("queue out"=w278:refnum<queue>, "queue out"=w280:refnum<queue>, "queue out"=w281:refnum<queue>, "queue out"=w282:refnum<queue>, "queue out"=w283:refnum<queue>, "queue out"=w284:refnum<queue>, "queue out"=w251:refnum<queue>)
          n163 = Build Path(base path=w263, name or relative path="scanvector.txt") -> (appended path=w265:path)
          n164 = for {
            tunnel: [w345] -> w277 mode=indexing
            tunnel: [w344] -> w276
            tunnel: w280 -> [w343]
            tunnel: w281 -> [w342]
            tunnel: w282 -> [w341]
            tunnel: w283 -> [w340]
            tunnel: w265 -> [w339]
            tunnel: w284 -> [w338]
            tunnel: w261 -> [w337] mode=indexing
            tunnel: "scan_selector" -> [w335]
            tunnel: w251 -> [w333]
            i -> [w334]
            stop <- w336 stop-if-true
            n165 = case shown="\"none\", Default" w335 {
              tunnel: w337 -> [w354 _ w368 w382 w390 w421 w433 w450 w459]
              tunnel: [w352 w362 w365 w379 w391 w409 w430 w448 w463] -> w344
              tunnel: [w357 "" w369 w383 w392 w410 w431 w443 w464] -> w345
              tunnel: w343 -> [w352 w362 w365 _ w391 _ _ _ _]
              tunnel: w342 -> [_ _ _ _ _ w409 _ _ _]
              tunnel: w341 -> [_ _ _ _ _ _ _ _ w463]
              tunnel: w340 -> [_ _ _ _ _ _ w430 _ _]
              tunnel: w339 -> [w347 _ w367 w381 w389 w405 w427 w451 w460]
              tunnel: w338 -> [_ _ _ _ _ _ _ w448 _]
              tunnel: [_ TRUE _ _ _ _ _ _ _] -> w336
              tunnel: w334 -> [_ _ _ _ _ _ _ _ _]
              tunnel: w333 -> [_ _ _ w379 _ _ _ _ _]
              frame "delay" {
                w359 = ":" ("string")
                n166 = local read "ESP_t0"() -> (w353:dbl)
                n167 = call "time2mm.vi"("fs[1]/ps[0]"=TRUE, "Offset (mm)"=w353, "time"=w354) -> ("position (mm)"=w349:dbl)
                n168 = Build Array(w349) -> (w348:dbl[])
                n169 = Number To Decimal String(number=0) -> (decimal integer string=w356:string)  [unwired: 1 in]
                n170 = Number To Fractional String(number=w349) -> (F-format string=w361:string)  [unwired: 3 in]
                n171 = call-poly <vilib>:"Write Delimited Spreadsheet.vi"("file path (dialog if empty)"=w347, "format (%.3f)"="%.6f", "1D data"=w348, "append to file? (new file:F)"=TRUE ("append to file? (F)")) -> ()  [unwired: 10 in, 2 out]
                n172 = Concatenate Strings("abs:" ("string"), w356, w359, w361, w359, "wait" ("string")) -> (w357:string)
              }
              frame "none", Default {
              }
              frame "waveplate" {
                w366 = ":" ("string")
                n173 = Number To Fractional String(number=w368) -> (F-format string=w377:string)  [unwired: 3 in]
                n174 = Build Array(w368) -> (w371:dbl[])
                n175 = Number To Decimal String(number=1) -> (decimal integer string=w374:string)  [unwired: 1 in]
                n176 = call-poly <vilib>:"Write Delimited Spreadsheet.vi"("file path (dialog if empty)"=w367, "format (%.3f)"="%.6f", "1D data"=w371, "append to file? (new file:F)"=TRUE ("append to file? (F)")) -> ()  [unwired: 10 in, 2 out]
                n177 = Concatenate Strings("abs:" ("string"), w374, w366, w377, w366, "wait" ("string")) -> (w369:string)
              }
              frame "wattpilot" {
                n178 = Number To Fractional String(number=w382) -> (F-format string=w388:string)  [unwired: 3 in]
                n179 = Build Array(w382) -> (w384:dbl[])
                n180 = call-poly <vilib>:"Write Delimited Spreadsheet.vi"("file path (dialog if empty)"=w381, "format (%.3f)"="%.6f", "1D data"=w384, "append to file? (new file:F)"=TRUE ("append to file? (F)")) -> ()  [unwired: 10 in, 2 out]
                n181 = Concatenate Strings("abs:" ("string"), w388, ":" ("string"), "wait" ("string")) -> (w383:string)
              }
              frame "stage2" {
                w394 = ":" ("string")
                n182 = Build Array(w390) -> (w399:dbl[])
                n183 = Number To Decimal String(number=2) -> (decimal integer string=w400:string)  [unwired: 1 in]
                n184 = Number To Fractional String(number=w390) -> (F-format string=w401:string)  [unwired: 3 in]
                n185 = call-poly <vilib>:"Write Delimited Spreadsheet.vi"("file path (dialog if empty)"=w389, "format (%.3f)"="%.6f", "1D data"=w399, "append to file? (new file:F)"=TRUE ("append to file? (F)")) -> ()  [unwired: 10 in, 2 out]
                n186 = Concatenate Strings("abs:" ("string"), w400, w394, w401, w394, "wait" ("string")) -> (w392:string)
              }
              frame "manipulator" {
                n187 = call-poly <vilib>:"Vector Norm.vi"("Input Vector"="scan_manip_deltas") -> ("norm"=w423:dbl)  [unwired: 9 in, 1 out]
                n188 = Divide(x="scan_manip_deltas", y=w423) -> (x/y=w422:dbl[])
                n189 = Multiply(x=w422, y=w421) -> (x*y=w408:dbl[])
                n190 = Add(x="scan_manip_start", y=w408) -> (x+y=w404:dbl[])
                n191 = call-poly <vilib>:"Write Delimited Spreadsheet.vi"("file path (dialog if empty)"=w405, "format (%.3f)"="%.6f", "1D data"=w404, "append to file? (new file:F)"=TRUE ("append to file? (F)")) -> ()  [unwired: 10 in, 2 out]
                n192 = Index Array(array=w404) -> (element #1=w412:dbl, element #2=w413:dbl, element #3=w414:dbl, element #4=w415:dbl, element #5=w416:dbl, element #6=w417:dbl)  [unwired: 6 in]
                n193 = Format Into String(format string="%g_%g_%g_%g_%g_%g", w412, w413, w414, w415, w416, w417) -> (resulting string=w419:string)  [unwired: 2 in, 1 out]
                n194 = Concatenate Strings("abs:" ("string"), w419, ":wait" ("string")) -> (w410:string)
              }
              frame "mirror" {
                n195 = call-poly <vilib>:"Vector Norm.vi"("Input Vector"="scan_mirr_deltas") -> ("norm"=w441:dbl)  [unwired: 9 in, 1 out]
                n196 = Divide(x="scan_mirr_deltas", y=w441) -> (x/y=w440:dbl[])
                n197 = Multiply(x=w440, y=w433) -> (x*y=w429:dbl[])
                n198 = Add(x="scan_mirr_start", y=w429) -> (x+y=w426:dbl[])
                n199 = call-poly <vilib>:"Write Delimited Spreadsheet.vi"("file path (dialog if empty)"=w427, "format (%.3f)"="%.6f", "1D data"=w426, "append to file? (new file:F)"=TRUE ("append to file? (F)")) -> ()  [unwired: 10 in, 2 out]
                n200 = Index Array(array=w426) -> (element #1=w436:dbl, element #2=w437:dbl)  [unwired: 2 in]
                n201 = Format Into String(format string="%g_%g", w436, w437) -> (resulting string=w439:string)  [unwired: 2 in, 1 out]
                n202 = Concatenate Strings("abs:" ("string"), w439, ":wait" ("string")) -> (w431:string)
              }
              frame "temperature" {
                n203 = Build Array(w450) -> (w449:dbl[])
                n204 = Number To Fractional String(number=w450) -> (F-format string=w447:string)  [unwired: 3 in]
                n205 = Concatenate Strings("ramp:" ("string"), w447) -> (w445:string)
                n206 = case shown="False" "Wait for T" {
                  tunnel: w445 -> [w454 w457]
                  tunnel: ":wait" ("string") -> [_ w456]
                  tunnel: [w454 w455] -> w443
                  frame False {
                  }
                  frame True {
                    n207 = Concatenate Strings(w457, w456) -> (w455:string)
                  }
                }
                n208 = call-poly <vilib>:"Write Delimited Spreadsheet.vi"("file path (dialog if empty)"=w451, "format (%.3f)"="%.6f", "1D data"=w449, "append to file? (new file:F)"=TRUE ("append to file? (F)")) -> ()  [unwired: 10 in, 2 out]
              }
              frame "voltage" {
                n209 = local read "scan_volt_parameter"() -> (w467:string)
                n210 = Build Array(w459) -> (w458:dbl[])
                n211 = Number To Fractional String(number=w459) -> (F-format string=w465:string)  [unwired: 3 in]
                n212 = Concatenate Strings("setsgl:" ("string"), w467, ":" ("string"), w465) -> (w464:string)
                n213 = call-poly <vilib>:"Write Delimited Spreadsheet.vi"("file path (dialog if empty)"=w460, "format (%.3f)"="%.6f", "1D data"=w458, "append to file? (new file:F)"=TRUE ("append to file? (F)")) -> ()  [unwired: 10 in, 2 out]
              }
            }
          }
          n214 = Build Path(base path=w263, name or relative path="RAW\\LUT.txt") -> (appended path=w274:path)
          n215 = case shown="\"waveplate\"" "scan_selector" {
            tunnel: ["delay" ("input 1") "waveplate" ("input 1") "stage2" ("input 1") "manipulator" ("input 1") "temperature" "mirror" ("input 1") "voltage" ("input 1")] -> w275
            frame "delay", Default {
            }
            frame "waveplate" {
            }
            frame "stage2" {
            }
            frame "manipulator" {
            }
            frame "temperature" {
            }
            frame "mirror" {
            }
            frame "voltage" {
            }
          }
          n216 = Build Path(base path=w263, name or relative path="info.txt") -> (appended path=w262:path)
          n217 = call-poly <vilib>:"Write Delimited Spreadsheet.vi"("file path (dialog if empty)"=w274, "1D data"=string[] ["filename", "time", "delaystage", "X", "Y", "Z", "polar", "tilt", "azimuth", "mirrorX", "mirrorY", "KineticEnergy", "PassEnergy", "CoilCurrent", "WorkFunction", "DetectorVoltage", "ScreenVoltage", "ConversionVoltage", "FD1", "FD2"]) -> ("new file path (Not A Path if cancelled)"=w266:path)  [unwired: 12 in, 1 out]
          n218 = while {
            tunnel: w263 -> [w497]
            tunnel: w292 -> [w496]
            shift-right: [w495] -> w290
            shift-left: w291 -> [w494]
            tunnel: w287 -> [w493]
            tunnel: w289 -> [w492]
            tunnel: w276 -> [w491]
            tunnel: w277 -> [w490]
            tunnel: w278 -> [w489]
            shift-right: [w487] -> _
            shift-left: w266 -> [w488]
            shift-right: [w486] -> w288
            shift-left: w261 -> [w485]
            tunnel: w258 -> [w478]
            tunnel: w250 -> [w477]
            tunnel: w252 -> [w476]
            i -> [w484]
            stop <- w481 stop-if-true
            n219 = local read "meas_iter"() -> (w483:i32)
            n220 = for {
              N -> [w534]
              tunnel: w497 -> [w532]
              tunnel: w496 -> [w553]
              tunnel: w484 -> [w530]
              shift-right: [w544] -> w495
              shift-left: w494 -> [w549]
              tunnel: w493 -> [w546]
              tunnel: w492 -> [w533]
              tunnel: w491 -> [w526]
              tunnel: w490 -> [w506] mode=indexing
              tunnel: w489 -> [w525]
              shift-right: [w521] -> w487
              shift-left: w488 -> [w522]
              shift-right: [w517] -> w486
              shift-left: w485 -> [w517]
              tunnel: [w514] -> w480
              tunnel: w483 -> [w513]
              tunnel: w478 -> [w508]
              tunnel: w477 -> [w500]
              tunnel: w476 -> [w504]
              i -> [w531]
              stop <- "stop after step" stop-if-true
              n221 = Not Equal?(x="", y=w506) -> (x != y?=w505:bool)
              n222 = case shown="True" w505 {
                tunnel: [w558 w564] -> w548
                tunnel: w546 -> [_ w562]
                tunnel: w526 -> [_ w561]
                tunnel: w506 -> [_ w560]
                tunnel: w508 -> [w558 w559]
                frame False {
                }
                frame True {
                  n223 = Cancel Notification(0:w562, 3:w559) -> (11:w563:errorcluster)  [unwired: 2 out]
                  n224 = Enqueue Element(queue=w561, element=w560, error in (no error)=w563) -> (error out=w565:errorcluster)  [unwired: 1 in, 2 out]
                  n225 = Wait on Notification(notifier=w562, error in (no error)=w565) -> (error out=w564:errorcluster)  [unwired: 2 in, 3 out]
                }
              }
              n226 = Equal To 0?(x=w531) -> (x = 0?=w552:bool)
              n227 = Equal To 0?(x=w530) -> (x = 0?=w551:bool)
              n228 = Get Date/Time In Seconds() -> (seconds since 1Jan1904=w523:timestamp)
              n229 = And(x=w552, y=w551) -> (x .and. y?=w550:bool)
              n230 = Enqueue Element(queue=w525, element="snap", error in (no error)=w548) -> (error out=w547:errorcluster)  [unwired: 1 in, 2 out]
              n231 = call "createFileStruc.vi"("i_iter"=w530, "i_delay"=w531, "meas_path"=w532) -> ("AVG file"=w527:path, "RAW file"=w519:path)  [unwired: 7 in]
              n232 = Dequeue Element(queue=w553, error in (no error)=w547) -> (element=w529:dbl[][], error out=w520:errorcluster)  [unwired: 1 in, 2 out]
              n233 = Strip Path(path=w519) -> (name=w518:string)  [unwired: 1 out]
              n234 = Array Size(array=w529) -> (size(s)=w557:i32[])
              n235 = call-poly <vilib>:"Write Delimited Spreadsheet.vi"("file path (dialog if empty)"=w519, "2D data"=w529, "error in (no error)"=w520) -> ()  [unwired: 11 in, 2 out]
              n236 = Index Array(array=w557) -> (element #1=w555:i32, element #2=w554:i32)  [unwired: 2 in]
              n237 = Subtract(x=w523, y=w533) -> (x-y=w536:dbl)
              n238 = flat-sequence {
                tunnel: "%s\\t%<%Y.%m.%d %H:%M:%S>T\\t%f\\t%f\\t%f\\t%f\\t%f\\t%f\\t%f\\t%f\\t%f\\t%f\\t%f\\t%f\\t%f\\t%f\\t%f\\t%f\\t%f\\t%f\\t%f" -> [w595]
                tunnel: w523 -> [w594]
                tunnel: w522 -> [w571]
                tunnel: [w570] -> w521
                tunnel: w520 -> [w567]
                tunnel: w518 -> [w566]
                frame #0 {
                  n239 = local read "pos"() -> (w596:dbl[])
                  n240 = local read "mirr_posX"() -> (w583:i32)
                  n241 = local read "mirr_posY"() -> (w584:i32)
                  n242 = local read "ESP_delay"() -> (w576:dbl)
                  n243 = local read "phoib_I_1"() -> (w585:dbl)
                  n244 = local read "phoib_I_2"() -> (w586:dbl)
                  n245 = local read "phoib_I_3"() -> (w587:dbl)
                  n246 = local read "phoib_I_4"() -> (w588:dbl)
                  n247 = local read "phoib_I_5"() -> (w589:dbl)
                  n248 = local read "phoib_I_6"() -> (w590:dbl)
                  n249 = local read "phoib_I_7"() -> (w591:dbl)
                  n250 = local read "phoib_I_8"() -> (w592:dbl)
                  n251 = local read "phoib_I_9"() -> (w593:dbl)
                  n252 = local read "ESP_pos"() -> (w575:dbl)
                  n253 = Index Array(array=w596) -> (element #1=w577:dbl, element #2=w578:dbl, element #3=w579:dbl, element #4=w580:dbl, element #5=w581:dbl, element #6=w582:dbl)  [unwired: 6 in]
                  n254 = Format Into String(format string=w595, error in=w567, w566, w594, w575, w576, w577, w578, w579, w580, w581, w582, w583, w584, w585, w586, w587, w588, w589, w590, w591, w592, w593) -> (resulting string=w573:string)  [unwired: 1 in, 1 out]
                  n255 = Spreadsheet String To Array(format string="%s", spreadsheet string=w573, array type (2D Dbl)=string[] []) -> (array=w569:string[])  [unwired: 1 in]
                  n256 = call-poly <vilib>:"Write Delimited Spreadsheet.vi"("file path (dialog if empty)"=w571, "1D data"=w569, "append to file? (new file:F)"=TRUE ("append to file? (F)")) -> ("new file path (Not A Path if cancelled)"=w570:path)  [unwired: 11 in, 1 out]
                }
              }
              n257 = case shown="True" w550 {
                tunnel: w534 -> [_ w602]
                tunnel: [w597 w600] -> w556
                tunnel: w549 -> [w597 _]
                tunnel: w555 -> [_ w599]
                tunnel: w554 -> [_ w598]
                frame False {
                }
                frame True {
                  n258 = Initialize Array(0.0 ("element"), w602, w599, w598) -> (w600:dbl[][][])
                }
              }
              n259 = Increment(x=w531) -> (x+1=w540:i32)
              "current scan" <- w540
              n260 = Increment(x=w530) -> (x+1=w539:i32)
              "current iteration" <- w539
              n261 = for {
                N: w555 -> [_]
                tunnel: w531 -> [w609]
                shift-right: [w607] -> w544
                shift-left: w556 -> [w610]
                tunnel: w530 -> [w605]
                shift-right: [w604] -> w528
                shift-left: w529 -> [w606]
                tunnel: w554 -> [w603]
                i -> [w608]
                n262 = for {
                  N: w603 -> [_]
                  tunnel: w609 -> [w617]
                  tunnel: w608 -> [w614]
                  shift-right: [w616] -> w607
                  shift-left: w610 -> [w618]
                  tunnel: w605 -> [w612]
                  shift-right: [w611] -> w604
                  shift-left: w606 -> [w615]
                  i -> [w613]
                  n263 = in-place {
                    in-place-border: w612 -> [w624]
                    n264 = in-place-array #1(w618, w617, w614, w613) -> (w625:dbl)
                    n265 = in-place-array #2(w615, w614, w613) -> (w622:dbl)
                    n266 = Multiply(x=w625, y=w624) -> (x*y=w623:dbl)
                    n267 = Increment(x=w624) -> (x+1=w620:i32)
                    n268 = Add(x=w623, y=w622) -> (x+y=w621:dbl)
                    n269 = Divide(x=w621, y=w620) -> (x/y=w619:dbl)
                    n270 = in-place-array #1(w619) -> (w616:dbl[][][])  [unwired: 3 out]
                    n271 = in-place-array #2(w619) -> (w611:dbl[][])  [unwired: 2 out]
                  }
                }
              }
              n272 = Multiply(x=w534, y=w530) -> (x*y=w535:i32)
              n273 = Multiply(x=w534, y=w513) -> (x*y=w499:i32)
              n274 = Divide(x=w540, y=w534) -> (x/y=→"scan 2":dbl)
              n275 = Divide(x=w539, y=w513) -> (x/y=→"iteration":dbl)
              n276 = Add(x=w531, y=w535) -> (x+y=w502:i32)
              n277 = Multiply(x=w504, y=w499) -> (x*y=w503:i32)
              n278 = Add(x=w502, y=w503) -> (x+y=w501:i32)
              n279 = Divide(x=w536, y=w501) -> (x/y=w509:dbl)
              n280 = Multiply(x=w500, y=w499) -> (x*y=w498:i32)
              n281 = Multiply(x=w509, y=w498) -> (x*y=w512:dbl)
              n282 = local write "duration [HH:MM:SS]"(w512) -> ()
              n283 = local write "time/step [s]"(w509) -> ()
              n284 = property on="mainimg" class="IntGraph (strict)"() -> ("CrsrLis"=w543:T3)  [unwired: 2 in, 2 out]
              n285 = call-poly <vilib>:"Write Delimited Spreadsheet.vi"("file path (dialog if empty)"=w527, "2D data"=w528) -> ()  [unwired: 12 in, 2 out]
              n286 = call "processData.vi"("Cursor List"=w543, "data in"=w544) -> ("Angle Chart"=→"anglegraph":dbl[][], "Energy Chart"=→"energygraph":dbl[][], "Intensity Chart"=w542:dbl[])  [unwired: 1 in]
              n287 = Bundle("Array"=w517, "Intensity Chart"=w542) -> (→"intensitygraph":cluster{"Array":dbl[], "Intensity Chart":dbl[]})  [unwired: 1 in]
              n288 = Or(x="stop after iteration", y="stop after step") -> (x .or. y?=w514:bool)
            }
            n289 = Increment(x=w484) -> (x+1=w482:i32)
            n290 = Greater Or Equal?(x=w482, y=w483) -> (x >= y?=w479:bool)
            n291 = Or(x=w480, y=w479) -> (x .or. y?=w481:bool)
          }
        }
      }
      frame "refresh" {
        n292 = Dequeue Element(queue=w626) -> ()  [unwired: 2 in, 4 out]
        n293 = property on="mainimg" class="IntGraph (strict)"() -> ("CrsrLis"=w633:T3)  [unwired: 2 in, 2 out]
        n294 = call "processData.vi"("Cursor List"=w633, "data in"=w632) -> ("Angle Chart"=w630:dbl[][], "Energy Chart"=w631:dbl[][], "Intensity Chart"=w627:dbl[])  [unwired: 1 in]
        n295 = Bundle("Array"=w628, "Intensity Chart"=w627) -> (w629:cluster{"Array":dbl[], "Intensity Chart":dbl[]})  [unwired: 1 in]
        n296 = local write "energygraph"(w631) -> ()
        n297 = local write "intensitygraph"(w629) -> ()
        n298 = local write "anglegraph"(w630) -> ()
      }
    }
  }
  n299 = while {
    tunnel: w24 -> [w643]
    tunnel: w23 -> [w642]
    tunnel: w22 -> [w641]
    tunnel: w21 -> [w640]
    tunnel: w26 -> [w638]
    tunnel: w33 -> [w639]
    tunnel: w8 -> [w637]
    tunnel: w15 -> [w636]
    tunnel: w9 -> [w635]
    tunnel: w3 -> [w634]
    stop <- w644 stop-if-true
    n300 = event shown="[8] \"phoib_standby\": Value Change" {
      selector: _ -> [_ _ _ _ _ _ _ _ _ _ _ _ _ _ _ _ _ _ _ _ _ _ _ _ _ _ _ _ _ _ _ _ _ _ _ _]
      dyn-events: _ -> [_ _ _ _ _ _ _ _ _ _ _ _ _ _ _ _ _ _ _ _ _ _ _ _ _ _ _ _ _ _ _ _ _ _ _ _]
      timeout: _ -> [_ _ _ _ _ _ _ _ _ _ _ _ _ _ _ _ _ _ _ _ _ _ _ _ _ _ _ _ _ _ _ _ _ _ _ _]
      tunnel: [_ TRUE _ _ _ _ _ _ _ _ _ _ _ _ _ _ _ _ _ _ _ _ _ _ _ _ _ _ _ _ _ _ _ _ _ _] -> w644
      tunnel: w643 -> [_ w661 w673 _ _ _ _ _ _ _ w703 w705 _ _ _ _ _ _ _ _ _ _ _ _ _ _ _ _ _ _ _ _ _ _ _ _]
      tunnel: w642 -> [_ w660 _ w677 _ _ _ _ _ _ _ _ _ _ _ _ _ _ _ _ _ _ _ w784 _ _ w806 _ _ _ _ _ _ _ _ _]
      tunnel: w641 -> [_ w659 _ _ w683 _ _ _ _ _ _ _ _ _ _ _ _ _ _ _ w758 w774 w776 _ _ _ _ _ _ _ _ _ _ _ _ _]
      tunnel: w640 -> [_ w658 _ _ _ _ _ w693 w699 w700 _ _ _ _ _ _ _ _ _ _ _ _ _ _ _ _ _ _ _ _ _ _ _ _ _ _]
      tunnel: w639 -> [_ w666 _ _ _ _ _ _ _ _ _ _ _ _ _ _ _ _ _ _ _ _ _ _ _ _ _ _ _ _ _ _ _ _ _ _]
      tunnel: w638 -> [_ w657 _ _ _ _ _ _ _ _ _ _ w707 w709 _ _ _ _ _ _ _ _ _ _ _ _ _ _ _ _ _ _ _ w830 _ _]
      tunnel: w637 -> [_ w665 _ _ _ _ _ _ _ _ _ _ _ _ _ _ _ _ _ _ _ _ _ _ _ _ _ _ _ _ _ _ _ _ _ _]
      tunnel: w636 -> [_ w656 _ _ _ _ _ _ _ _ _ _ _ _ _ w732 _ _ _ _ _ _ _ _ _ _ _ _ _ _ _ _ _ _ w832 w853]
      tunnel: w635 -> [_ w649 _ _ _ _ _ _ _ _ _ _ _ _ _ _ _ _ _ _ _ _ _ _ _ _ _ _ _ _ _ _ _ _ _ _]
      tunnel: w634 -> [_ w647 _ _ _ _ _ _ _ _ _ _ _ _ _ _ _ _ _ _ _ _ _ _ _ _ _ _ _ _ _ _ _ _ _ _]
      event Timeout {
        n301 = event-data() -> ()  [unwired: 1 in, 1 out]
      }
      event "main_close": Value Change {
        w645 = "close" ("element")
        w662 = "release" ("element")
        n302 = event-data() -> ()  [unwired: 1 in, 1 out]
        n303 = Release Notifier(notifier=w665) -> ()  [unwired: 2 in, 3 out]
        n304 = Flush Queue(queue=w661) -> (queue out=w655:refnum<queue>)  [unwired: 1 in, 2 out]
        n305 = Flush Queue(queue=w660) -> (queue out=w654:refnum<queue>)  [unwired: 1 in, 2 out]
        n306 = Flush Queue(queue=w659) -> (queue out=w653:refnum<queue>)  [unwired: 1 in, 2 out]
        n307 = Flush Queue(queue=w658) -> (queue out=w652:refnum<queue>)  [unwired: 1 in, 2 out]
        n308 = Flush Queue(queue=w657) -> (queue out=w651:refnum<queue>)  [unwired: 1 in, 2 out]
        n309 = Flush Queue(queue=w656) -> (queue out=w650:refnum<queue>)  [unwired: 1 in, 2 out]
        n310 = Flush Queue(queue=w649) -> (queue out=w648:refnum<queue>)  [unwired: 1 in, 2 out]
        n311 = Flush Queue(queue=w647) -> (queue out=w646:refnum<queue>)  [unwired: 1 in, 2 out]
        n312 = Release Queue(queue=w666) -> ()  [unwired: 2 in, 3 out]
        n313 = Enqueue Element(queue=w655, element=w662) -> (queue out=w670:refnum<queue>)  [unwired: 2 in, 2 out]
        n314 = Enqueue Element(queue=w654, element=w662) -> (queue out=w669:refnum<queue>)  [unwired: 2 in, 2 out]
        n315 = Enqueue Element(queue=w653, element=w662) -> (queue out=w668:refnum<queue>)  [unwired: 2 in, 2 out]
        n316 = Enqueue Element(queue=w652, element=w662) -> (queue out=w667:refnum<queue>)  [unwired: 2 in, 2 out]
        n317 = Enqueue Element(queue=w650, element=w662) -> (queue out=w664:refnum<queue>, error out=w663:errorcluster)  [unwired: 2 in, 1 out]
        n318 = Enqueue Element(queue=w670, element=w645) -> ()  [unwired: 2 in, 3 out]
        n319 = Enqueue Element(queue=w669, element=w645) -> ()  [unwired: 2 in, 3 out]
        n320 = Enqueue Element(queue=w668, element=w645) -> ()  [unwired: 2 in, 3 out]
        n321 = Enqueue Element(queue=w667, element=w645) -> ()  [unwired: 2 in, 3 out]
        n322 = Enqueue Element(queue=w651, element=w645) -> ()  [unwired: 2 in, 3 out]
        n323 = Enqueue Element(queue=w664, element=w645, error in (no error)=w663) -> ()  [unwired: 1 in, 3 out]
        n324 = Enqueue Element(queue=w648, element=w645) -> ()  [unwired: 2 in, 3 out]
        n325 = Enqueue Element(queue=w646, element=w645) -> ()  [unwired: 2 in, 3 out]
      }
      event "cam_release", "cam_init": Value Change {
        n326 = event-data() -> ()  [unwired: 1 in, 2 out]
        n327 = Select(t="init" ("name (unnamed)"), s="cam_init", f="release" ("name (unnamed)")) -> (s? t:f=w672:string)
        n328 = Enqueue Element(queue=w673, element=w672) -> ()  [unwired: 2 in, 3 out]
      }
      event "ESP_release", "ESP_init": Value Change {
        n329 = event-data() -> ()  [unwired: 1 in, 2 out]
        n330 = Select(t="init" ("name (unnamed)"), s="ESP_init", f="release" ("name (unnamed)")) -> (s? t:f=w681:string)
        n331 = Enqueue Element(queue=w677, element=w681) -> ()  [unwired: 2 in, 3 out]
      }
      event "manip_init", "manip_release": Value Change {
        n332 = event-data() -> ()  [unwired: 1 in, 2 out]
        n333 = Flush Queue(queue=w683) -> (queue out=w682:refnum<queue>)  [unwired: 1 in, 2 out]
        n334 = Select(t="init" ("name (unnamed)"), s="manip_init", f="release" ("name (unnamed)")) -> (s? t:f=w685:string)
        n335 = Enqueue Element(queue=w682, element=w685) -> ()  [unwired: 2 in, 3 out]
      }
      event "setpoint_set": Value Change {
        n336 = event-data() -> ()  [unwired: 1 in, 2 out]
        n337 = local read "LS310  EPICS SP"() -> (w689:string)
        n338 = call-poly <userlib>:"CaLabPut.vi"("Value"="Setpoint", "PV Name"=w689) -> ()  [unwired: 6 in, 4 out]
      }
      event "wattpilot_set": Value Change {
        n339 = event-data() -> ()  [unwired: 1 in, 2 out]
        n340 = local read "WattPilot EPICS chanel set"() -> (w691:string)
        n341 = call-poly <userlib>:"CaLabPut.vi"("Value"="Set Powet (%)", "PV Name"=w691) -> ()  [unwired: 6 in, 4 out]
      }
      event "phoib_release", "phoib_init": Value Change {
        n342 = event-data() -> ()  [unwired: 1 in, 2 out]
        n343 = Flush Queue(queue=w693) -> (queue out=w692:refnum<queue>)  [unwired: 1 in, 2 out]
        n344 = Select(t="init" ("name (unnamed)"), s="phoib_init", f="release" ("name (unnamed)")) -> (s? t:f=w695:string)
        n345 = Enqueue Element(queue=w692, element=w695) -> ()  [unwired: 2 in, 3 out]
      }
      event "phoib_standby": Value Change {
        n346 = event-data() -> ()  [unwired: 1 in, 2 out]
        n347 = Enqueue Element(queue=w699, element="standby") -> ()  [unwired: 2 in, 3 out]
      }
      event "phoib_set": Value Change {
        n348 = event-data() -> ()  [unwired: 1 in, 2 out]
        n349 = Enqueue Element(queue=w700, element="set") -> ()  [unwired: 2 in, 3 out]
      }
      event "cam_dark": Value Change {
        n350 = event-data() -> ()  [unwired: 1 in, 2 out]
        n351 = Enqueue Element(queue=w703, element="dark") -> ()  [unwired: 2 in, 3 out]
      }
      event "ROI Left", "ROI Right", "ROI Top", "ROI Bottom", "cam_exp", "binning", "gain": Value Change {
        n352 = event-data() -> ()  [unwired: 1 in, 1 out]
        n353 = Enqueue Element(queue=w705, element="set") -> ()  [unwired: 2 in, 3 out]
      }
      event "cam_saveimg": Value Change {
        n354 = event-data() -> ()  [unwired: 1 in, 1 out]
        n355 = Enqueue Element(queue=w707, element="single") -> ()  [unwired: 2 in, 3 out]
      }
      event "scan_go": Value Change {
        n356 = event-data() -> ()  [unwired: 1 in, 1 out]
        n357 = Enqueue Element(queue=w709, element="scan") -> ()  [unwired: 2 in, 3 out]
      }
      event "meas_iter", "waypointsD1", "waypointsD2": Value Change {
        n358 = event-data() -> ()  [unwired: 1 in, 6 out]
        n359 = local read "waypointsD2"() -> (w720:string[][])
        n360 = local read "waypointsD1"() -> (w730:string[][])
        n361 = call "create scan vectr.vi"("Table Control"=w720) -> ("Array"=w719:dbl[])
        n362 = call "create scan vectr.vi"("Table Control"=w730) -> ("Array"=w729:dbl[])
        n363 = Array Size(array=w719) -> (size(s)=w717:i32)
        n364 = Array Size(array=w729) -> (size(s)=w713:i32)
        n365 = local read "meas_iter"() -> (w725:i32)
        n366 = local read "binning"() -> (w727:u16)
        n367 = Equal To 0?(x=w717) -> (x = 0?=w718:bool)
        n368 = Select(t=1, s=w718, f=w717) -> (s? t:f=w715:i32)
        n369 = Index Array(array=dbl[] [8.79, 2.2, 0.553, 0.138], index=w727) -> (element=w724:dbl)
        n370 = Multiply(x=w715, y=w713) -> (x*y=w714:i32)
        "measpoints" <- w714
        n371 = Multiply(x=w714, y=w725) -> (x*y=w722:i32)
        "total steps" <- w722
        n372 = Get Date/Time In Seconds() -> (seconds since 1Jan1904=w712:timestamp)
        n373 = Multiply(x=w722, y=w724) -> (x*y=→"disk [MB]":dbl)
        n374 = Multiply(x=w722, y="time/step [s]") -> (x*y=w711:dbl)
        "duration [HH:MM:SS]" <- w711
        n375 = Multiply(x=w713, y=w724) -> (x*y=→"RAM [MB]":dbl)
        n376 = Add(x=w712, y=w711) -> (x+y=→"ETA 2":timestamp)
      }
      event "mirr_go": Value Change {
        n377 = event-data() -> ()  [unwired: 1 in, 1 out]
        n378 = Index Array(array="mirr_dest") -> (element #1=w737:i32, element #2=w736:i32)  [unwired: 2 in]
        n379 = Format Into String(format string="%g_%g", w737, w736) -> (resulting string=w734:string)  [unwired: 2 in, 1 out]
        n380 = Concatenate Strings("abs:" ("string"), w734) -> (w731:string)
        n381 = Enqueue Element(queue=w732, element=w731) -> ()  [unwired: 2 in, 3 out]
      }
      event "scan_manip_setstart": Value Change {
        n382 = event-data() -> ()  [unwired: 1 in, 1 out]
        n383 = local read "pos"() -> (w739:dbl[])
        n384 = local write "scan_manip_start"(w739) -> ()
      }
      event "scan_manip_setstart 2": Value Change {
        n385 = event-data() -> ()  [unwired: 1 in, 1 out]
        n386 = local read "pos"() -> (w740:dbl[])
        n387 = local write "scan_manip_start 2"(w740) -> ()
      }
      event "scan_mirr_setstart": Value Change {
        n388 = event-data() -> ()  [unwired: 1 in, 1 out]
        n389 = local read "mirr_posX"() -> (w743:i32)
        n390 = local read "mirr_posY"() -> (w742:i32)
        n391 = Build Array(w743, w742) -> (w741:i32[])
        n392 = local write "scan_mirr_start"(w741) -> ()
      }
      event "scan_mirr_setstart 2": Value Change {
        n393 = event-data() -> ()  [unwired: 1 in, 1 out]
        n394 = local read "mirr_posX"() -> (w746:i32)
        n395 = local read "mirr_posY"() -> (w745:i32)
        n396 = Build Array(w746, w745) -> (w744:i32[])
        n397 = local write "scan_mirr_start 2"(w744) -> ()
      }
      event "Move Abs": Value Change {
        n398 = event-data() -> ()  [unwired: 1 in, 1 out]
        n399 = Index Array(array="dest") -> (element #1=w756:dbl, element #2=w755:dbl, element #3=w754:dbl, element #4=w753:dbl, element #5=w752:dbl, element #6=w751:dbl)  [unwired: 6 in]
        n400 = Format Into String(format string="%g_%g_%g_%g_%g_%g", w756, w755, w754, w753, w752, w751) -> (resulting string=w749:string)  [unwired: 2 in, 1 out]
        n401 = Concatenate Strings("abs:" ("string"), w749) -> (w748:string)
        n402 = Enqueue Element(queue=w758, element=w748) -> ()  [unwired: 2 in, 3 out]
      }
      event "ManipRel +", "ManipRel -": Value Change {
        n403 = event-data() -> ()  [unwired: 1 in, 2 out]
        n404 = Negate(x="manip_deltas") -> (-x=w762:dbl[])
        n405 = Select(t="manip_deltas", s="ManipRel +", f=w762) -> (s? t:f=w760:dbl[])
        n406 = Index Array(array=w760) -> (element #1=w766:dbl, element #2=w767:dbl, element #3=w768:dbl, element #4=w769:dbl, element #5=w770:dbl, element #6=w771:dbl)  [unwired: 6 in]
        n407 = Format Into String(format string="%g_%g_%g_%g_%g_%g", w766, w767, w768, w769, w770, w771) -> (resulting string=w773:string)  [unwired: 2 in, 1 out]
        n408 = Concatenate Strings("rel:" ("string"), w773, ":wait" ("string")) -> (w764:string)
        n409 = Enqueue Element(queue=w774, element=w764) -> ()  [unwired: 2 in, 3 out]
      }
      event "stop manip": Value Change {
        n410 = event-data() -> ()  [unwired: 1 in, 1 out]
        n411 = Enqueue Element(queue=w776, element="stop") -> ()  [unwired: 2 in, 3 out]
      }
      event "ESP_go": Value Change {
        w778 = ":" ("string")
        n412 = event-data() -> ()  [unwired: 1 in, 1 out]
        n413 = Number To Decimal String(number=0) -> (decimal integer string=w780:string)  [unwired: 1 in]
        n414 = Number To Fractional String(number="ESP_dest") -> (F-format string=w779:string)  [unwired: 3 in]
        n415 = Concatenate Strings("abs:" ("string"), w780, w778, w779, w778) -> (w783:string)
        n416 = Enqueue Element(queue=w784, element=w783) -> ()  [unwired: 2 in, 3 out]
      }
      event "ESP_set_t0": Value Change {
        n417 = event-data() -> ()  [unwired: 1 in, 1 out]
        n418 = Current VI's Path() -> (path=w795:path)
        n419 = Strip Path(path=w795) -> (stripped path=w793:path)  [unwired: 1 out]
        n420 = Strip Path(path=w793) -> (stripped path=w792:path)  [unwired: 1 out]
        n421 = local read "ESP_pos"() -> (w794:dbl)
        "ESP_t0" <- w794
        n422 = Number To Fractional String(number=w794) -> (F-format string=w787:string)  [unwired: 3 in]
        n423 = Build Path(base path=w792, name or relative path="t0.txt") -> (appended path=w789:path)
        n424 = Get Date/Time In Seconds() -> (seconds since 1Jan1904=w791:timestamp)
        n425 = Format Date/Time String(time format string (%c)="%Y.%m.%d %H:%M", seconds (now)=w791) -> (date/time string=w788:string)  [unwired: 1 in]
        n426 = Build Array(w788, w787) -> (w786:string[])
        n427 = call-poly <vilib>:"Write Delimited Spreadsheet.vi"("file path (dialog if empty)"=w789, "1D data"=w786, "append to file? (new file:F)"=TRUE ("append to file? (F)")) -> ()  [unwired: 11 in, 2 out]
      }
      event "ESP_opent0file": Value Change {
        n428 = event-data() -> ()  [unwired: 1 in, 6 out]
        n429 = Current VI's Path() -> (path=w799:path)
        n430 = Strip Path(path=w799) -> (stripped path=w798:path)  [unwired: 1 out]
        n431 = Strip Path(path=w798) -> (stripped path=w800:path)  [unwired: 1 out]
        n432 = call <vilib>:"System Exec.vi"("wait until completion? (T)"=FALSE, "working directory"=w800, "command line"="notepad t0.txt") -> ()  [unwired: 5 in, 4 out]
      }
      event "ESP_+", "ESP_-": Value Change {
        n433 = event-data() -> ()  [unwired: 1 in, 6 out]
        n434 = Negate(x="ESP_delta") -> (-x=w809:dbl)
        n435 = Select(t="ESP_delta", s="ESP_+", f=w809) -> (s? t:f=w807:dbl)
        n436 = Number To Decimal String(number=0) -> (decimal integer string=w805:string)  [unwired: 1 in]
        n437 = Number To Fractional String(number=w807) -> (F-format string=w803:string)  [unwired: 3 in]
        n438 = Concatenate Strings("rel:" ("string"), w805, ":" ("string"), w803) -> (w812:string)
        n439 = Enqueue Element(queue=w806, element=w812) -> ()  [unwired: 2 in, 3 out]
      }
      event "ESP_dest": Value Change {
        n440 = event-data() -> ()  [unwired: 1 in, 6 out]
        n441 = local read "ESP_dest"() -> (w816:dbl)
        n442 = local read "ESP_t0"() -> (w815:dbl)
        n443 = call "mm2time.vi"("fs?"=TRUE ("fs[1]/ps[0]"), "Offset (mm)"=w815, "distance (mm)"=w816) -> ("time in fs/ps seconds"=w813:dbl)
        n444 = local write "ESP_dest_t"(w813) -> ()
      }
      event "ESP_dest_t": Value Change {
        n445 = event-data() -> ()  [unwired: 1 in, 1 out]
        n446 = local read "ESP_t0"() -> (w819:dbl)
        n447 = call "time2mm.vi"("fs[1]/ps[0]"=TRUE, "Offset (mm)"=w819, "time"="ESP_dest_t") -> ("position (mm)"=w817:dbl)
        n448 = local write "ESP_dest"(w817) -> ()
      }
      event "load waypoints 1": Value Change {
        n449 = event-data() -> ()  [unwired: 1 in, 6 out]
        n450 = call-poly <vilib>:"Read Delimited Spreadsheet.vi"() -> ("all rows"=w822:string[][], "error out"=w821:errorcluster)  [unwired: 10 in, 4 out]
        n451 = case shown="No Error" w821 {
          tunnel: w822 -> [w823 _]
          frame No Error {
            n452 = local write "waypointsD1"(w823) -> ()
          }
          frame Error {
          }
        }
      }
      event "load waypoints 2": Value Change {
        n453 = event-data() -> ()  [unwired: 1 in, 6 out]
        n454 = call-poly <vilib>:"Read Delimited Spreadsheet.vi"() -> ("all rows"=w825:string[][], "error out"=w824:errorcluster)  [unwired: 10 in, 4 out]
        n455 = case shown="No Error" w824 {
          tunnel: w825 -> [w826 _]
          frame No Error {
            n456 = local write "waypointsD2"(w826) -> ()
          }
          frame Error {
          }
        }
      }
      event "clear waypoints 1": Value Change {
        n457 = event-data() -> ()  [unwired: 1 in, 6 out]
        n458 = local write "waypointsD1"(string[][] []) -> ()
      }
      event "clear waypoints 2": Value Change {
        n459 = event-data() -> ()  [unwired: 1 in, 6 out]
        n460 = local write "waypointsD2"(string[][] []) -> ()
      }
      event "mainimg": Cursor Release {
        n461 = event-data() -> ()  [unwired: 1 in, 1 out]
        n462 = Enqueue Element(queue=w830, element="refresh") -> ()  [unwired: 2 in, 3 out]
      }
      event "mirr_init", "mirr_release": Value Change {
        n463 = event-data() -> ()  [unwired: 1 in, 6 out]
        n464 = Flush Queue(queue=w832) -> (queue out=w833:refnum<queue>)  [unwired: 1 in, 2 out]
        n465 = Select(t="init" ("name (unnamed)"), s="mirr_init", f="release" ("name (unnamed)")) -> (s? t:f=w834:string)
        n466 = Enqueue Element(queue=w833, element=w834) -> ()  [unwired: 2 in, 3 out]
      }
      event "mirr_X-", "mirr_X+", "mirr_Y+", "mirr_Y-": Value Change {
        n467 = event-data() -> ()  [unwired: 1 in, 1 out]
        n468 = local read "mirr_X#"() -> (w844:u8)
        n469 = local read "mirr_Y#"() -> (w843:u8)
        n470 = Or(x="mirr_X+", y="mirr_X-") -> (x .or. y?=w845:bool)
        n471 = Or(x="mirr_X-", y="mirr_Y-") -> (x .or. y?=w851:bool)
        n472 = Negate(x="mirr_rel") -> (-x=w850:i32)
        n473 = Select(t=w844, s=w845, f=w843) -> (s? t:f=w842:u8)
        n474 = Select(t=w850, s=w851, f="mirr_rel") -> (s? t:f=w839:i32)
        n475 = Number To Decimal String(number=w842) -> (decimal integer string=w841:string)  [unwired: 1 in]
        n476 = Number To Decimal String(number=w839) -> (decimal integer string=w838:string)  [unwired: 1 in]
        n477 = Concatenate Strings("rel:" ("string"), w841, ":" ("string"), w838) -> (w837:string)
        n478 = Enqueue Element(queue=w853, element=w837) -> ()  [unwired: 2 in, 3 out]
      }
    }
  }
  n479 = while {
    tunnel: w15 -> [w862]
    shift-right: [w859] -> _
    shift-left: _ -> [w860]
    tunnel: w8 -> [w858]
    shift-right: [w857] -> _
    shift-left: _ -> [w856]
    shift-right: [w854] -> _
    shift-left: _ -> [w855]
    stop <- w861 stop-if-true
    # "mirr"
    n480 = Preview Queue Element(queue=w862, timeout in ms (-1)=w860) -> (queue out=w865:refnum<queue>, element=w866:string)  [unwired: 1 in, 2 out]
    n481 = Match Pattern(string=w866, regular expression=":") -> (before substring=w864:string, after substring=w863:string)  [unwired: 1 in, 2 out]
    n482 = case shown="\"idle\", Default" w864 {
      tunnel: w865 -> [w901 w911 w926 w930 w933 w938 _]
      tunnel: w863 -> [w895 w912 _ _ _ _ _]
      tunnel: [_ _ _ TRUE _ _ _] -> w861
      tunnel: [_ _ _ _ -1 _ _] -> w859
      tunnel: w858 -> [w868 _ _ _ _ _ _]
      tunnel: [w887 w908 refnum<visa-resource-name> refnum ("VISA resource name out") w928 w932 w937 w943] -> w857
      tunnel: w856 -> [w900 w910 w925 w928 w932 _ w947]
      tunnel: [w872 w907 w924 w927 w931 w936 w942] -> w854
      tunnel: w855 -> [w899 w909 _ w927 w931 _ w946]
      frame "abs" {
        w883 = u8 20 items=["Echo"=55, "Home"=1, "Move Absolute"=20, "Move Relative"=21, "Move at Constant Speed"=22, "Renumber"=2, "Restore Settings"=36, "Stop"=23] ("Command")
        w898 = u8 20 items=["Echo"=55, "Home"=1, "Move Absolute"=20, "Move Relative"=21, "Move at Constant Speed"=22, "Renumber"=2, "Restore Settings"=36, "Stop"=23] ("Command")
        n483 = Dequeue Element(queue=w901) -> ()  [unwired: 2 in, 4 out]
        n484 = Match Pattern(string=w895, regular expression=":") -> (before substring=w885:string, after substring=w871:string)  [unwired: 1 in, 2 out]
        n485 = Equal?(x=w871, y="wait") -> (x = y?=w869:bool)
        n486 = Scan From String(format string="%g_%g", input string=w885) -> (output 1=w880:dbl, output 2=w879:dbl)  [unwired: 4 in, 3 out]
        n487 = local read "mirr_X#"() -> (w882:u8)
        n488 = Bundle("mirr_X#"=w882, "Command"=w898, w880, "Response Count"=1) -> (w894:T4)  [unwired: 1 in]
        n489 = local read "mirr_Y#"() -> (w881:u8)
        n490 = call "Request Command.vi"("error in (no error)"=w899, "Request"=w894, "VISA resource name"=w900) -> ("error out"=w876:errorcluster, "VISA resource name out"=w877:refnum<visa-resource-name>)  [unwired: 5 in, 2 out]
        n491 = Bundle("mirr_Y#"=w881, "Command"=w883, w879, "Response Count"=1) -> (w878:T5)  [unwired: 1 in]
        n492 = call "Request Command.vi"("error in (no error)"=w876, "Request"=w878, "VISA resource name"=w877) -> ("error out"=w874:errorcluster, "VISA resource name out"=w875:refnum<visa-resource-name>)  [unwired: 5 in, 2 out]
        n493 = local read "mirr_X#"() -> (w892:u8)
        n494 = call "zaber_readpos.vi"("error in (no error)"=w874, "axis"=w892, "VISA in"=w875) -> ("error out"=w888:errorcluster, "position"=w893:i32, "VISA out"=w889:refnum<visa-resource-name>)  [unwired: 6 in]
        n495 = local read "mirr_Y#"() -> (w890:u8)
        n496 = local write "mirr_posX"(w893) -> ()
        n497 = call "zaber_readpos.vi"("error in (no error)"=w888, "axis"=w890, "VISA in"=w889) -> ("error out"=w873:errorcluster, "position"=w891:i32, "VISA out"=w887:refnum<visa-resource-name>)  [unwired: 6 in]
        n498 = local write "mirr_posY"(w891) -> ()
        n499 = case shown="True" w869 {
          tunnel: w873 -> [w902 w906]
          tunnel: [w902 w905] -> w872
          tunnel: w868 -> [_ w904]
          frame False {
          }
          frame True {
            n500 = Send Notification(notification=TRUE, notifier=w904, error in (no error)=w906) -> (error out=w905:errorcluster)  [unwired: 1 out]
          }
        }
      }
      frame "rel" {
        w915 = u8 21 items=["Echo"=55, "Home"=1, "Move Absolute"=20, "Move Relative"=21, "Move at Constant Speed"=22, "Renumber"=2, "Restore Settings"=36, "Stop"=23] ("Command")
        n501 = Dequeue Element(queue=w911) -> ()  [unwired: 2 in, 4 out]
        n502 = Match Pattern(string=w912, regular expression=":") -> (before substring=w917:string, after substring=w916:string)  [unwired: 1 in, 2 out]
        n503 = Decimal String To Number(string=w917) -> (number=w919:i32)  [unwired: 2 in, 1 out]
        n504 = Decimal String To Number(string=w916) -> (number=w920:i32)  [unwired: 2 in, 1 out]
        n505 = Bundle(w919, "Command"=w915, w920, "Response Count"=1) -> (w913:T6)  [unwired: 1 in]
        n506 = call "Request Command.vi"("error in (no error)"=w909, "Request"=w913, "VISA resource name"=w910) -> ("error out"=w907:errorcluster, "VISA resource name out"=w908:refnum<visa-resource-name>)  [unwired: 5 in, 2 out]
      }
      frame "release" {
        n507 = Dequeue Element(queue=w926) -> (queue out=w922:refnum<queue>)  [unwired: 2 in, 3 out]
        n508 = Enqueue Element(queue=w922, element="suspend") -> ()  [unwired: 2 in, 3 out]
        n509 = call "Close.vi"("VISA resource name"=w925) -> ("error out"=w924:errorcluster)  [unwired: 9 in, 1 out]
      }
      frame "close" {
        n510 = Release Queue(queue=w930) -> ()  [unwired: 2 in, 3 out]
      }
      frame "suspend" {
        n511 = Dequeue Element(queue=w933) -> ()  [unwired: 2 in, 4 out]
      }
      frame "init" {
        n512 = Dequeue Element(queue=w938) -> ()  [unwired: 2 in, 4 out]
        n513 = call "Initialize.vi"("VISA resource name"="mirr_VISA") -> ("error out"=w936:errorcluster, "VISA resource name out"=w937:refnum<visa-resource-name>)  [unwired: 8 in, 1 out]
      }
      frame "idle", Default {
        n514 = local read "mirr_X#"() -> (w948:u8)
        n515 = call "zaber_readpos.vi"("error in (no error)"=w946, "axis"=w948, "VISA in"=w947) -> ("error out"=w944:errorcluster, "position"=→"mirr_posX":i32, "VISA out"=w945:refnum<visa-resource-name>)  [unwired: 6 in]
        n516 = local read "mirr_Y#"() -> (w941:u8)
        n517 = call "zaber_readpos.vi"("error in (no error)"=w944, "axis"=w941, "VISA in"=w945) -> ("error out"=w942:errorcluster, "position"=→"mirr_posY":i32, "VISA out"=w943:refnum<visa-resource-name>)  [unwired: 6 in]
      }
    }
    "mirr_Error" <- w854
  }
  n518 = while {
    tunnel: w23 -> [w958]
    shift-right: [w956] -> _
    shift-left: _ -> [w954]
    shift-right: [w955] -> _
    shift-left: _ -> [w953]
    shift-right: [w951] -> _
    shift-left: 0 -> [w952]
    tunnel: w8 -> [w950]
    stop <- w957 stop-if-true
    # "ESP"
    n519 = Preview Queue Element(queue=w958, timeout in ms (-1)=w952) -> (queue out=w961:refnum<queue>, element=w962:string)  [unwired: 1 in, 2 out]
    n520 = Match Pattern(string=w962, regular expression=":") -> (before substring=w960:string, after substring=w959:string)  [unwired: 1 in, 2 out]
    n521 = case shown="\"init\"" w960 {
      tunnel: w961 -> [_ w984 w1004 w1044 w1047 w1054 w1059]
      tunnel: w959 -> [_ w988 w1010 _ _ _ _]
      tunnel: [_ _ _ _ _ TRUE _] -> w957
      tunnel: [w967 w990 w1005 w1042 refnum<visa-resource-name> refnum ("VISA resource name out") w1051 w1058] -> w956
      tunnel: [w968 w991 w1003 w1041 w1049 w1052 w1057] -> w955
      tunnel: w954 -> [w977 w993 w1008 w1042 w1050 w1051 _]
      tunnel: w953 -> [w976 w992 w1009 w1041 _ w1052 _]
      tunnel: [_ _ _ -1 _ _ _] -> w951
      tunnel: w950 -> [_ _ w997 _ _ _ _]
      tunnel: "ESP patch" -> [w974 w983 w996 _ _ _ _]
      frame "idle", Default {
        n522 = Index Array(array=w974) -> (element #1=w973:i32, element #2=w970:i32)  [unwired: 3 in, 1 out]
        n523 = local read "ESP_t0"() -> (w980:dbl)
        n524 = call "Read Actual Position.vi"("error in (no error)"=w976, "Axis (1)"=w973, "VISA resource name"=w977) -> ("error out"=w971:errorcluster, "Position (units)"=w975:dbl, "VISA resource name out"=w972:refnum<visa-resource-name>)  [unwired: 2 in]
        "ESP_pos" <- w975
        n525 = call "mm2time.vi"("fs?"=TRUE, "Offset (mm)"=w980, "distance (mm)"=w975) -> ("time in fs/ps seconds"=→"ESP_delay":dbl)
        n526 = call "Read Actual Position.vi"("error in (no error)"=w971, "Axis (1)"=w970, "VISA resource name"=w972) -> ("error out"=w969:errorcluster, "Position (units)"=→"waveplate position":dbl, "VISA resource name out"=w966:refnum<visa-resource-name>)  [unwired: 2 in]
        n527 = call "Read Actual Position.vi"("error in (no error)"=w969, "VISA resource name"=w966) -> ("error out"=w968:errorcluster, "Position (units)"=→"stage2 position":dbl, "VISA resource name out"=w967:refnum<visa-resource-name>)  [unwired: 3 in]
      }
      frame "rel" {
        n528 = Dequeue Element(queue=w984) -> ()  [unwired: 2 in, 4 out]
        n529 = Match Pattern(string=w988, regular expression=":") -> (before substring=w987:string, after substring=w986:string)  [unwired: 1 in, 2 out]
        n530 = Decimal String To Number(string=w987) -> (number=w982:i32)  [unwired: 2 in, 1 out]
        n531 = Fract/Exp String To Number(string=w986) -> (number=w985:dbl)  [unwired: 3 in, 1 out]
        n532 = Index Array(array=w983, index=w982) -> (element=w981:i32)
        n533 = call "Move Relative.vi"("error in (no error)"=w992, "Position (0 units)"=w985, "Axis (1)"=w981, "VISA resource name"=w993) -> ("error out"=w991:errorcluster, "VISA resource name out"=w990:refnum<visa-resource-name>)  [unwired: 2 in]
      }
      frame "abs" {
        n534 = Dequeue Element(queue=w1004) -> ()  [unwired: 2 in, 4 out]
        n535 = Match Pattern(string=w1010, regular expression=":") -> (before substring=w1011:string, after substring=w1001:string)  [unwired: 1 in, 2 out]
        n536 = Match Pattern(string=w1001, regular expression=":") -> (before substring=w1000:string, after substring=w999:string)  [unwired: 1 in, 2 out]
        n537 = Decimal String To Number(string=w1011) -> (number=w995:i32)  [unwired: 2 in, 1 out]
        n538 = Fract/Exp String To Number(string=w1000) -> (number=w998:dbl)  [unwired: 3 in, 1 out]
        n539 = Index Array(array=w996, index=w995) -> (element=w994:i32)
        n540 = call "Move Absolute.vi"("error in (no error)"=w1009, "Position (0 units)"=w998, "Axis (1)"=w994, "VISA resource name"=w1008) -> ("error out"=w1006:errorcluster, "VISA resource name out"=w1007:refnum<visa-resource-name>)  [unwired: 2 in]
        n541 = case shown="\"wait\"" w999 {
          tunnel: w994 -> [_ w1015]
          tunnel: w1007 -> [w1014 w1031]
          tunnel: w1006 -> [w1013 w1030]
          tunnel: [w1014 w1020] -> w1005
          tunnel: [w1013 w1027] -> w1003
          tunnel: w997 -> [_ w1026]
          frame "", Default {
          }
          frame "wait" {
            n542 = while {
              tunnel: w1015 -> [w1040]
              shift-right: [w1037] -> w1029
              shift-left: w1031 -> [w1039]
              shift-right: [w1036] -> w1028
              shift-left: w1030 -> [w1038]
              stop <- w1035 stop-if-true
              n543 = call "Get Axis Motion Status.vi"("error in (no error)"=w1038, "Axis (1)"=w1040, "VISA resource name"=w1039) -> ("error out"=w1036:errorcluster, "Motion Done"=w1035:bool, "VISA resource name out"=w1037:refnum<visa-resource-name>)  [unwired: 2 in]
            }
            n544 = flat-sequence {
              tunnel: w1029 -> [w1034]
              tunnel: w1028 -> [w1033]
              tunnel: [w1034] -> w1022
              tunnel: [w1033] -> w1021
              frame #0 {
                n545 = Wait (ms)(milliseconds to wait=u32 1000) -> ()  [unwired: 1 out]
              }
            }
            n546 = local read "ESP_t0"() -> (w1024:dbl)
            n547 = call "Read Actual Position.vi"("error in (no error)"=w1021, "Axis (1)"=w1015, "VISA resource name"=w1022) -> ("error out"=w1016:errorcluster, "Position (units)"=w1018:dbl, "VISA resource name out"=w1020:refnum<visa-resource-name>)  [unwired: 2 in]
            n548 = call "mm2time.vi"("fs?"=TRUE, "Offset (mm)"=w1024, "distance (mm)"=w1018) -> ("time in fs/ps seconds"=w1019:dbl)
            n549 = call <vilib>:"Clear Errors.vi"("error in (no error)"=w1016) -> ("error out"=w1017:errorcluster)  [unwired: 5 in, 1 out]
            n550 = local write "ESP_pos"(w1018) -> ()
            n551 = local write "ESP_delay"(w1019) -> ()
            n552 = Send Notification(notification=TRUE, notifier=w1026, error in (no error)=w1017) -> (error out=w1027:errorcluster)  [unwired: 1 out]
          }
        }
      }
      frame "suspend" {
        n553 = Dequeue Element(queue=w1044) -> ()  [unwired: 2 in, 4 out]
      }
      frame "release" {
        n554 = Dequeue Element(queue=w1047) -> (queue out=w1045:refnum<queue>)  [unwired: 2 in, 3 out]
        n555 = call "Close.vi"("VISA resource name"=w1050) -> ("error out"=w1049:errorcluster)  [unwired: 10 in]
        n556 = Enqueue Element(queue=w1045, element="suspend") -> ()  [unwired: 2 in, 3 out]
      }
      frame "close" {
        n557 = Release Queue(queue=w1054) -> ()  [unwired: 2 in, 3 out]
      }
      frame "init" {
        n558 = Dequeue Element(queue=w1059) -> ()  [unwired: 2 in, 4 out]
        n559 = flat-sequence {
          tunnel: [w1062] -> w1056
          tunnel: [w1061] -> w1055
          tunnel: [w1066] -> w1057
          tunnel: [w1067] -> w1058
          tunnel: w1056 -> [w1067]
          tunnel: w1055 -> [w1066]
          frame #0 {
            n560 = local write "ESP_con?"(FALSE ("ESP_con?")) -> ()
          }
          frame #1 {
            n561 = call "Initialize.vi"("VISA resource name"="ESP301 VISA", "Serial Link (RS232)"=enum16{"RS232", "USB"}."RS232") -> ("VISA resource name out"=w1062:refnum<visa-resource-name>, "error out"=w1061:errorcluster)  [unwired: 7 in]
          }
          frame #2 {
            n562 = local write "ESP_con?"(TRUE ("ESP_con?")) -> ()
          }
        }
      }
    }
    "error out" <- w955
  }
  n563 = while {
    tunnel: w22 -> [w1076]
    shift-right: [w1074] -> _
    shift-left: _ -> [w1072]
    shift-right: [w1073] -> _
    shift-left: _ -> [w1071]
    shift-right: [w1069] -> _
    shift-left: 0 -> [w1070]
    tunnel: w8 -> [w1068]
    stop <- w1075 stop-if-true
    # "manip"
    n564 = Preview Queue Element(queue=w1076, timeout in ms (-1)=w1070) -> (queue out=w1079:refnum<queue>, element=w1080:string)  [unwired: 1 in, 2 out]
    n565 = Match Pattern(string=w1080, regular expression=":") -> (before substring=w1078:string, after substring=w1077:string)  [unwired: 1 in, 2 out]
    n566 = case shown="\"init\"" w1078 {
      tunnel: w1079 -> [_ w1092 w1119 w1166 w1204 w1210 w1219 w1224]
      tunnel: w1077 -> [_ _ w1106 w1165 _ _ _ _]
      tunnel: [_ _ _ _ _ _ TRUE _] -> w1075
      tunnel: [w1086 w1094 w1098 w1163 w1206 refnum<k5> refnum ("gateway_connection out") w1217 w1223] -> w1074
      tunnel: [w1085 w1093 w1100 w1162 w1205 w1212 w1216 w1222] -> w1073
      tunnel: w1072 -> [w1088 w1096 w1122 w1156 w1206 w1214 w1217 _]
      tunnel: w1071 -> [w1087 w1095 w1121 w1157 w1205 _ w1216 _]
      tunnel: [_ _ _ _ -1 _ _ _] -> w1069
      tunnel: w1068 -> [_ _ w1097 w1159 _ _ _ _]
      frame "idle", Default {
        n567 = call "sp_manip_get_axis_status.vi"("error in"=w1087, "gateway_connection"=w1088) -> ("error out"=w1085:errorcluster, "axis_out"=w1084:T7, "gateway_connection out"=w1086:refnum<k5>)  [unwired: 5 in, 2 out]
        n568 = for {
          tunnel: w1084 -> [w1091] mode=indexing
          tunnel: [w1090] -> w1083 mode=indexing
          tunnel: [w1089] -> w1082 mode=indexing
          n569 = Unbundle By Name(w1091) -> ("Axis_Position"=w1090:dbl, "moving"=w1089:bool)
        }
        "moving?" <- w1082
        n570 = local write "pos"(w1083) -> ()
      }
      frame "stop" {
        n571 = Dequeue Element(queue=w1092) -> ()  [unwired: 2 in, 4 out]
        n572 = call "sp_manip_abort.vi"("error in"=w1095, "gateway_connection"=w1096) -> ("error out"=w1093:errorcluster, "gateway_connection out"=w1094:refnum<k5>)  [unwired: 6 in, 2 out]
      }
      frame "rel" {
        n573 = Dequeue Element(queue=w1119) -> ()  [unwired: 2 in, 4 out]
        n574 = Match Pattern(string=w1106, regular expression=":") -> (before substring=w1105:string, after substring=w1104:string)  [unwired: 1 in, 2 out]
        n575 = Equal?(x=w1104, y="wait") -> (x = y?=w1102:bool)
        n576 = call "sp_manip_get_axis_status.vi"("error in"=w1121, "gateway_connection"=w1122) -> ("error out"=w1124:errorcluster, "axis_out"=w1111:T7, "gateway_connection out"=w1123:refnum<k5>)  [unwired: 5 in, 2 out]
        n577 = Scan From String(format string="%g_%g_%g_%g_%g_%g", input string=w1105) -> (output 1=w1118:dbl, output 2=w1117:dbl, output 3=w1116:dbl, output 4=w1115:dbl, output 5=w1114:dbl, output 6=w1113:dbl)  [unwired: 8 in, 3 out]
        n578 = for {
          tunnel: w1111 -> [w1151] mode=indexing
          tunnel: [w1150] -> w1109 mode=indexing
          tunnel: [w1149] -> w1110 mode=indexing
          n579 = Unbundle By Name(w1151) -> ("Axis_Name"=w1150:string, "Axis_Position"=w1149:dbl)
        }
        n580 = Build Array(w1118, w1117, w1116, w1115, w1114, w1113) -> (w1112:dbl[])
        n581 = Add(x=w1110, y=w1112) -> (x+y=w1108:dbl[])
        n582 = call "sp_manip_start_move.vi"("error in"=w1124, "target positions"=w1108, "axis names"=w1109, "gateway_connection"=w1123) -> ("error out"=w1101:errorcluster, "gateway_connection out"=w1099:refnum<k5>)  [unwired: 4 in, 2 out]
        n583 = case shown="True" w1102 {
          tunnel: w1101 -> [w1125 w1136]
          tunnel: [w1125 w1135] -> w1100
          tunnel: w1099 -> [w1126 w1137]
          tunnel: [w1126 w1129] -> w1098
          tunnel: w1097 -> [_ w1134]
          frame False {
          }
          frame True {
            n584 = while {
              tunnel: w1137 -> [w1143]
              tunnel: w1136 -> [w1142]
              tunnel: [w1141] -> w1130
              tunnel: [w1140] -> w1128
              stop <- w1144 continue-if-true
              n585 = call "sp_manip_get_axis_status.vi"("error in"=w1142, "gateway_connection"=w1143) -> ("error out"=w1140:errorcluster, "axis_out"=w1146:T7, "gateway_connection out"=w1141:refnum<k5>)  [unwired: 5 in, 2 out]
              n586 = for {
                tunnel: w1146 -> [w1148] mode=indexing
                tunnel: [w1147] -> w1145 mode=indexing
                n587 = Unbundle By Name(w1148) -> ("moving"=w1147:bool)
              }
              n588 = Or Array Elements(Boolean array=w1145) -> (logical OR=w1144:bool)
            }
            n589 = call "sp_manip_get_axis_status.vi"("error in"=w1128, "gateway_connection"=w1130) -> ("error out"=w1127:errorcluster, "axis_out"=w1132:T7, "gateway_connection out"=w1129:refnum<k5>)  [unwired: 5 in, 2 out]
            n590 = for {
              tunnel: w1132 -> [w1139] mode=indexing
              tunnel: [w1138] -> w1131 mode=indexing
              n591 = Unbundle By Name(w1139) -> ("Axis_Position"=w1138:dbl)
            }
            n592 = Send Notification(notification=TRUE, notifier=w1134, error in (no error)=w1127) -> (error out=w1135:errorcluster)  [unwired: 1 out]
            n593 = local write "dest"(w1131) -> ()
          }
        }
      }
      frame "abs" {
        n594 = Dequeue Element(queue=w1166) -> ()  [unwired: 2 in, 4 out]
        n595 = call "sp_manip_get_axis_status.vi"("error in"=w1157, "gateway_connection"=w1156) -> ("error out"=w1152:errorcluster, "axis_out"=w1155:T7, "gateway_connection out"=w1153:refnum<k5>)  [unwired: 5 in, 2 out]
        n596 = Match Pattern(string=w1165, regular expression=":") -> (before substring=w1169:string, after substring=w1168:string)  [unwired: 1 in, 2 out]
        n597 = Equal?(x=w1168, y="wait") -> (x = y?=w1158:bool)
        n598 = for {
          tunnel: w1155 -> [w1179] mode=indexing
          tunnel: [w1178] -> w1154 mode=indexing
          n599 = Unbundle By Name(w1179) -> ("Axis_Name"=w1178:string)
        }
        n600 = Scan From String(format string="%g_%g_%g_%g_%g_%g", input string=w1169) -> (output 1=w1175:dbl, output 2=w1174:dbl, output 3=w1173:dbl, output 4=w1172:dbl, output 5=w1171:dbl, output 6=w1170:dbl)  [unwired: 8 in, 3 out]
        n601 = Build Array(w1175, w1174, w1173, w1172, w1171, w1170) -> (w1177:dbl[])
        n602 = call "sp_manip_start_move.vi"("error in"=w1152, "target positions"=w1177, "axis names"=w1154, "gateway_connection"=w1153) -> ("error out"=w1161:errorcluster, "gateway_connection out"=w1160:refnum<k5>)  [unwired: 4 in, 2 out]
        n603 = case shown="True" w1158 {
          tunnel: w1161 -> [w1180 w1191]
          tunnel: [w1180 w1190] -> w1162
          tunnel: w1160 -> [w1181 w1192]
          tunnel: [w1181 w1183] -> w1163
          tunnel: w1159 -> [_ w1189]
          frame False {
          }
          frame True {
            n604 = while {
              tunnel: w1192 -> [w1198]
              tunnel: w1191 -> [w1197]
              tunnel: [w1196] -> w1185
              tunnel: [w1195] -> w1184
              stop <- w1199 continue-if-true
              n605 = call "sp_manip_get_axis_status.vi"("error in"=w1197, "gateway_connection"=w1198) -> ("error out"=w1195:errorcluster, "axis_out"=w1201:T7, "gateway_connection out"=w1196:refnum<k5>)  [unwired: 5 in, 2 out]
              n606 = for {
                tunnel: w1201 -> [w1203] mode=indexing
                tunnel: [w1202] -> w1200 mode=indexing
                n607 = Unbundle By Name(w1203) -> ("moving"=w1202:bool)
              }
              n608 = Or Array Elements(Boolean array=w1200) -> (logical OR=w1199:bool)
            }
            n609 = call "sp_manip_get_axis_status.vi"("error in"=w1184, "gateway_connection"=w1185) -> ("error out"=w1182:errorcluster, "axis_out"=w1187:T7, "gateway_connection out"=w1183:refnum<k5>)  [unwired: 5 in, 2 out]
            n610 = for {
              tunnel: w1187 -> [w1194] mode=indexing
              tunnel: [w1193] -> w1186 mode=indexing
              n611 = Unbundle By Name(w1194) -> ("Axis_Position"=w1193:dbl)
            }
            n612 = local write "pos"(w1186) -> ()
            n613 = Send Notification(notification=TRUE, notifier=w1189, error in (no error)=w1182) -> (error out=w1190:errorcluster)  [unwired: 1 out]
          }
        }
      }
      frame "suspend" {
        n614 = Dequeue Element(queue=w1204) -> ()  [unwired: 2 in, 4 out]
      }
      frame "release" {
        n615 = Dequeue Element(queue=w1210) -> (queue out=w1208:refnum<queue>)  [unwired: 2 in, 3 out]
        n616 = call "sp_manip_disconnect.vi"("gateway_connection"=w1214) -> ("error out"=w1213:errorcluster, "gateway_connection_out"=w1215:refnum<k5>)  [unwired: 7 in, 2 out]
        n617 = call "tcp_gateway_close_connection.vi"("error in"=w1213, "server_connection"=w1215) -> ("error out"=w1212:errorcluster)  [unwired: 5 in]
        n618 = Enqueue Element(queue=w1208, element="suspend") -> ()  [unwired: 2 in, 3 out]
      }
      frame "close" {
        n619 = Release Queue(queue=w1219) -> ()  [unwired: 2 in, 3 out]
      }
      frame "init" {
        n620 = Dequeue Element(queue=w1224) -> ()  [unwired: 2 in, 4 out]
        n621 = flat-sequence {
          tunnel: [w1227] -> w1221
          tunnel: [w1226] -> w1220
          tunnel: [w1237] -> w1222
          tunnel: [w1238] -> w1223
          tunnel: w1221 -> [w1238]
          tunnel: w1220 -> [w1237]
          frame #0 {
            n622 = local write "manip_con?"(FALSE ("manip_con?")) -> ()
          }
          frame #1 {
            n623 = call "tcp_gateway_open_connection.vi"() -> ("gateway_connection"=w1230:refnum<k5>, "error out"=w1229:errorcluster)  [unwired: 5 in, 3 out]
            n624 = call "sp_manip_connect.vi"("error in"=w1229, "gateway_connection"=w1230) -> ("error out"=w1226:errorcluster, "axis_out"=w1228:T7, "gateway_connection out"=w1227:refnum<k5>)  [unwired: 5 in, 2 out]
            n625 = for {
              tunnel: w1228 -> [w1235] mode=indexing
              tunnel: [w1234] -> w1231 mode=indexing
              tunnel: [w1233] -> w1232 mode=indexing
              n626 = Unbundle By Name(w1235) -> ("Axis_Name"=w1234:string, "Axis_Position"=w1233:dbl)
            }
            "axis" <- w1231
            "pos" <- w1232
            n627 = local write "dest"(w1232) -> ()
          }
          frame #2 {
            n628 = local write "manip_con?"(TRUE ("manip_con?")) -> ()
          }
        }
      }
    }
    "error out 2" <- w1073
  }
  n629 = while {
    tunnel: w21 -> [w1249]
    shift-right: [w1244] -> _
    shift-left: 0 -> [w1247]
    tunnel: string[] ["Kinetic Energy", "Pass Energy", "Coil Current", "Work Function", "Detector Voltage", "Screen Voltage", "Conversion Voltage", "Focus Displacement 1", "Mesh Front", "Mesh Back"] -> [w1246]
    tunnel: w8 -> [w1245]
    tunnel: w1 -> [w1243]
    shift-right: [w1240] -> _
    shift-left: _ -> [w1242]
    shift-right: [w1239] -> _
    shift-left: _ -> [w1241]
    stop <- w1248 stop-if-true
    # "phoib"
    n630 = Preview Queue Element(queue=w1249, timeout in ms (-1)=w1247) -> (queue out=w1252:refnum<queue>, element=w1253:string)  [unwired: 1 in, 2 out]
    n631 = Match Pattern(string=w1253, regular expression=":") -> (before substring=w1251:string, after substring=w1250:string)  [unwired: 1 in, 2 out]
    n632 = case shown="\"set\"" w1251 {
      tunnel: w1252 -> [_ w1317 w1367 w1410 w1419 w1430 w1434 w1439]
      tunnel: w1250 -> [_ _ w1364 _ _ _ _ _]
      tunnel: [_ _ _ _ _ TRUE _ _] -> w1248
      tunnel: w1246 -> [_ _ _ _ _ _ _ _]
      tunnel: w1245 -> [_ _ w1365 _ _ _ _ _]
      tunnel: [_ _ _ _ _ _ -1 _] -> w1244
      tunnel: w1243 -> [w1267 w1303 w1346 _ _ _ _ _]
      tunnel: w1242 -> [w1266 w1307 w1357 w1409 w1416 w1428 w1432 _]
      tunnel: w1241 -> [w1265 w1306 w1356 w1408 w1415 w1427 w1431 _]
      tunnel: [w1264 w1302 w1337 w1407 w1412 w1428 w1432 w1437] -> w1240
      tunnel: [w1263 w1301 w1349 w1406 w1413 w1427 w1431 w1436] -> w1239
      frame "idle", Default {
        n633 = for {
          tunnel: w1266 -> [w1276]
          tunnel: w1265 -> [w1274]
          tunnel: w1267 -> [w1275] mode=indexing
          tunnel: [w1271] -> w1262 mode=indexing
          tunnel: [w1270] -> w1264
          tunnel: [w1269] -> w1263
          n634 = call "GetAnalyzerParameterValue.vi"("error in"=w1274, "Parameter Name"=w1275, "connection ID in"=w1276) -> ("error out"=w1269:errorcluster, "Parameter"=w1273:cluster{"Name":string, "Value":string}, "connection ID out"=w1270:refnum<k5>)  [unwired: 3 in, 3 out]
          n635 = Unbundle(w1273) -> ("Value"=w1272:string)  [unwired: 1 out]
          n636 = Fract/Exp String To Number(use system decimal point (T)=FALSE, string=w1272) -> (number=w1271:dbl)  [unwired: 2 in, 1 out]
        }
        n637 = Index Array(array=w1262) -> (element #1=→"phoib_I_3":dbl, element #2=→"phoib_I_5":dbl, element #3=→"phoib_I_6":dbl, element #4=→"phoib_I_8":dbl, element #5=→"phoib_I_9":dbl, element #6=→"phoib_I_10":dbl, element #7=→"phoib_I_7":dbl)  [unwired: 7 in]
      }
      frame "set" {
        n638 = Dequeue Element(queue=w1317) -> ()  [unwired: 2 in, 4 out]
        n639 = Number To Fractional String(use system decimal point (T)=FALSE, number="phoib_I_1s") -> (F-format string=w1297:string)  [unwired: 2 in]
        n640 = Number To Fractional String(use system decimal point (T)=FALSE, number="phoib_I_2s") -> (F-format string=w1296:string)  [unwired: 2 in]
        n641 = Concatenate Strings("\"Pass Energy\":" ("string"), w1296) -> (w1295:string)
        n642 = Concatenate Strings("\"Kinetic Energy\":" ("string"), w1297) -> (w1294:string)
        n643 = Concatenate Strings("LensMode:\"" ("string"), "lens_mode", "\"" ("string")) -> (w1298:string)
        n644 = Concatenate Strings("ScanRange:\"" ("string"), "scan_range", "\"" ("string")) -> (w1299:string)
        n645 = Concatenate Strings("Polarity:\"" ("string"), "negative" ("string"), "\"" ("string")) -> (w1300:string)
        n646 = Build Array(w1298, w1299, w1300, w1294, w1295) -> (w1278:string[])
        n647 = Build Array("phoib_I_3s", "phoib_I_5s", "phoib_I_6s", "phoib_I_8s", "phoib_I_9s", "phoib_I_10s", "phoib_I_7s") -> (w1316:dbl[])
        n648 = call "SetAnalyzerParameterDirectly.vi"("error in"=w1306, "Set Parameter List"=w1278, "connection ID in"=w1307) -> ("error out"=w1304:errorcluster, "connection ID out"=w1305:refnum<k5>)  [unwired: 4 in, 3 out]
        n649 = Number To Fractional String(use system decimal point (T)=FALSE, number=w1316) -> (F-format string=w1308:string[])  [unwired: 2 in]
        n650 = for {
          tunnel: w1305 -> [w1327]
          tunnel: w1304 -> [w1326]
          tunnel: [w1334] -> w1302
          tunnel: [w1333] -> w1301
          tunnel: w1303 -> [w1322] mode=indexing
          tunnel: w1308 -> [w1321] mode=indexing
          w1318 = FALSE ("use system decimal point (T)")
          n651 = call "GetAnalyzerParameterInfo.vi"("error in"=w1326, "Parameter Name"=w1322, "connection ID in"=w1327) -> ("error out"=w1324:errorcluster, "Parameter Info"=w1323:T8, "connection ID out"=w1325:refnum<k5>)  [unwired: 3 in, 3 out]
          n652 = Unbundle(w1323) -> ("Min"=w1332:string, "Max"=w1331:string)  [unwired: 5 out]
          n653 = Fract/Exp String To Number(use system decimal point (T)=w1318, string=w1331) -> (number=w1329:dbl)  [unwired: 2 in, 1 out]
          n654 = Fract/Exp String To Number(use system decimal point (T)=w1318, string=w1321) -> (number=w1330:dbl)  [unwired: 2 in, 1 out]
          n655 = Fract/Exp String To Number(use system decimal point (T)=w1318, string=w1332) -> (number=w1328:dbl)  [unwired: 2 in, 1 out]
          n656 = In Range and Coerce(upper limit=w1329, x=w1330, lower limit=w1328) -> (coerced(x)=w1319:dbl)  [unwired: 1 out]
          n657 = Number To Fractional String(number=w1319) -> (F-format string=w1320:string)  [unwired: 3 in]
          n658 = call "SetAnalyzerParameterValue.vi"("error in"=w1324, "Parameter Value"=w1320, "Parameter Name"=w1322, "connection ID in"=w1325) -> ("error out"=w1333:errorcluster, "connection ID out"=w1334:refnum<k5>)  [unwired: 3 in, 3 out]
        }
      }
      frame "setsgl" {
        w1335 = FALSE ("use system decimal point (T)")
        n659 = Dequeue Element(queue=w1367) -> ()  [unwired: 2 in, 4 out]
        n660 = Match Pattern(string=w1364, regular expression=":") -> (before substring=w1352:string, after substring=w1351:string)  [unwired: 1 in, 2 out]
        n661 = call "GetAnalyzerParameterInfo.vi"("error in"=w1356, "Parameter Name"=w1352, "connection ID in"=w1357) -> ("error out"=w1354:errorcluster, "Parameter Info"=w1363:T8, "connection ID out"=w1355:refnum<k5>)  [unwired: 3 in, 3 out]
        n662 = Unbundle(w1363) -> ("Min"=w1362:string, "Max"=w1361:string)  [unwired: 5 out]
        n663 = Fract/Exp String To Number(use system decimal point (T)=w1335, string=w1361) -> (number=w1359:dbl)  [unwired: 2 in, 1 out]
        n664 = Fract/Exp String To Number(use system decimal point (T)=w1335, string=w1351) -> (number=w1360:dbl)  [unwired: 2 in, 1 out]
        n665 = Fract/Exp String To Number(use system decimal point (T)=w1335, string=w1362) -> (number=w1358:dbl)  [unwired: 2 in, 1 out]
        n666 = In Range and Coerce(upper limit=w1359, x=w1360, lower limit=w1358) -> (In Range?=w1353:bool)  [unwired: 1 out]
        n667 = case shown="True" w1353 {
          tunnel: [FALSE ("notification") TRUE ("notification")] -> w1350
          tunnel: [w1378 w1392] -> w1348
          tunnel: [w1377 w1384] -> w1347
          tunnel: w1352 -> [_ w1383]
          tunnel: w1355 -> [w1378 w1382]
          tunnel: w1354 -> [w1377 w1381]
          tunnel: w1351 -> [_ w1380]
          frame False {
          }
          frame True {
            n668 = Fract/Exp String To Number(string=w1380) -> (number=w1388:dbl)  [unwired: 3 in, 1 out]
            n669 = Multiply(x=0.01, y=w1388) -> (x*y=w1387:dbl)
            n670 = call "SetAnalyzerParameterValue.vi"("error in"=w1381, "Parameter Value"=w1380, "Parameter Name"=w1383, "connection ID in"=w1382) -> ("error out"=w1390:errorcluster, "connection ID out"=w1391:refnum<k5>)  [unwired: 3 in, 3 out]
            n671 = Add(x=w1387, y=w1388) -> (x+y=w1386:dbl)
            n672 = Subtract(x=w1388, y=w1387) -> (x-y=w1385:dbl)
            n673 = while {
              tunnel: w1391 -> [w1405]
              tunnel: w1390 -> [w1404]
              tunnel: [w1403] -> w1392
              tunnel: [w1402] -> w1384
              tunnel: w1383 -> [w1401]
              tunnel: w1386 -> [w1396]
              tunnel: w1385 -> [w1395]
              stop <- w1398 stop-if-true
              n674 = call "GetAnalyzerParameterValue.vi"("error in"=w1404, "Parameter Name"=w1401, "connection ID in"=w1405) -> ("error out"=w1402:errorcluster, "Parameter"=w1400:cluster{"Name":string, "Value":string}, "connection ID out"=w1403:refnum<k5>)  [unwired: 3 in, 3 out]
              n675 = Unbundle(w1400) -> ("Value"=w1399:string)  [unwired: 1 out]
              n676 = Fract/Exp String To Number(use system decimal point (T)=FALSE, string=w1399) -> (number=w1397:dbl)  [unwired: 2 in, 1 out]
              n677 = In Range and Coerce(upper limit=w1396, x=w1397, lower limit=w1395) -> (In Range?=w1398:bool)  [unwired: 1 out]
            }
          }
        }
        n678 = for {
          tunnel: w1348 -> [w1376]
          tunnel: w1347 -> [w1374]
          tunnel: w1346 -> [w1375] mode=indexing
          tunnel: [w1371] -> w1345 mode=indexing
          tunnel: [w1370] -> w1337
          tunnel: [w1369] -> w1336
          n679 = call "GetAnalyzerParameterValue.vi"("error in"=w1374, "Parameter Name"=w1375, "connection ID in"=w1376) -> ("error out"=w1369:errorcluster, "Parameter"=w1373:cluster{"Name":string, "Value":string}, "connection ID out"=w1370:refnum<k5>)  [unwired: 3 in, 3 out]
          n680 = Unbundle(w1373) -> ("Value"=w1372:string)  [unwired: 1 out]
          n681 = Fract/Exp String To Number(use system decimal point (T)=FALSE, string=w1372) -> (number=w1371:dbl)  [unwired: 2 in, 1 out]
        }
        n682 = Index Array(array=w1345) -> (element #1=w1344:dbl, element #2=w1343:dbl, element #3=w1342:dbl, element #4=w1341:dbl, element #5=w1340:dbl, element #6=w1339:dbl, element #7=w1338:dbl)  [unwired: 7 in]
        n683 = local write "phoib_I_3"(w1344) -> ()
        n684 = local write "phoib_I_5"(w1343) -> ()
        n685 = local write "phoib_I_6"(w1342) -> ()
        n686 = local write "phoib_I_8"(w1341) -> ()
        n687 = local write "phoib_I_9"(w1340) -> ()
        n688 = local write "phoib_I_10"(w1339) -> ()
        n689 = local write "phoib_I_7"(w1338) -> ()
        n690 = Send Notification(notification=w1350, notifier=w1365, error in (no error)=w1336) -> (error out=w1349:errorcluster)  [unwired: 1 out]
      }
      frame "standby" {
        n691 = Dequeue Element(queue=w1410) -> ()  [unwired: 2 in, 4 out]
        n692 = call "SetSafeState.vi"("error in"=w1408, "connection ID in"=w1409) -> ("error out"=w1406:errorcluster, "connection ID out"=w1407:refnum<k5>)  [unwired: 5 in, 3 out]
      }
      frame "release" {
        n693 = Dequeue Element(queue=w1419) -> (queue out=w1417:refnum<queue>)  [unwired: 2 in, 3 out]
        n694 = Enqueue Element(queue=w1417, element="suspend") -> ()  [unwired: 2 in, 3 out]
        n695 = flat-sequence {
          tunnel: w1416 -> [w1423]
          tunnel: w1415 -> [w1422]
          tunnel: [w1421] -> w1414
          tunnel: [w1420] -> w1411
          tunnel: w1414 -> [w1425]
          tunnel: [w1425] -> w1413
          tunnel: [w1424] -> w1412
          tunnel: w1411 -> [w1424]
          frame #0 {
            n696 = call "Disconnect.vi"("error in"=w1422, "connection ID in"=w1423) -> ("error out"=w1421:errorcluster, "connection ID out"=w1420:refnum<k5>)  [unwired: 5 in, 3 out]
          }
          frame #1 {
            n697 = local write "phoib_con?"(FALSE ("phoib_con?")) -> ()
          }
        }
      }
      frame "close" {
        n698 = Release Queue(queue=w1430) -> ()  [unwired: 2 in, 3 out]
      }
      frame "suspend" {
        n699 = Dequeue Element(queue=w1434) -> ()  [unwired: 2 in, 4 out]
      }
      frame "init" {
        n700 = Dequeue Element(queue=w1439) -> ()  [unwired: 2 in, 4 out]
        n701 = flat-sequence {
          tunnel: [w1445] -> w1438
          tunnel: [w1444] -> w1435
          tunnel: w1438 -> [w1458]
          tunnel: [w1458] -> w1437
          tunnel: [w1457] -> w1436
          tunnel: w1435 -> [w1457]
          frame #0 {
            n702 = local write "phoib_con?"(FALSE ("phoib_con?")) -> ()
          }
          frame #1 {
            n703 = TCP Open Connection(address="localhost", remote port or service name=u16 7010) -> (connection ID=w1450:refnum<k5>, error out=w1451:errorcluster)  [unwired: 3 in]
            n704 = call "Connect.vi"("error in"=w1451, "connection ID in"=w1450) -> ("error out"=w1453:errorcluster, "connection ID out"=w1452:refnum<k5>)  [unwired: 4 in, 4 out]
            n705 = call "GetSpectrumParameterInfo.vi"("error in"=w1453, "Parameter Name"="LensMode", "connection ID in"=w1452) -> ("error out"=w1455:errorcluster, "Spectrum Parameter Info"=w1443:T9, "connection ID out"=w1454:refnum<k5>)  [unwired: 3 in, 3 out]
            n706 = Unbundle By Name(w1443) -> ("Values"=w1442:string[])
            n707 = call "GetSpectrumParameterInfo.vi"("error in"=w1455, "Parameter Name"="ScanRange", "connection ID in"=w1454) -> ("error out"=w1444:errorcluster, "Spectrum Parameter Info"=w1456:T9, "connection ID out"=w1445:refnum<k5>)  [unwired: 3 in, 3 out]
            n708 = property on="lens_mode" class="CmbBox"("Strings[]"=w1442) -> ()  [unwired: 2 in, 2 out]
            n709 = Unbundle By Name(w1456) -> ("Values"=w1441:string[])
            n710 = property on="scan_range" class="CmbBox"("Strings[]"=w1441) -> ()  [unwired: 2 in, 2 out]
          }
          frame #2 {
            n711 = local write "phoib_con?"(TRUE ("phoib_con?")) -> ()
          }
        }
      }
    }
    "phoib_error" <- w1239
  }
  n712 = while {
    tunnel: w9 -> [w1469]
    tunnel: w8 -> [w1463]
    shift-right: [w1462] -> _
    shift-left: 0 -> [w1461]
    stop <- w1460 stop-if-true
    # "temp"
    n713 = Preview Queue Element(queue=w1469, timeout in ms (-1)=w1461) -> (queue out=w1464:refnum<queue>, element=w1468:string)  [unwired: 1 in, 2 out]
    n714 = Match Pattern(string=w1468, regular expression=":") -> (before substring=w1467:string, after substring=w1466:string)  [unwired: 1 in, 2 out]
    n715 = case shown="\"idle\", Default" w1467 {
      tunnel: w1466 -> [w1475 _ _ _ _]
      tunnel: w1464 -> [w1470 w1495 w1496 _ w1509]
      tunnel: w1463 -> [w1471 _ _ _ _]
      tunnel: [_ _ _ _ -1] -> w1462
      tunnel: [_ TRUE _ _ _] -> w1460
      frame "ramp" {
        n716 = Dequeue Element(queue=w1470) -> ()  [unwired: 2 in, 4 out]
        n717 = Match Pattern(string=w1475, regular expression=":") -> (before substring=w1474:string, after substring=w1478:string)  [unwired: 1 in, 2 out]
        n718 = Equal?(x=w1478, y="wait") -> (x = y?=w1472:bool)
        n719 = Scan From String(input string=w1474) -> (output 1=w1473:dbl)  [unwired: 4 in, 3 out]
        n720 = flat-sequence {
          tunnel: w1473 -> [w1480]
          tunnel: w1472 -> [w1482]
          tunnel: w1471 -> [w1492]
          frame #0 {
            n721 = local read "LS310  EPICS SP"() -> (w1479:string)
            n722 = call-poly <userlib>:"CaLabPut.vi"("Value"=w1480, "PV Name"=w1479) -> ()  [unwired: 6 in, 4 out]
          }
          frame #1 {
            n723 = Wait (ms)(milliseconds to wait=500) -> ()  [unwired: 1 out]
          }
          frame #2 {
            n724 = case shown="False" w1482 {
              frame False {
              }
              frame True {
                n725 = while {
                  stop <- w1488 stop-if-true
                  n726 = local read "Status EPICS chanel"() -> (w1490:string)
                  n727 = Wait (ms)(milliseconds to wait=500) -> ()  [unwired: 1 out]
                  n728 = call-poly <userlib>:"CaLabGet.vi"("PV Name"=w1490) -> ("1rst Value (string)"=w1491:string)  [unwired: 8 in, 6 out]
                  n729 = Equal?(x=w1491, y="Inside Range") -> (x = y?=w1488:bool)
                  n730 = local read "LS310  EPICS chanel A"() -> (w1484:string)
                  n731 = local read "LS310  EPICS chanel B"() -> (w1483:string)
                  n732 = call-poly <userlib>:"CaLabGet.vi"("PV Name"=w1484) -> ("1rst Value (number)"=w1485:dbl)  [unwired: 8 in, 6 out]
                  n733 = call-poly <userlib>:"CaLabGet.vi"("PV Name"=w1483) -> ("1rst Value (number)"=w1486:dbl)  [unwired: 8 in, 6 out]
                  n734 = local write "TB"(w1486) -> ()
                  n735 = local write "TA"(w1485) -> ()
                }
              }
            }
          }
          frame #3 {
            n736 = Send Notification(notification=TRUE, notifier=w1492) -> ()  [unwired: 1 in, 2 out]
          }
        }
      }
      frame "close" {
        n737 = Release Queue(queue=w1495) -> ()  [unwired: 2 in, 3 out]
      }
      frame "init" {
        n738 = Dequeue Element(queue=w1496) -> ()  [unwired: 2 in, 4 out]
      }
      frame "idle", Default {
        n739 = local read "LS310  EPICS chanel A"() -> (w1507:string)
        n740 = local read "LS310  EPICS chanel B"() -> (w1506:string)
        n741 = local read "LS310  EPICS SP"() -> (w1497:string)
        n742 = local read "Status EPICS chanel"() -> (w1505:string)
        n743 = local read "LS310  EPICS Heater"() -> (w1504:string)
        n744 = call-poly <userlib>:"CaLabGet.vi"("PV Name"=w1507) -> ("1rst Value (number)"=→"TA":dbl)  [unwired: 8 in, 6 out]
        n745 = call-poly <userlib>:"CaLabGet.vi"("PV Name"=w1506) -> ("1rst Value (number)"=→"TB":dbl)  [unwired: 8 in, 6 out]
        n746 = call-poly <userlib>:"CaLabGet.vi"("PV Name"=w1497) -> ("1rst Value (number)"=→"Readback":dbl)  [unwired: 8 in, 6 out]
        n747 = call-poly <userlib>:"CaLabGet.vi"("PV Name"=w1505) -> ("1rst Value (string)"=w1501:string)  [unwired: 8 in, 6 out]
        n748 = call-poly <userlib>:"CaLabGet.vi"("PV Name"=w1504) -> ()  [unwired: 8 in, 7 out]
        n749 = Equal?(x=w1501, y="Inside Range") -> (x = y?=→"In Range":bool)
      }
      frame "suspend" {
        n750 = Dequeue Element(queue=w1509) -> ()  [unwired: 2 in, 4 out]
      }
    }
  }
  n751 = while {
    tunnel: w3 -> [w1519]
    tunnel: w8 -> [w1513]
    shift-right: [w1512] -> _
    shift-left: _ -> [w1511]
    stop <- w1510 stop-if-true
    # "temp"
    n752 = Preview Queue Element(queue=w1519, timeout in ms (-1)=w1511) -> (queue out=w1514:refnum<queue>, element=w1518:string)  [unwired: 1 in, 2 out]
    n753 = Match Pattern(string=w1518, regular expression=":") -> (before substring=w1517:string, after substring=w1516:string)  [unwired: 1 in, 2 out]
    n754 = case shown="\"abs\"" w1517 {
      tunnel: w1516 -> [w1526 _ _ _ _]
      tunnel: w1514 -> [w1521 w1546 w1547 _ w1551]
      tunnel: w1513 -> [w1522 _ _ _ _]
      tunnel: [_ _ _ _ -1] -> w1512
      tunnel: [_ TRUE _ _ _] -> w1510
      frame "abs" {
        n755 = Dequeue Element(queue=w1521) -> ()  [unwired: 2 in, 4 out]
        n756 = Match Pattern(string=w1526, regular expression=":") -> (before substring=w1525:string, after substring=w1529:string)  [unwired: 1 in, 2 out]
        n757 = Equal?(x=w1529, y="wait") -> (x = y?=w1523:bool)
        n758 = Scan From String(input string=w1525) -> (output 1=w1524:dbl)  [unwired: 4 in, 3 out]
        n759 = flat-sequence {
          tunnel: w1524 -> [w1530]
          tunnel: [w1530] -> w1520
          tunnel: w1523 -> [w1533]
          tunnel: w1520 -> [w1532]
          tunnel: w1522 -> [w1543]
          frame #0 {
            n760 = local read "WattPilot EPICS chanel set"() -> (w1531:string)
            n761 = call-poly <userlib>:"CaLabPut.vi"("Value"=w1530, "PV Name"=w1531) -> ()  [unwired: 6 in, 4 out]
          }
          frame #1 {
            n762 = case shown="False" w1533 {
              tunnel: w1532 -> [_ w1534]
              frame False {
              }
              frame True {
                n763 = while {
                  tunnel: w1534 -> [w1539]
                  stop <- w1536 stop-if-true
                  n764 = local read "WattPilot EPICS chanel readback"() -> (w1541:string)
                  n765 = Wait (ms)(milliseconds to wait=500) -> ()  [unwired: 1 out]
                  n766 = call-poly <userlib>:"CaLabGet.vi"("PV Name"=w1541) -> ("1rst Value (number)"=w1540:dbl)  [unwired: 8 in, 6 out]
                  n767 = Subtract(x=w1540, y=w1539) -> (x-y=w1538:dbl)
                  n768 = Absolute Value(x=w1538) -> (abs(x)=w1537:dbl)
                  n769 = local write "Readback_wattpilot"(w1540) -> ()
                  n770 = Less?(x=w1537, y=0.1) -> (x < y?=w1536:bool)
                }
              }
            }
          }
          frame #2 {
            n771 = Send Notification(notification=TRUE, notifier=w1543) -> ()  [unwired: 1 in, 2 out]
          }
        }
      }
      frame "close" {
        n772 = Release Queue(queue=w1546) -> ()  [unwired: 2 in, 3 out]
      }
      frame "init" {
        n773 = Dequeue Element(queue=w1547) -> ()  [unwired: 2 in, 4 out]
      }
      frame "idle", Default {
        n774 = local read "WattPilot EPICS chanel readback"() -> (w1549:string)
        n775 = call-poly <userlib>:"CaLabGet.vi"("PV Name"=w1549) -> ("1rst Value (number)"=→"Readback_wattpilot":dbl)  [unwired: 8 in, 6 out]
      }
      frame "suspend" {
        n776 = Dequeue Element(queue=w1551) -> ()  [unwired: 2 in, 4 out]
      }
    }
  }
  n777 = while {
    tunnel: w24 -> [w1578]
    shift-right: [w1572] -> _
    shift-left: _ -> [w1571]
    shift-right: [w1570] -> _
    shift-left: _ -> [w1568]
    shift-right: [w1569] -> _
    shift-left: _ -> [w1567]
    shift-right: [w1564] -> _
    shift-left: 0 -> [w1565]
    shift-right: [w1563] -> _
    shift-left: _ -> [w1562]
    shift-right: [w1561] -> _
    shift-left: _ -> [w1560]
    tunnel: w33 -> [w1559]
    shift-right: [w1558] -> _
    shift-left: _ -> [w1557]
    shift-right: [w1555] -> _
    shift-left: _ -> [w1554]
    shift-right: [w1553] -> _
    shift-left: _ -> [w1552]
    i -> [w1556]
    stop <- w1566 stop-if-true
    # "cam"
    n778 = Preview Queue Element(queue=w1578, timeout in ms (-1)=w1565) -> (queue out=w1577:refnum<queue>, element=w1576:string)  [unwired: 1 in, 2 out]
    n779 = Match Pattern(string=w1576, regular expression=":") -> (before substring=w1573:string, after substring=w1574:string)  [unwired: 1 in, 2 out]
    n780 = case shown="\"idle\", Default" w1573 {
      tunnel: w1577 -> [w1590 w1622 w1655 w1668 _ w1756 w1786 w1851]
      tunnel: w1574 -> [_ _ _ _ _ _ _ _]
      tunnel: [w1584 w1609 w1654 w1666 w1709 w1753 w1771 w1849] -> w1572
      tunnel: w1571 -> [_ _ w1654 w1666 w1709 w1753 w1771 w1849]
      tunnel: [w1589 w1623 u64 0 ("Hout") w1665 w1713 w1754 w1781 w1848] -> w1570
      tunnel: [w1591 w1624 w1651 w1664 w1714 w1755 w1772 w1847] -> w1569
      tunnel: w1568 -> [_ w1626 w1653 w1665 w1716 w1758 w1783 w1848]
      tunnel: w1567 -> [_ w1625 _ w1664 w1715 w1757 w1782 w1847]
      tunnel: [_ _ _ TRUE _ _ _ _] -> w1566
      tunnel: [_ _ -1 _ _ _ _ -1] -> w1564
      tunnel: [w1583 w1610 _ _ w1723 _ _ _] -> w1563
      tunnel: w1562 -> [w1583 w1610 _ _ w1722 _ _ _]
      tunnel: [w1584 w1612 w1649 w1663 w1718 w1747 w1784 w1846] -> w1561
      tunnel: w1560 -> [_ w1612 w1649 w1663 w1718 _ w1784 w1846]
      tunnel: w1559 -> [_ _ _ _ _ _ w1775 _]
      tunnel: [w1581 w1607 w1648 w1661 w1676 w1744 w1778 w1845] -> w1558
      tunnel: w1557 -> [w1581 w1607 w1648 w1661 w1711 w1744 w1778 w1845]
      tunnel: w1556 -> [_ _ _ _ w1684 _ _ _]
      tunnel: [w1582 w1608 w1647 w1662 w1710 w1743 w1777 w1844] -> w1555
      tunnel: w1554 -> [w1582 w1608 w1647 w1662 w1683 w1743 w1777 w1844]
      tunnel: [w1580 w1604 refnum<k21> refnum ("task out") w1660 w1669 w1742 w1768 w1843] -> w1553
      tunnel: w1552 -> [_ w1604 w1646 w1660 w1669 w1742 w1769 w1843]
      frame "init" {
        w1584 = u16[][] []
        n781 = flat-sequence {
          tunnel: [w1593] -> w1588
          tunnel: [w1594] -> w1587
          tunnel: [w1602] -> w1589
          tunnel: [w1603] -> w1591
          tunnel: w1588 -> [w1603]
          tunnel: w1587 -> [w1602]
          frame #0 {
            n782 = local write "cam_con?"(FALSE ("cam_con?")) -> ()
          }
          frame #1 {
            n783 = call "SCInitBoard.vi"("boardnr"="board number") -> ("Hout"=w1597:u32, "error out"=w1598:errorcluster)  [unwired: 1 in, 1 out]
            n784 = call "SCSetupCamera.vi"("Handle"=w1597, "error in (no error)"=w1598) -> ("Hout"=w1599:u64, "error out"=w1600:errorcluster)  [unwired: 1 out]
            n785 = call "SCStopCOC.vi"("error in (no error)"=w1600, "Stop mode"=0, "Handle"=w1599) -> ("error out"=w1593:errorcluster, "Hout"=w1594:u64)
          }
          frame #2 {
            n786 = local write "cam_con?"(TRUE ("cam_con?")) -> ()
          }
        }
        n787 = Dequeue Element(queue=w1590) -> (queue out=w1586:refnum<queue>)  [unwired: 2 in, 3 out]
        n788 = Enqueue Element At Opposite End(queue=w1586, element="set") -> ()  [unwired: 2 in, 3 out]
        n789 = call-poly <vilib>:"DAQmx Create Virtual Channel.vi"("lines"=tag "Dev1/port0/line0") -> ("task out"=w1580:refnum<k21>)  [unwired: 13 in, 1 out]
      }
      frame "set" {
        n790 = Dequeue Element(queue=w1622) -> ()  [unwired: 2 in, 4 out]
        n791 = call "SCStopCOC.vi"("error in (no error)"=w1625, "Stop mode"=0, "Handle"=w1626) -> ("error out"=w1641:errorcluster, "Hout"=w1640:u64)
        n792 = Bundle By Name(cluster=cluster{"Delay":dbl, "Exposure ":dbl} {"Delay"=0.0, "Exposure "=0.0} ("Delay and exposure"), "Exposure"="cam_exp") -> (w1619:cluster{"Delay":dbl, "Exposure ":dbl})
        n793 = Bundle By Name(cluster=T10 {"Camera type"=0, "Operating mode\nHP & QE / HS & DiCam Pro "=0, "Frame trigger \n(High Performance and QE only)"=0, "Sequence trigger"=0, "Low Light\n(QE only)"=FALSE, "Gain"=FALSE, "Horzontal\nbinning"=0, "Vertical\nbinning "=0, "ROI Left"=1, "ROI Right"=20, "ROI Top"=1, "ROI Bottom"=15} ("Camera controls"), "Operating mode\nHP & QE / HS & DiCam Pro"="Operating mode\nHP & QE / HS & DiCam Pro", "Horzontal\nbinning"="binning", "Vertical\nbinning"="binning", "ROI Left"="ROI Left", "ROI Right"="ROI Right", "ROI Top"="ROI Top", "ROI Bottom"="ROI Bottom", "Gain"="gain", "Frame trigger \n(High Performance and QE only)"="Frame trigger \n(High Performance and QE only)") -> (w1636:T10)
        n794 = call "New delay and exposure forma.vi"("Operating mode\nHP & QE / HS & DiCam Pro"="Operating mode\nHP & QE / HS & DiCam Pro", "Delay and exposure"=w1619) -> ("Output table"=w1637:string)  [unwired: 3 in]
        n795 = call "SCSetCoC.vi"("error in (no error)"=w1641, "Delay and exposure table"=w1637, "Camera controls"=w1636, "Handle"=w1640) -> ("error out"=w1629:errorcluster, "Hout"=w1628:u64)  [unwired: 1 out]
        n796 = call "SCGetImageSize.vi"("Handle"=w1628, "error in (no error)"=w1629) -> ("Hout"=w1627:u64, "error out"=w1611:errorcluster, "Horizontal size"=w1616:i32, "Vertical size"=w1615:i32)  [unwired: 2 out]
        n797 = Greater?(x=w1616, y=w1615) -> (0:w1617:bool)
        n798 = Initialize Array(u16 0 ("dimension size"), w1615, w1616) -> (w1609:u16[][])
        n799 = call "SCRun.vi"("error in (no error)"=w1611, "Run mode"=0, "Handle"=w1627) -> ("error out"=w1624:errorcluster, "Hout"=w1623:u64)  [unwired: 1 out]
        n800 = Select(t=w1616, s=w1617, f=w1615) -> (s? t:f=w1614:i32)
        n801 = property on="mainimg" class="IntGraph (strict)"("XScale.Maximum"=w1614, "YScale.Maximum"=w1614) -> ()  [unwired: 2 in, 2 out]
      }
      frame "release" {
        n802 = Dequeue Element(queue=w1655) -> (queue out=w1642:refnum<queue>)  [unwired: 2 in, 3 out]
        n803 = flat-sequence {
          tunnel: w1653 -> [w1657]
          tunnel: [w1656] -> w1650
          tunnel: [w1659] -> w1651
          tunnel: w1650 -> [w1659]
          frame #0 {
            n804 = call "SCCloseBoard.vi"("Handle"=w1657) -> ("error out"=w1656:errorcluster)  [unwired: 1 in, 2 out]
          }
          frame #1 {
            n805 = local write "cam_con?"(FALSE ("cam_con?")) -> ()
          }
        }
        n806 = Enqueue Element(queue=w1642, element="suspend") -> ()  [unwired: 2 in, 3 out]
        n807 = call <vilib>:"DAQmx Clear Task.vi"("task in"=w1646) -> ()  [unwired: 14 in, 1 out]
      }
      frame "close" {
        n808 = Release Queue(queue=w1668) -> ()  [unwired: 2 in, 3 out]
      }
      frame "idle", Default {
        n809 = call "grabimg.vi"("array in"=w1709, "error in"=w1715, "Hin"=w1716) -> ("error out"=w1714:errorcluster, "imgdata"=w1712:i32[][], "Hout"=w1713:u64)  [unwired: 6 in]
        n810 = local read "lower threshold"() -> (w1707:i32)
        n811 = case shown="True" "cam_dark?" {
          tunnel: w1718 -> [_ w1741]
          tunnel: [w1738 w1740] -> w1708
          tunnel: w1712 -> [w1738 w1739]
          frame False {
          }
          frame True {
            n812 = Subtract(x=w1739, y=w1741) -> (x-y=w1740:dbl[][])
          }
        }
        n813 = call "filtr_b.vi"("threshold"=w1707, "input array"=w1708) -> ("output array"=w1699:dbl[][])  [unwired: 9 in]
        n814 = call <vilib>:"High Resolution Relative Seconds.vi"() -> ("relative seconds"=w1723:dbl)
        n815 = Subtract(x=w1723, y=w1722) -> (x-y=w1721:dbl)
        n816 = Array Size(array=w1699) -> (size(s)=w1698:i32[])
        n817 = Reciprocal(x=w1721) -> (1/x=→"cam_fps":dbl)
        n818 = Index Array(array=w1698) -> (element #1=w1693:i32, element #2=w1692:i32)  [unwired: 2 in]
        n819 = Subtract(x=w1684, y=w1683) -> (x-y=w1682:i32)
        n820 = Less Or Equal?(x="pics2avg", y=w1682) -> (x <= y?=w1705:bool)
        n821 = And(x="reset every n pics", y=w1705) -> (x .and. y?=w1703:bool)
        n822 = Not(x=w1703) -> (.not. x?=w1702:bool)
        n823 = call-poly <vilib>:"Ramp Pattern.vi"("start"=0.0, "end"=w1693, "samples"=w1693) -> ("Ramp Pattern"=w1688:dbl[])  [unwired: 7 in, 1 out]
        n824 = call-poly <vilib>:"Ramp Pattern.vi"("start"=0.0, "end"=w1692, "samples"=w1692) -> ("Ramp Pattern"=w1689:dbl[])  [unwired: 7 in, 1 out]
        n825 = property on="mainimg" class="IntGraph (strict)"() -> ("CrsrLis"=w1681:T3)  [unwired: 2 in, 2 out]
        n826 = And(x="cam_liveavg", y=w1702) -> (x .and. y?=w1700:bool)
        n827 = case shown="False" w1700 {
          tunnel: w1699 -> [w1728 w1734]
          tunnel: [w1728 w1731] -> w1676
          tunnel: w1711 -> [_ w1736]
          tunnel: w1684 -> [w1729 _]
          tunnel: [w1729 w1737] -> w1710
          tunnel: w1683 -> [_ w1737]
          tunnel: w1682 -> [_ w1730]
          frame False {
          }
          frame True {
            n828 = Multiply(x=w1736, y=w1730) -> (x*y=w1735:dbl[][])
            n829 = Increment(x=w1730) -> (x+1=w1732:i32)
            n830 = Add(x=w1735, y=w1734) -> (x+y=w1733:dbl[][])
            n831 = Divide(x=w1733, y=w1732) -> (x/y=w1731:dbl[][])
          }
        }
        "mainimg" <- w1676
        n832 = Index Array(array=w1681) -> (element #1=w1679:T11, element #2=w1680:T11)  [unwired: 2 in]
        n833 = Unbundle By Name(w1679) -> ("Position.X"=w1673:dbl, "Position.Y"=w1675:dbl)
        n834 = Unbundle By Name(w1680) -> ("Position.X"=w1677:dbl, "Position.Y"=w1678:dbl)
        n835 = Array Max & Min(array=w1676) -> (max value=→"max":dbl)  [unwired: 3 out]
        n836 = Subtract(x=w1678, y=w1675) -> (x-y=w1674:dbl)
        n837 = Subtract(x=w1677, y=w1673) -> (x-y=w1672:dbl)
        n838 = Array Subset(array=w1676, index (row)=w1675, length (row)=w1674) -> (w1687:dbl[][])  [unwired: 2 in]
        n839 = Array Subset(array=w1676, index (col)=w1673, length (col)=w1672) -> (w1685:dbl[][])  [unwired: 2 in]
        n840 = Array Subset(array=w1676, index (row)=w1675, length (row)=w1674, index (col)=w1673, length (col)=w1672) -> (w1671:dbl[][])
        n841 = Transpose 2D Array(2D array=w1687) -> (transposed array=w1686:dbl[][])
        n842 = Add Array Elements(numeric array=w1671) -> (sum=→"sum" →"Waveform Chart":dbl)
        n843 = for {
          tunnel: w1685 -> [w1725] mode=indexing
          tunnel: [w1724] -> w1695 mode=indexing
          n844 = Add Array Elements(numeric array=w1725) -> (sum=w1724:dbl)
        }
        n845 = for {
          tunnel: w1686 -> [w1727] mode=indexing
          tunnel: [w1726] -> w1694 mode=indexing
          n846 = Add Array Elements(numeric array=w1727) -> (sum=w1726:dbl)
        }
        n847 = Bundle("Ramp Pattern"=w1689, w1694) -> (→"G2 X":cluster{"Ramp Pattern":dbl[], dbl[]})  [unwired: 1 in]
        n848 = Bundle(w1695, "Ramp Pattern"=w1688) -> (→"G2 Y":cluster{dbl[], "Ramp Pattern":dbl[]})  [unwired: 1 in]
      }
      frame "dark" {
        n849 = Dequeue Element(queue=w1756) -> ()  [unwired: 2 in, 4 out]
        n850 = Array Size(array=w1753) -> (size(s)=w1752:i32[])
        n851 = Index Array(array=w1752) -> (element #1=w1751:i32, element #2=w1750:i32)  [unwired: 2 in]
        n852 = Initialize Array(0.0 ("element"), w1751, w1750) -> (w1748:dbl[][])
        n853 = for {
          N: "dark avg" -> [_]
          tunnel: w1758 -> [w1766]
          tunnel: w1757 -> [w1765]
          tunnel: [w1764] -> w1755
          tunnel: w1753 -> [w1763]
          tunnel: [w1762] -> w1754
          shift-right: [w1759] -> w1746
          shift-left: w1748 -> [w1760]
          n854 = call "grabimg.vi"("array in"=w1763, "error in"=w1765, "Hin"=w1766) -> ("error out"=w1764:errorcluster, "imgdata"=w1761:i32[][], "Hout"=w1762:u64)  [unwired: 6 in]
          n855 = Add(x=w1761, y=w1760) -> (x+y=w1759:dbl[][])
        }
        n856 = Divide(x=w1746, y="dark avg") -> (x/y=w1747:dbl[][])
      }
      frame "snap" {
        n857 = Dequeue Element(queue=w1786) -> ()  [unwired: 2 in, 4 out]
        n858 = local read "cam_dark?"() -> (w1785:bool)
        n859 = local read "cam_avgs"() -> (w1780:i32)
        n860 = To Double Precision Float(number=w1771) -> (double precision float=w1770:dbl[][])
        n861 = Equal To 0?(x="aq.mode") -> (x = 0?=w1773:bool)
        n862 = Get Date/Time In Seconds() -> (seconds since 1Jan1904=w1776:timestamp)
        n863 = for {
          N: w1780 -> [w1798]
          shift-right: [w1815] -> w1781
          shift-left: w1783 -> [w1817]
          shift-right: [w1803] -> w1779
          shift-left: w1782 -> [w1816]
          tunnel: w1785 -> [w1813]
          tunnel: w1784 -> [w1812]
          tunnel: w1771 -> [w1811]
          tunnel: w1776 -> [w1807]
          tunnel: w1773 -> [w1791]
          shift-right: [w1799] -> w1767
          shift-left: w1770 -> [w1800]
          shift-right: [w1789] -> w1768
          shift-left: w1769 -> [w1789]
          i -> [w1787]
          stop <- "abort acq." stop-if-true
          n864 = call "grabimg.vi"("array in"=w1811, "error in"=w1816, "Hin"=w1817) -> ("error out"=w1803:errorcluster, "imgdata"=w1814:i32[][], "Hout"=w1815:u64)  [unwired: 6 in]
          n865 = local read "lower threshold"() -> (w1794:i32)
          n866 = Increment(x=w1787) -> (x+1=w1796:i32)
          "acq. imgs" <- w1796
          n867 = Get Date/Time In Seconds() -> (seconds since 1Jan1904=w1810:timestamp)
          n868 = case shown="True" w1813 {
            tunnel: w1814 -> [w1839 w1842]
            tunnel: w1812 -> [_ w1841]
            tunnel: [w1839 w1840] -> w1793
            frame False {
            }
            frame True {
              n869 = Subtract(x=w1842, y=w1841) -> (x-y=w1840:dbl[][])
            }
          }
          n870 = Divide(x=w1796, y=w1798) -> (x/y=→"snap_prog":dbl)
          n871 = Subtract(x=w1810, y=w1807) -> (x-y=w1809:dbl)
          n872 = call "filtr_b.vi"("threshold"=w1794, "input array"=w1793) -> ("output array"=w1792:dbl[][])  [unwired: 9 in]
          n873 = Divide(x=w1809, y=w1787) -> (x/y=w1805:dbl)
          n874 = Multiply(x=w1805, y=w1798) -> (x*y=w1808:dbl)
          n875 = Reciprocal(x=w1805) -> (1/x=w1804:dbl)
          n876 = case shown="True" "count?" {
            tunnel: w1792 -> [w1830 w1832]
            tunnel: "e-size" -> [_ w1834]
            tunnel: w1794 -> [_ w1833]
            tunnel: [w1830 w1831] -> w1790
            frame False {
            }
            frame True {
              n877 = Array Size(array=w1832) -> (size(s)=w1836:i32[])
              n878 = call "findr.vi"("thresh"=w1833, "esize"=w1834, "inp array"=w1832) -> ("locs"=w1835:i32[][])  [unwired: 8 in]
              n879 = Index Array(array=w1836) -> (element #1=w1838:i32, element #2=w1837:i32)  [unwired: 2 in]
              n880 = call "drawe.vi"("Ysize"=w1838, "Xsize"=w1837, "pos array"=w1835) -> ("img out"=w1831:i32[][])  [unwired: 8 in]
            }
          }
          n881 = Add(x=w1808, y=w1807) -> (x+y=→"ETA":timestamp)
          n882 = local write "cam_fps"(w1804) -> ()
          n883 = local write "mainimg"(w1792) -> ()
          n884 = case shown="True" w1791 {
            tunnel: w1790 -> [w1820 w1828]
            tunnel: w1800 -> [w1822 w1827]
            tunnel: [w1821 w1825] -> w1799
            tunnel: [w1819 w1824] -> w1788
            tunnel: w1787 -> [w1818 w1823]
            frame False {
              n885 = Add(x=w1820, y=w1822) -> (x+y=w1821:dbl[][])
              n886 = Increment(x=w1818) -> (x+1=w1819:i32)
            }
            frame True {
              n887 = Multiply(x=w1827, y=w1823) -> (x*y=w1829:dbl[][])
              n888 = Increment(x=w1823) -> (x+1=w1824:i32)
              n889 = Add(x=w1828, y=w1829) -> (x+y=w1826:dbl[][])
              n890 = Divide(x=w1826, y=w1824) -> (x/y=w1825:dbl[][])
            }
          }
          "Pics L" <- w1788
          n891 = local write "sideimg"(w1799) -> ()
        }
        n892 = Enqueue Element(queue=w1775, element=w1767, error in (no error)=w1779) -> (error out=w1772:errorcluster)  [unwired: 1 in, 2 out]
      }
      frame "suspend" {
        n893 = Dequeue Element(queue=w1851) -> ()  [unwired: 2 in, 4 out]
      }
    }
    "cam_error" <- w1569
  }
